vi "RTS Door Opener Setup.vi"(8 "Error In":errorcluster, 11 "Station Settings":T1) -> (0 "Error Out":errorcluster, 3 "Update Server Output":bool)   [LabVIEW 2020]
uses:
  Type Definitions/RTS Door Op Data.ctl
  Type Definitions/RTS Door Ops Client.ctl
  Type Definitions/RTS Door Opening Schedule.ctl
  Type Definitions/RTS Door Ops Sequence.ctl
  Type Definitions/RTS Standard Door Opening Test.ctl
  Type Definitions/RTS Station Settions TCP Comms.ctl
  Type Definitions/RTS Chamber Save Status.ctl
  Type Definitions/RTS Test Pattern.ctl
panel:
  out "Front Program Name":string
  in  "Update Server":bool
  in  "Tab Control 2":enum32{"Page 1", "Standard Test"}(tab)
  out "time stamp":timestamp
  out "Station":u16
  out "Chamber":u16
  out "Debug array":string[](array[string])
  in  "Debug":bool
  in  "ISO Energy Consumption":T4={"Chamber 1-3"=[], "Chamber 1-2"=[], "Chamber 1-1"=[{"End Time"=timestamp(0 s since 1904-01-01), "Start Time"=timestamp(0 s since 1904-01-01), "Door Opening Schedule:"={"Open Door Timer (s)"=0.0, "Delay Time (s)"=0.0, "Close Door Timer (s)"=0.0}, "Enable Door Ops"=FALSE, "Door Openings"=0, "Temp (°F)"=90.0, "Humidity (%)"=40.0, "Voltage (V)"=0.0, "Door Open Sequence:"=enum."", "Door Delay(sec)"=0.0, "Dehum (°F)"=0.0, "Cool (°F)"=0.0}], "Standard Tests 1-1"=enum."511-B304 ISO Energy Consumption"} {"Chamber 1-1"."Start Time" format="%<%X\n%x>T"; "Chamber 1-1"."End Time" format="%<%X\n%x>T"; "Chamber 1-2"."Start Time" format="%<%X\n%x>T"; "Chamber 1-2"."End Time" format="%<%X\n%x>T"; "Chamber 1-3"."Start Time" format="%<%X\n%x>T"; "Chamber 1-3"."End Time" format="%<%X\n%x>T"}
  in  "NDO":T4={"Chamber 1-3"=[], "Chamber 1-2"=[], "Chamber 1-1"=[{"End Time"=timestamp(0 s since 1904-01-01), "Start Time"=timestamp(0 s since 1904-01-01), "Door Opening Schedule:"={"Open Door Timer (s)"=0.0, "Delay Time (s)"=0.0, "Close Door Timer (s)"=0.0}, "Enable Door Ops"=FALSE, "Door Openings"=0, "Temp (°F)"=90.0, "Humidity (%)"=50.0, "Voltage (V)"=0.0, "Door Open Sequence:"=enum."", "Door Delay(sec)"=0.0, "Dehum (°F)"=0.0, "Cool (°F)"=0.0}], "Standard Tests 1-1"=enum."511-B100 No Door Opening (NDO)"} {"Chamber 1-1"."Start Time" format="%<%X\n%x>T"; "Chamber 1-1"."End Time" format="%<%X\n%x>T"; "Chamber 1-2"."Start Time" format="%<%X\n%x>T"; "Chamber 1-2"."End Time" format="%<%X\n%x>T"; "Chamber 1-3"."Start Time" format="%<%X\n%x>T"; "Chamber 1-3"."End Time" format="%<%X\n%x>T"}
  in  "Moisture Accumulation (511-C401)":T4={"Chamber 1-3"=[{"End Time"=timestamp(0 s since 1904-01-01), "Start Time"=timestamp(0 s since 1904-01-01), "Door Opening Schedule:"={"Open Door Timer (s)"=0.0, "Delay Time (s)"=0.0, "Close Door Timer (s)"=0.0}, "Enable Door Ops"=FALSE, "Door Openings"=0, "Temp (°F)"=78.0, "Humidity (%)"=83.0, "Voltage (V)"=120.0, "Door Open Sequence:"=enum."", "Door Delay(sec)"=0.0, "Dehum (°F)"=70.0, "Cool (°F)"=65.0}, {"End Time"=timestamp(0 s since 1904-01-01), "Start Time"=timestamp(0 s since 1904-01-01), "Door Opening Schedule:"={"Open Door Timer (s)"=6.0, "Delay Time (s)"=465.0, "Close Door Timer (s)"=6.0}, "Enable Door Ops"=TRUE, "Door Openings"=0, "Temp (°F)"=90.0, "Humidity (%)"=65.0, "Voltage (V)"=120.0, "Door Open Sequence:"=enum."", "Door Delay(sec)"=0.0, "Dehum (°F)"=84.0, "Cool (°F)"=85.0}, {"End Time"=timestamp(0 s since 1904-01-01), "Start Time"=timestamp(0 s since 1904-01-01), "Door Opening Schedule:"={"Open Door Timer (s)"=6.0, "Delay Time (s)"=465.0, "Close Door Timer (s)"=6.0}, "Enable Door Ops"=TRUE, "Door Openings"=0, "Temp (°F)"=78.0, "Humidity (%)"=83.0, "Voltage (V)"=120.0, "Door Open Sequence:"=enum."", "Door Delay(sec)"=0.0, "Dehum (°F)"=70.0, "Cool (°F)"=65.0}, {"End Time"=timestamp(0 s since 1904-01-01), "Start Time"=timestamp(0 s since 1904-01-01), "Door Opening Schedule:"={"Open Door Timer (s)"=0.0, "Delay Time (s)"=0.0, "Close Door Timer (s)"=0.0}, "Enable Door Ops"=FALSE, "Door Openings"=0, "Temp (°F)"=78.0, "Humidity (%)"=83.0, "Voltage (V)"=120.0, "Door Open Sequence:"=enum."", "Door Delay(sec)"=0.0, "Dehum (°F)"=70.0, "Cool (°F)"=65.0}, {"End Time"=timestamp(0 s since 1904-01-01), "Start Time"=timestamp(0 s since 1904-01-01), "Door Opening Schedule:"={"Open Door Timer (s)"=6.0, "Delay Time (s)"=465.0, "Close Door Timer (s)"=6.0}, "Enable Door Ops"=TRUE, "Door Openings"=0, "Temp (°F)"=90.0, "Humidity (%)"=65.0, "Voltage (V)"=120.0, "Door Open Sequence:"=enum."", "Door Delay(sec)"=0.0, "Dehum (°F)"=84.0, "Cool (°F)"=85.0}, {"End Time"=timestamp(0 s since 1904-01-01), "Start Time"=timestamp(0 s since 1904-01-01), "Door Opening Schedule:"={"Open Door Timer (s)"=6.0, "Delay Time (s)"=465.0, "Close Door Timer (s)"=6.0}, "Enable Door Ops"=TRUE, "Door Openings"=0, "Temp (°F)"=78.0, "Humidity (%)"=83.0, "Voltage (V)"=120.0, "Door Open Sequence:"=enum."", "Door Delay(sec)"=0.0, "Dehum (°F)"=70.0, "Cool (°F)"=65.0}, {"End Time"=timestamp(0 s since 1904-01-01), "Start Time"=timestamp(0 s since 1904-01-01), "Door Opening Schedule:"={"Open Door Timer (s)"=0.0, "Delay Time (s)"=0.0, "Close Door Timer (s)"=0.0}, "Enable Door Ops"=FALSE, "Door Openings"=0, "Temp (°F)"=78.0, "Humidity (%)"=83.0, "Voltage (V)"=120.0, "Door Open Sequence:"=enum."", "Door Delay(sec)"=0.0, "Dehum (°F)"=70.0, "Cool (°F)"=65.0}], "Chamber 1-2"=[{"End Time"=timestamp(0 s since 1904-01-01), "Start Time"=timestamp(0 s since 1904-01-01), "Door Opening Schedule:"={"Open Door Timer (s)"=0.0, "Delay Time (s)"=0.0, "Close Door Timer (s)"=0.0}, "Enable Door Ops"=FALSE, "Door Openings"=0, "Temp (°F)"=78.0, "Humidity (%)"=83.0, "Voltage (V)"=120.0, "Door Open Sequence:"=enum."", "Door Delay(sec)"=0.0, "Dehum (°F)"=70.0, "Cool (°F)"=65.0}, {"End Time"=timestamp(0 s since 1904-01-01), "Start Time"=timestamp(0 s since 1904-01-01), "Door Opening Schedule:"={"Open Door Timer (s)"=6.0, "Delay Time (s)"=465.0, "Close Door Timer (s)"=6.0}, "Enable Door Ops"=TRUE, "Door Openings"=0, "Temp (°F)"=90.0, "Humidity (%)"=65.0, "Voltage (V)"=120.0, "Door Open Sequence:"=enum."", "Door Delay(sec)"=0.0, "Dehum (°F)"=0.0, "Cool (°F)"=0.0}, {"End Time"=timestamp(0 s since 1904-01-01), "Start Time"=timestamp(0 s since 1904-01-01), "Door Opening Schedule:"={"Open Door Timer (s)"=6.0, "Delay Time (s)"=465.0, "Close Door Timer (s)"=6.0}, "Enable Door Ops"=TRUE, "Door Openings"=0, "Temp (°F)"=78.0, "Humidity (%)"=83.0, "Voltage (V)"=120.0, "Door Open Sequence:"=enum."", "Door Delay(sec)"=0.0, "Dehum (°F)"=70.0, "Cool (°F)"=65.0}, {"End Time"=timestamp(0 s since 1904-01-01), "Start Time"=timestamp(0 s since 1904-01-01), "Door Opening Schedule:"={"Open Door Timer (s)"=0.0, "Delay Time (s)"=0.0, "Close Door Timer (s)"=0.0}, "Enable Door Ops"=FALSE, "Door Openings"=0, "Temp (°F)"=78.0, "Humidity (%)"=83.0, "Voltage (V)"=120.0, "Door Open Sequence:"=enum."", "Door Delay(sec)"=0.0, "Dehum (°F)"=70.0, "Cool (°F)"=65.0}, {"End Time"=timestamp(0 s since 1904-01-01), "Start Time"=timestamp(0 s since 1904-01-01), "Door Opening Schedule:"={"Open Door Timer (s)"=6.0, "Delay Time (s)"=465.0, "Close Door Timer (s)"=6.0}, "Enable Door Ops"=TRUE, "Door Openings"=0, "Temp (°F)"=90.0, "Humidity (%)"=65.0, "Voltage (V)"=120.0, "Door Open Sequence:"=enum."", "Door Delay(sec)"=0.0, "Dehum (°F)"=84.0, "Cool (°F)"=85.0}, {"End Time"=timestamp(0 s since 1904-01-01), "Start Time"=timestamp(0 s since 1904-01-01), "Door Opening Schedule:"={"Open Door Timer (s)"=6.0, "Delay Time (s)"=465.0, "Close Door Timer (s)"=6.0}, "Enable Door Ops"=TRUE, "Door Openings"=0, "Temp (°F)"=78.0, "Humidity (%)"=83.0, "Voltage (V)"=120.0, "Door Open Sequence:"=enum."", "Door Delay(sec)"=0.0, "Dehum (°F)"=70.0, "Cool (°F)"=65.0}, {"End Time"=timestamp(0 s since 1904-01-01), "Start Time"=timestamp(0 s since 1904-01-01), "Door Opening Schedule:"={"Open Door Timer (s)"=0.0, "Delay Time (s)"=0.0, "Close Door Timer (s)"=0.0}, "Enable Door Ops"=FALSE, "Door Openings"=0, "Temp (°F)"=78.0, "Humidity (%)"=83.0, "Voltage (V)"=120.0, "Door Open Sequence:"=enum."", "Door Delay(sec)"=0.0, "Dehum (°F)"=70.0, "Cool (°F)"=65.0}], "Chamber 1-1"=[{"End Time"=timestamp(0 s since 1904-01-01), "Start Time"=timestamp(0 s since 1904-01-01), "Door Opening Schedule:"={"Open Door Timer (s)"=0.0, "Delay Time (s)"=0.0, "Close Door Timer (s)"=0.0}, "Enable Door Ops"=FALSE, "Door Openings"=0, "Temp (°F)"=78.0, "Humidity (%)"=83.0, "Voltage (V)"=120.0, "Door Open Sequence:"=enum."", "Door Delay(sec)"=0.0, "Dehum (°F)"=70.0, "Cool (°F)"=65.0}, {"End Time"=timestamp(0 s since 1904-01-01), "Start Time"=timestamp(0 s since 1904-01-01), "Door Opening Schedule:"={"Open Door Timer (s)"=6.0, "Delay Time (s)"=1850.0, "Close Door Timer (s)"=6.0}, "Enable Door Ops"=TRUE, "Door Openings"=0, "Temp (°F)"=90.0, "Humidity (%)"=65.0, "Voltage (V)"=120.0, "Door Open Sequence:"=enum."", "Door Delay(sec)"=0.0, "Dehum (°F)"=84.0, "Cool (°F)"=85.0}, {"End Time"=timestamp(0 s since 1904-01-01), "Start Time"=timestamp(0 s since 1904-01-01), "Door Opening Schedule:"={"Open Door Timer (s)"=6.0, "Delay Time (s)"=1850.0, "Close Door Timer (s)"=6.0}, "Enable Door Ops"=TRUE, "Door Openings"=0, "Temp (°F)"=78.0, "Humidity (%)"=83.0, "Voltage (V)"=120.0, "Door Open Sequence:"=enum."", "Door Delay(sec)"=0.0, "Dehum (°F)"=70.0, "Cool (°F)"=65.0}, {"End Time"=timestamp(0 s since 1904-01-01), "Start Time"=timestamp(0 s since 1904-01-01), "Door Opening Schedule:"={"Open Door Timer (s)"=0.0, "Delay Time (s)"=0.0, "Close Door Timer (s)"=0.0}, "Enable Door Ops"=FALSE, "Door Openings"=0, "Temp (°F)"=78.0, "Humidity (%)"=83.0, "Voltage (V)"=120.0, "Door Open Sequence:"=enum."", "Door Delay(sec)"=0.0, "Dehum (°F)"=70.0, "Cool (°F)"=65.0}, {"End Time"=timestamp(0 s since 1904-01-01), "Start Time"=timestamp(0 s since 1904-01-01), "Door Opening Schedule:"={"Open Door Timer (s)"=6.0, "Delay Time (s)"=1850.0, "Close Door Timer (s)"=6.0}, "Enable Door Ops"=TRUE, "Door Openings"=0, "Temp (°F)"=90.0, "Humidity (%)"=65.0, "Voltage (V)"=120.0, "Door Open Sequence:"=enum."", "Door Delay(sec)"=0.0, "Dehum (°F)"=84.0, "Cool (°F)"=85.0}, {"End Time"=timestamp(0 s since 1904-01-01), "Start Time"=timestamp(0 s since 1904-01-01), "Door Opening Schedule:"={"Open Door Timer (s)"=6.0, "Delay Time (s)"=1850.0, "Close Door Timer (s)"=6.0}, "Enable Door Ops"=TRUE, "Door Openings"=0, "Temp (°F)"=78.0, "Humidity (%)"=83.0, "Voltage (V)"=120.0, "Door Open Sequence:"=enum."", "Door Delay(sec)"=0.0, "Dehum (°F)"=70.0, "Cool (°F)"=65.0}, {"End Time"=timestamp(0 s since 1904-01-01), "Start Time"=timestamp(0 s since 1904-01-01), "Door Opening Schedule:"={"Open Door Timer (s)"=0.0, "Delay Time (s)"=0.0, "Close Door Timer (s)"=0.0}, "Enable Door Ops"=FALSE, "Door Openings"=0, "Temp (°F)"=78.0, "Humidity (%)"=83.0, "Voltage (V)"=120.0, "Door Open Sequence:"=enum."", "Door Delay(sec)"=0.0, "Dehum (°F)"=70.0, "Cool (°F)"=65.0}], "Standard Tests 1-1"=enum."511-C401 Moisture Accumulation"} {"Chamber 1-1"."Start Time" format="%<%X\n%x>T"; "Chamber 1-1"."End Time" format="%<%X\n%x>T"; "Chamber 1-2"."Start Time" format="%<%X\n%x>T"; "Chamber 1-2"."End Time" format="%<%X\n%x>T"; "Chamber 1-3"."Start Time" format="%<%X\n%x>T"; "Chamber 1-3"."End Time" format="%<%X\n%x>T"}
  in  "SLAT (512-C419)":T4={"Chamber 1-3"=[{"End Time"=timestamp(3594046716.8947463 s since 1904-01-01), "Start Time"=timestamp(3593614713.19836 s since 1904-01-01), "Door Opening Schedule:"={"Open Door Timer (s)"=12.0, "Delay Time (s)"=695.0, "Close Door Timer (s)"=12.0}, "Enable Door Ops"=FALSE, "Door Openings"=120, "Temp (°F)"=0.0, "Humidity (%)"=0.0, "Voltage (V)"=0.0, "Door Open Sequence:"=enum."", "Door Delay(sec)"=0.0, "Dehum (°F)"=0.0, "Cool (°F)"=0.0}], "Chamber 1-2"=[{"End Time"=timestamp(3594046708.565822 s since 1904-01-01), "Start Time"=timestamp(3593614700.612354 s since 1904-01-01), "Door Opening Schedule:"={"Open Door Timer (s)"=12.0, "Delay Time (s)"=695.0, "Close Door Timer (s)"=12.0}, "Enable Door Ops"=FALSE, "Door Openings"=0, "Temp (°F)"=0.0, "Humidity (%)"=0.0, "Voltage (V)"=0.0, "Door Open Sequence:"=enum."", "Door Delay(sec)"=0.0, "Dehum (°F)"=0.0, "Cool (°F)"=0.0}], "Chamber 1-1"=[{"End Time"=timestamp(3594046691.867131 s since 1904-01-01), "Start Time"=timestamp(3593614687.850203 s since 1904-01-01), "Door Opening Schedule:"={"Open Door Timer (s)"=12.0, "Delay Time (s)"=2800.0, "Close Door Timer (s)"=12.0}, "Enable Door Ops"=TRUE, "Door Openings"=30, "Temp (°F)"=0.0, "Humidity (%)"=0.0, "Voltage (V)"=0.0, "Door Open Sequence:"=enum."", "Door Delay(sec)"=0.0, "Dehum (°F)"=0.0, "Cool (°F)"=0.0}], "Standard Tests 1-1"=enum."512-C410 SLAT"} {"Chamber 1-1"."Start Time" format="%<%X\n%x>T"; "Chamber 1-1"."End Time" format="%<%X\n%x>T"; "Chamber 1-2"."Start Time" format="%<%X\n%x>T"; "Chamber 1-2"."End Time" format="%<%X\n%x>T"; "Chamber 1-3"."Start Time" format="%<%X\n%x>T"; "Chamber 1-3"."End Time" format="%<%X\n%x>T"}
  in  "HUT (511-B110)":T4={"Chamber 1-3"=[{"End Time"=timestamp(3594046716.8947463 s since 1904-01-01), "Start Time"=timestamp(3593614713.19836 s since 1904-01-01), "Door Opening Schedule:"={"Open Door Timer (s)"=0.0, "Delay Time (s)"=0.0, "Close Door Timer (s)"=0.0}, "Enable Door Ops"=FALSE, "Door Openings"=120, "Temp (°F)"=78.0, "Humidity (%)"=83.0, "Voltage (V)"=120.0, "Door Open Sequence:"=enum."", "Door Delay(sec)"=0.0, "Dehum (°F)"=70.0, "Cool (°F)"=65.0}, {"End Time"=timestamp(0 s since 1904-01-01), "Start Time"=timestamp(0 s since 1904-01-01), "Door Opening Schedule:"={"Open Door Timer (s)"=6.0, "Delay Time (s)"=465.0, "Close Door Timer (s)"=6.0}, "Enable Door Ops"=TRUE, "Door Openings"=0, "Temp (°F)"=90.0, "Humidity (%)"=65.0, "Voltage (V)"=120.0, "Door Open Sequence:"=enum."", "Door Delay(sec)"=0.0, "Dehum (°F)"=84.0, "Cool (°F)"=85.0}, {"End Time"=timestamp(0 s since 1904-01-01), "Start Time"=timestamp(0 s since 1904-01-01), "Door Opening Schedule:"={"Open Door Timer (s)"=6.0, "Delay Time (s)"=465.0, "Close Door Timer (s)"=6.0}, "Enable Door Ops"=TRUE, "Door Openings"=0, "Temp (°F)"=78.0, "Humidity (%)"=83.0, "Voltage (V)"=120.0, "Door Open Sequence:"=enum."", "Door Delay(sec)"=0.0, "Dehum (°F)"=70.0, "Cool (°F)"=65.0}, {"End Time"=timestamp(0 s since 1904-01-01), "Start Time"=timestamp(0 s since 1904-01-01), "Door Opening Schedule:"={"Open Door Timer (s)"=0.0, "Delay Time (s)"=0.0, "Close Door Timer (s)"=0.0}, "Enable Door Ops"=FALSE, "Door Openings"=0, "Temp (°F)"=78.0, "Humidity (%)"=83.0, "Voltage (V)"=120.0, "Door Open Sequence:"=enum."", "Door Delay(sec)"=0.0, "Dehum (°F)"=70.0, "Cool (°F)"=65.0}], "Chamber 1-2"=[{"End Time"=timestamp(3594046708.565822 s since 1904-01-01), "Start Time"=timestamp(3593614700.612354 s since 1904-01-01), "Door Opening Schedule:"={"Open Door Timer (s)"=0.0, "Delay Time (s)"=0.0, "Close Door Timer (s)"=0.0}, "Enable Door Ops"=FALSE, "Door Openings"=0, "Temp (°F)"=78.0, "Humidity (%)"=83.0, "Voltage (V)"=120.0, "Door Open Sequence:"=enum."", "Door Delay(sec)"=0.0, "Dehum (°F)"=70.0, "Cool (°F)"=65.0}, {"End Time"=timestamp(0 s since 1904-01-01), "Start Time"=timestamp(0 s since 1904-01-01), "Door Opening Schedule:"={"Open Door Timer (s)"=6.0, "Delay Time (s)"=465.0, "Close Door Timer (s)"=6.0}, "Enable Door Ops"=TRUE, "Door Openings"=0, "Temp (°F)"=90.0, "Humidity (%)"=65.0, "Voltage (V)"=120.0, "Door Open Sequence:"=enum."", "Door Delay(sec)"=0.0, "Dehum (°F)"=84.0, "Cool (°F)"=85.0}, {"End Time"=timestamp(0 s since 1904-01-01), "Start Time"=timestamp(0 s since 1904-01-01), "Door Opening Schedule:"={"Open Door Timer (s)"=6.0, "Delay Time (s)"=465.0, "Close Door Timer (s)"=6.0}, "Enable Door Ops"=TRUE, "Door Openings"=0, "Temp (°F)"=78.0, "Humidity (%)"=83.0, "Voltage (V)"=120.0, "Door Open Sequence:"=enum."", "Door Delay(sec)"=0.0, "Dehum (°F)"=70.0, "Cool (°F)"=65.0}, {"End Time"=timestamp(0 s since 1904-01-01), "Start Time"=timestamp(0 s since 1904-01-01), "Door Opening Schedule:"={"Open Door Timer (s)"=0.0, "Delay Time (s)"=0.0, "Close Door Timer (s)"=0.0}, "Enable Door Ops"=FALSE, "Door Openings"=0, "Temp (°F)"=78.0, "Humidity (%)"=83.0, "Voltage (V)"=120.0, "Door Open Sequence:"=enum."", "Door Delay(sec)"=0.0, "Dehum (°F)"=70.0, "Cool (°F)"=65.0}], "Chamber 1-1"=[{"End Time"=timestamp(3594046691.867131 s since 1904-01-01), "Start Time"=timestamp(3593614687.850203 s since 1904-01-01), "Door Opening Schedule:"={"Open Door Timer (s)"=0.0, "Delay Time (s)"=0.0, "Close Door Timer (s)"=0.0}, "Enable Door Ops"=FALSE, "Door Openings"=30, "Temp (°F)"=78.0, "Humidity (%)"=83.0, "Voltage (V)"=120.0, "Door Open Sequence:"=enum."", "Door Delay(sec)"=0.0, "Dehum (°F)"=70.0, "Cool (°F)"=65.0}, {"End Time"=timestamp(0 s since 1904-01-01), "Start Time"=timestamp(0 s since 1904-01-01), "Door Opening Schedule:"={"Open Door Timer (s)"=6.0, "Delay Time (s)"=1850.0, "Close Door Timer (s)"=6.0}, "Enable Door Ops"=TRUE, "Door Openings"=0, "Temp (°F)"=90.0, "Humidity (%)"=65.0, "Voltage (V)"=120.0, "Door Open Sequence:"=enum."", "Door Delay(sec)"=0.0, "Dehum (°F)"=84.0, "Cool (°F)"=85.0}, {"End Time"=timestamp(0 s since 1904-01-01), "Start Time"=timestamp(0 s since 1904-01-01), "Door Opening Schedule:"={"Open Door Timer (s)"=6.0, "Delay Time (s)"=1850.0, "Close Door Timer (s)"=6.0}, "Enable Door Ops"=TRUE, "Door Openings"=0, "Temp (°F)"=78.0, "Humidity (%)"=83.0, "Voltage (V)"=120.0, "Door Open Sequence:"=enum."", "Door Delay(sec)"=0.0, "Dehum (°F)"=70.0, "Cool (°F)"=65.0}, {"End Time"=timestamp(0 s since 1904-01-01), "Start Time"=timestamp(0 s since 1904-01-01), "Door Opening Schedule:"={"Open Door Timer (s)"=0.0, "Delay Time (s)"=0.0, "Close Door Timer (s)"=0.0}, "Enable Door Ops"=FALSE, "Door Openings"=0, "Temp (°F)"=78.0, "Humidity (%)"=83.0, "Voltage (V)"=120.0, "Door Open Sequence:"=enum."", "Door Delay(sec)"=0.0, "Dehum (°F)"=70.0, "Cool (°F)"=65.0}], "Standard Tests 1-1"=enum."511-B110 HUT"} {"Chamber 1-1"."Start Time" format="%<%X\n%x>T"; "Chamber 1-1"."End Time" format="%<%X\n%x>T"; "Chamber 1-2"."Start Time" format="%<%X\n%x>T"; "Chamber 1-2"."End Time" format="%<%X\n%x>T"; "Chamber 1-3"."Start Time" format="%<%X\n%x>T"; "Chamber 1-3"."End Time" format="%<%X\n%x>T"}
  in  "Internal Moisture Test (511-B111) - 5 Days":T4={"Chamber 1-3"=[{"End Time"=timestamp(3594046716.8947463 s since 1904-01-01), "Start Time"=timestamp(3593614713.19836 s since 1904-01-01), "Door Opening Schedule:"={"Open Door Timer (s)"=12.0, "Delay Time (s)"=695.0, "Close Door Timer (s)"=12.0}, "Enable Door Ops"=FALSE, "Door Openings"=120, "Temp (°F)"=78.0, "Humidity (%)"=83.0, "Voltage (V)"=120.0, "Door Open Sequence:"=enum."", "Door Delay(sec)"=0.0, "Dehum (°F)"=70.0, "Cool (°F)"=65.0}, {"End Time"=timestamp(0 s since 1904-01-01), "Start Time"=timestamp(0 s since 1904-01-01), "Door Opening Schedule:"={"Open Door Timer (s)"=6.0, "Delay Time (s)"=465.0, "Close Door Timer (s)"=6.0}, "Enable Door Ops"=TRUE, "Door Openings"=0, "Temp (°F)"=90.0, "Humidity (%)"=65.0, "Voltage (V)"=120.0, "Door Open Sequence:"=enum."", "Door Delay(sec)"=0.0, "Dehum (°F)"=84.0, "Cool (°F)"=85.0}, {"End Time"=timestamp(0 s since 1904-01-01), "Start Time"=timestamp(0 s since 1904-01-01), "Door Opening Schedule:"={"Open Door Timer (s)"=6.0, "Delay Time (s)"=465.0, "Close Door Timer (s)"=6.0}, "Enable Door Ops"=TRUE, "Door Openings"=0, "Temp (°F)"=78.0, "Humidity (%)"=83.0, "Voltage (V)"=120.0, "Door Open Sequence:"=enum."", "Door Delay(sec)"=0.0, "Dehum (°F)"=70.0, "Cool (°F)"=65.0}, {"End Time"=timestamp(0 s since 1904-01-01), "Start Time"=timestamp(0 s since 1904-01-01), "Door Opening Schedule:"={"Open Door Timer (s)"=0.0, "Delay Time (s)"=0.0, "Close Door Timer (s)"=0.0}, "Enable Door Ops"=FALSE, "Door Openings"=0, "Temp (°F)"=78.0, "Humidity (%)"=83.0, "Voltage (V)"=120.0, "Door Open Sequence:"=enum."", "Door Delay(sec)"=0.0, "Dehum (°F)"=70.0, "Cool (°F)"=65.0}, {"End Time"=timestamp(0 s since 1904-01-01), "Start Time"=timestamp(0 s since 1904-01-01), "Door Opening Schedule:"={"Open Door Timer (s)"=6.0, "Delay Time (s)"=465.0, "Close Door Timer (s)"=6.0}, "Enable Door Ops"=TRUE, "Door Openings"=0, "Temp (°F)"=90.0, "Humidity (%)"=65.0, "Voltage (V)"=120.0, "Door Open Sequence:"=enum."", "Door Delay(sec)"=0.0, "Dehum (°F)"=84.0, "Cool (°F)"=85.0}, {"End Time"=timestamp(0 s since 1904-01-01), "Start Time"=timestamp(0 s since 1904-01-01), "Door Opening Schedule:"={"Open Door Timer (s)"=6.0, "Delay Time (s)"=465.0, "Close Door Timer (s)"=6.0}, "Enable Door Ops"=TRUE, "Door Openings"=0, "Temp (°F)"=78.0, "Humidity (%)"=83.0, "Voltage (V)"=120.0, "Door Open Sequence:"=enum."", "Door Delay(sec)"=0.0, "Dehum (°F)"=70.0, "Cool (°F)"=65.0}, {"End Time"=timestamp(0 s since 1904-01-01), "Start Time"=timestamp(0 s since 1904-01-01), "Door Opening Schedule:"={"Open Door Timer (s)"=0.0, "Delay Time (s)"=0.0, "Close Door Timer (s)"=0.0}, "Enable Door Ops"=FALSE, "Door Openings"=0, "Temp (°F)"=78.0, "Humidity (%)"=83.0, "Voltage (V)"=120.0, "Door Open Sequence:"=enum."", "Door Delay(sec)"=0.0, "Dehum (°F)"=70.0, "Cool (°F)"=65.0}, {"End Time"=timestamp(0 s since 1904-01-01), "Start Time"=timestamp(0 s since 1904-01-01), "Door Opening Schedule:"={"Open Door Timer (s)"=6.0, "Delay Time (s)"=465.0, "Close Door Timer (s)"=6.0}, "Enable Door Ops"=TRUE, "Door Openings"=0, "Temp (°F)"=90.0, "Humidity (%)"=65.0, "Voltage (V)"=120.0, "Door Open Sequence:"=enum."", "Door Delay(sec)"=0.0, "Dehum (°F)"=84.0, "Cool (°F)"=85.0}, {"End Time"=timestamp(0 s since 1904-01-01), "Start Time"=timestamp(0 s since 1904-01-01), "Door Opening Schedule:"={"Open Door Timer (s)"=6.0, "Delay Time (s)"=465.0, "Close Door Timer (s)"=6.0}, "Enable Door Ops"=TRUE, "Door Openings"=0, "Temp (°F)"=78.0, "Humidity (%)"=83.0, "Voltage (V)"=120.0, "Door Open Sequence:"=enum."", "Door Delay(sec)"=0.0, "Dehum (°F)"=70.0, "Cool (°F)"=65.0}, {"End Time"=timestamp(0 s since 1904-01-01), "Start Time"=timestamp(0 s since 1904-01-01), "Door Opening Schedule:"={"Open Door Timer (s)"=0.0, "Delay Time (s)"=0.0, "Close Door Timer (s)"=0.0}, "Enable Door Ops"=FALSE, "Door Openings"=0, "Temp (°F)"=78.0, "Humidity (%)"=83.0, "Voltage (V)"=120.0, "Door Open Sequence:"=enum."", "Door Delay(sec)"=0.0, "Dehum (°F)"=70.0, "Cool (°F)"=65.0}, {"End Time"=timestamp(0 s since 1904-01-01), "Start Time"=timestamp(0 s since 1904-01-01), "Door Opening Schedule:"={"Open Door Timer (s)"=6.0, "Delay Time (s)"=465.0, "Close Door Timer (s)"=6.0}, "Enable Door Ops"=TRUE, "Door Openings"=0, "Temp (°F)"=90.0, "Humidity (%)"=65.0, "Voltage (V)"=120.0, "Door Open Sequence:"=enum."", "Door Delay(sec)"=0.0, "Dehum (°F)"=84.0, "Cool (°F)"=85.0}, {"End Time"=timestamp(0 s since 1904-01-01), "Start Time"=timestamp(0 s since 1904-01-01), "Door Opening Schedule:"={"Open Door Timer (s)"=6.0, "Delay Time (s)"=465.0, "Close Door Timer (s)"=6.0}, "Enable Door Ops"=TRUE, "Door Openings"=0, "Temp (°F)"=78.0, "Humidity (%)"=83.0, "Voltage (V)"=120.0, "Door Open Sequence:"=enum."", "Door Delay(sec)"=0.0, "Dehum (°F)"=70.0, "Cool (°F)"=65.0}, {"End Time"=timestamp(0 s since 1904-01-01), "Start Time"=timestamp(0 s since 1904-01-01), "Door Opening Schedule:"={"Open Door Timer (s)"=0.0, "Delay Time (s)"=0.0, "Close Door Timer (s)"=0.0}, "Enable Door Ops"=FALSE, "Door Openings"=0, "Temp (°F)"=78.0, "Humidity (%)"=83.0, "Voltage (V)"=120.0, "Door Open Sequence:"=enum."", "Door Delay(sec)"=0.0, "Dehum (°F)"=70.0, "Cool (°F)"=65.0}, {"End Time"=timestamp(0 s since 1904-01-01), "Start Time"=timestamp(0 s since 1904-01-01), "Door Opening Schedule:"={"Open Door Timer (s)"=6.0, "Delay Time (s)"=465.0, "Close Door Timer (s)"=6.0}, "Enable Door Ops"=TRUE, "Door Openings"=0, "Temp (°F)"=90.0, "Humidity (%)"=65.0, "Voltage (V)"=120.0, "Door Open Sequence:"=enum."", "Door Delay(sec)"=0.0, "Dehum (°F)"=84.0, "Cool (°F)"=85.0}, {"End Time"=timestamp(0 s since 1904-01-01), "Start Time"=timestamp(0 s since 1904-01-01), "Door Opening Schedule:"={"Open Door Timer (s)"=6.0, "Delay Time (s)"=465.0, "Close Door Timer (s)"=6.0}, "Enable Door Ops"=TRUE, "Door Openings"=0, "Temp (°F)"=78.0, "Humidity (%)"=83.0, "Voltage (V)"=120.0, "Door Open Sequence:"=enum."", "Door Delay(sec)"=0.0, "Dehum (°F)"=70.0, "Cool (°F)"=65.0}, {"End Time"=timestamp(0 s since 1904-01-01), "Start Time"=timestamp(0 s since 1904-01-01), "Door Opening Schedule:"={"Open Door Timer (s)"=0.0, "Delay Time (s)"=0.0, "Close Door Timer (s)"=0.0}, "Enable Door Ops"=FALSE, "Door Openings"=0, "Temp (°F)"=78.0, "Humidity (%)"=83.0, "Voltage (V)"=120.0, "Door Open Sequence:"=enum."", "Door Delay(sec)"=0.0, "Dehum (°F)"=70.0, "Cool (°F)"=65.0}], "Chamber 1-2"=[{"End Time"=timestamp(3594046708.565822 s since 1904-01-01), "Start Time"=timestamp(3593614700.612354 s since 1904-01-01), "Door Opening Schedule:"={"Open Door Timer (s)"=12.0, "Delay Time (s)"=695.0, "Close Door Timer (s)"=12.0}, "Enable Door Ops"=FALSE, "Door Openings"=0, "Temp (°F)"=78.0, "Humidity (%)"=83.0, "Voltage (V)"=120.0, "Door Open Sequence:"=enum."", "Door Delay(sec)"=0.0, "Dehum (°F)"=70.0, "Cool (°F)"=65.0}, {"End Time"=timestamp(0 s since 1904-01-01), "Start Time"=timestamp(0 s since 1904-01-01), "Door Opening Schedule:"={"Open Door Timer (s)"=6.0, "Delay Time (s)"=465.0, "Close Door Timer (s)"=6.0}, "Enable Door Ops"=TRUE, "Door Openings"=0, "Temp (°F)"=90.0, "Humidity (%)"=65.0, "Voltage (V)"=120.0, "Door Open Sequence:"=enum."", "Door Delay(sec)"=0.0, "Dehum (°F)"=84.0, "Cool (°F)"=85.0}, {"End Time"=timestamp(0 s since 1904-01-01), "Start Time"=timestamp(0 s since 1904-01-01), "Door Opening Schedule:"={"Open Door Timer (s)"=6.0, "Delay Time (s)"=465.0, "Close Door Timer (s)"=6.0}, "Enable Door Ops"=TRUE, "Door Openings"=0, "Temp (°F)"=78.0, "Humidity (%)"=83.0, "Voltage (V)"=120.0, "Door Open Sequence:"=enum."", "Door Delay(sec)"=0.0, "Dehum (°F)"=70.0, "Cool (°F)"=65.0}, {"End Time"=timestamp(0 s since 1904-01-01), "Start Time"=timestamp(0 s since 1904-01-01), "Door Opening Schedule:"={"Open Door Timer (s)"=0.0, "Delay Time (s)"=0.0, "Close Door Timer (s)"=0.0}, "Enable Door Ops"=FALSE, "Door Openings"=0, "Temp (°F)"=78.0, "Humidity (%)"=83.0, "Voltage (V)"=120.0, "Door Open Sequence:"=enum."", "Door Delay(sec)"=0.0, "Dehum (°F)"=70.0, "Cool (°F)"=65.0}, {"End Time"=timestamp(0 s since 1904-01-01), "Start Time"=timestamp(0 s since 1904-01-01), "Door Opening Schedule:"={"Open Door Timer (s)"=6.0, "Delay Time (s)"=465.0, "Close Door Timer (s)"=6.0}, "Enable Door Ops"=TRUE, "Door Openings"=0, "Temp (°F)"=90.0, "Humidity (%)"=65.0, "Voltage (V)"=120.0, "Door Open Sequence:"=enum."", "Door Delay(sec)"=0.0, "Dehum (°F)"=84.0, "Cool (°F)"=85.0}, {"End Time"=timestamp(0 s since 1904-01-01), "Start Time"=timestamp(0 s since 1904-01-01), "Door Opening Schedule:"={"Open Door Timer (s)"=6.0, "Delay Time (s)"=465.0, "Close Door Timer (s)"=6.0}, "Enable Door Ops"=TRUE, "Door Openings"=0, "Temp (°F)"=78.0, "Humidity (%)"=83.0, "Voltage (V)"=120.0, "Door Open Sequence:"=enum."", "Door Delay(sec)"=0.0, "Dehum (°F)"=70.0, "Cool (°F)"=65.0}, {"End Time"=timestamp(0 s since 1904-01-01), "Start Time"=timestamp(0 s since 1904-01-01), "Door Opening Schedule:"={"Open Door Timer (s)"=0.0, "Delay Time (s)"=0.0, "Close Door Timer (s)"=0.0}, "Enable Door Ops"=FALSE, "Door Openings"=0, "Temp (°F)"=78.0, "Humidity (%)"=83.0, "Voltage (V)"=120.0, "Door Open Sequence:"=enum."", "Door Delay(sec)"=0.0, "Dehum (°F)"=70.0, "Cool (°F)"=65.0}, {"End Time"=timestamp(0 s since 1904-01-01), "Start Time"=timestamp(0 s since 1904-01-01), "Door Opening Schedule:"={"Open Door Timer (s)"=6.0, "Delay Time (s)"=465.0, "Close Door Timer (s)"=6.0}, "Enable Door Ops"=TRUE, "Door Openings"=0, "Temp (°F)"=90.0, "Humidity (%)"=65.0, "Voltage (V)"=120.0, "Door Open Sequence:"=enum."", "Door Delay(sec)"=0.0, "Dehum (°F)"=84.0, "Cool (°F)"=85.0}, {"End Time"=timestamp(0 s since 1904-01-01), "Start Time"=timestamp(0 s since 1904-01-01), "Door Opening Schedule:"={"Open Door Timer (s)"=6.0, "Delay Time (s)"=465.0, "Close Door Timer (s)"=6.0}, "Enable Door Ops"=TRUE, "Door Openings"=0, "Temp (°F)"=78.0, "Humidity (%)"=83.0, "Voltage (V)"=120.0, "Door Open Sequence:"=enum."", "Door Delay(sec)"=0.0, "Dehum (°F)"=70.0, "Cool (°F)"=65.0}, {"End Time"=timestamp(0 s since 1904-01-01), "Start Time"=timestamp(0 s since 1904-01-01), "Door Opening Schedule:"={"Open Door Timer (s)"=0.0, "Delay Time (s)"=0.0, "Close Door Timer (s)"=0.0}, "Enable Door Ops"=FALSE, "Door Openings"=0, "Temp (°F)"=78.0, "Humidity (%)"=83.0, "Voltage (V)"=120.0, "Door Open Sequence:"=enum."", "Door Delay(sec)"=0.0, "Dehum (°F)"=70.0, "Cool (°F)"=65.0}, {"End Time"=timestamp(0 s since 1904-01-01), "Start Time"=timestamp(0 s since 1904-01-01), "Door Opening Schedule:"={"Open Door Timer (s)"=6.0, "Delay Time (s)"=465.0, "Close Door Timer (s)"=6.0}, "Enable Door Ops"=TRUE, "Door Openings"=0, "Temp (°F)"=90.0, "Humidity (%)"=65.0, "Voltage (V)"=120.0, "Door Open Sequence:"=enum."", "Door Delay(sec)"=0.0, "Dehum (°F)"=84.0, "Cool (°F)"=85.0}, {"End Time"=timestamp(0 s since 1904-01-01), "Start Time"=timestamp(0 s since 1904-01-01), "Door Opening Schedule:"={"Open Door Timer (s)"=6.0, "Delay Time (s)"=465.0, "Close Door Timer (s)"=6.0}, "Enable Door Ops"=TRUE, "Door Openings"=0, "Temp (°F)"=78.0, "Humidity (%)"=83.0, "Voltage (V)"=120.0, "Door Open Sequence:"=enum."", "Door Delay(sec)"=0.0, "Dehum (°F)"=70.0, "Cool (°F)"=65.0}, {"End Time"=timestamp(0 s since 1904-01-01), "Start Time"=timestamp(0 s since 1904-01-01), "Door Opening Schedule:"={"Open Door Timer (s)"=0.0, "Delay Time (s)"=0.0, "Close Door Timer (s)"=0.0}, "Enable Door Ops"=FALSE, "Door Openings"=0, "Temp (°F)"=78.0, "Humidity (%)"=83.0, "Voltage (V)"=120.0, "Door Open Sequence:"=enum."", "Door Delay(sec)"=0.0, "Dehum (°F)"=70.0, "Cool (°F)"=65.0}, {"End Time"=timestamp(0 s since 1904-01-01), "Start Time"=timestamp(0 s since 1904-01-01), "Door Opening Schedule:"={"Open Door Timer (s)"=6.0, "Delay Time (s)"=465.0, "Close Door Timer (s)"=6.0}, "Enable Door Ops"=TRUE, "Door Openings"=0, "Temp (°F)"=90.0, "Humidity (%)"=65.0, "Voltage (V)"=120.0, "Door Open Sequence:"=enum."", "Door Delay(sec)"=0.0, "Dehum (°F)"=84.0, "Cool (°F)"=85.0}, {"End Time"=timestamp(0 s since 1904-01-01), "Start Time"=timestamp(0 s since 1904-01-01), "Door Opening Schedule:"={"Open Door Timer (s)"=6.0, "Delay Time (s)"=465.0, "Close Door Timer (s)"=6.0}, "Enable Door Ops"=TRUE, "Door Openings"=0, "Temp (°F)"=78.0, "Humidity (%)"=83.0, "Voltage (V)"=120.0, "Door Open Sequence:"=enum."", "Door Delay(sec)"=0.0, "Dehum (°F)"=70.0, "Cool (°F)"=65.0}, {"End Time"=timestamp(0 s since 1904-01-01), "Start Time"=timestamp(0 s since 1904-01-01), "Door Opening Schedule:"={"Open Door Timer (s)"=0.0, "Delay Time (s)"=0.0, "Close Door Timer (s)"=0.0}, "Enable Door Ops"=FALSE, "Door Openings"=0, "Temp (°F)"=78.0, "Humidity (%)"=83.0, "Voltage (V)"=120.0, "Door Open Sequence:"=enum."", "Door Delay(sec)"=0.0, "Dehum (°F)"=70.0, "Cool (°F)"=65.0}], "Chamber 1-1"=[{"End Time"=timestamp(3594046691.867131 s since 1904-01-01), "Start Time"=timestamp(3593614687.850203 s since 1904-01-01), "Door Opening Schedule:"={"Open Door Timer (s)"=0.0, "Delay Time (s)"=0.0, "Close Door Timer (s)"=0.0}, "Enable Door Ops"=FALSE, "Door Openings"=0, "Temp (°F)"=78.0, "Humidity (%)"=83.0, "Voltage (V)"=120.0, "Door Open Sequence:"=enum."", "Door Delay(sec)"=0.0, "Dehum (°F)"=70.0, "Cool (°F)"=65.0}, {"End Time"=timestamp(0 s since 1904-01-01), "Start Time"=timestamp(0 s since 1904-01-01), "Door Opening Schedule:"={"Open Door Timer (s)"=6.0, "Delay Time (s)"=1850.0, "Close Door Timer (s)"=6.0}, "Enable Door Ops"=TRUE, "Door Openings"=0, "Temp (°F)"=90.0, "Humidity (%)"=65.0, "Voltage (V)"=120.0, "Door Open Sequence:"=enum."", "Door Delay(sec)"=0.0, "Dehum (°F)"=84.0, "Cool (°F)"=85.0}, {"End Time"=timestamp(0 s since 1904-01-01), "Start Time"=timestamp(0 s since 1904-01-01), "Door Opening Schedule:"={"Open Door Timer (s)"=6.0, "Delay Time (s)"=1850.0, "Close Door Timer (s)"=6.0}, "Enable Door Ops"=TRUE, "Door Openings"=0, "Temp (°F)"=78.0, "Humidity (%)"=83.0, "Voltage (V)"=120.0, "Door Open Sequence:"=enum."", "Door Delay(sec)"=0.0, "Dehum (°F)"=70.0, "Cool (°F)"=65.0}, {"End Time"=timestamp(0 s since 1904-01-01), "Start Time"=timestamp(0 s since 1904-01-01), "Door Opening Schedule:"={"Open Door Timer (s)"=0.0, "Delay Time (s)"=0.0, "Close Door Timer (s)"=0.0}, "Enable Door Ops"=FALSE, "Door Openings"=0, "Temp (°F)"=78.0, "Humidity (%)"=83.0, "Voltage (V)"=120.0, "Door Open Sequence:"=enum."", "Door Delay(sec)"=0.0, "Dehum (°F)"=70.0, "Cool (°F)"=65.0}, {"End Time"=timestamp(0 s since 1904-01-01), "Start Time"=timestamp(0 s since 1904-01-01), "Door Opening Schedule:"={"Open Door Timer (s)"=6.0, "Delay Time (s)"=1850.0, "Close Door Timer (s)"=6.0}, "Enable Door Ops"=TRUE, "Door Openings"=0, "Temp (°F)"=90.0, "Humidity (%)"=65.0, "Voltage (V)"=120.0, "Door Open Sequence:"=enum."", "Door Delay(sec)"=0.0, "Dehum (°F)"=84.0, "Cool (°F)"=85.0}, {"End Time"=timestamp(0 s since 1904-01-01), "Start Time"=timestamp(0 s since 1904-01-01), "Door Opening Schedule:"={"Open Door Timer (s)"=6.0, "Delay Time (s)"=1850.0, "Close Door Timer (s)"=6.0}, "Enable Door Ops"=TRUE, "Door Openings"=0, "Temp (°F)"=78.0, "Humidity (%)"=83.0, "Voltage (V)"=120.0, "Door Open Sequence:"=enum."", "Door Delay(sec)"=0.0, "Dehum (°F)"=70.0, "Cool (°F)"=65.0}, {"End Time"=timestamp(0 s since 1904-01-01), "Start Time"=timestamp(0 s since 1904-01-01), "Door Opening Schedule:"={"Open Door Timer (s)"=0.0, "Delay Time (s)"=0.0, "Close Door Timer (s)"=0.0}, "Enable Door Ops"=FALSE, "Door Openings"=0, "Temp (°F)"=78.0, "Humidity (%)"=83.0, "Voltage (V)"=120.0, "Door Open Sequence:"=enum."", "Door Delay(sec)"=0.0, "Dehum (°F)"=70.0, "Cool (°F)"=65.0}, {"End Time"=timestamp(0 s since 1904-01-01), "Start Time"=timestamp(0 s since 1904-01-01), "Door Opening Schedule:"={"Open Door Timer (s)"=6.0, "Delay Time (s)"=1850.0, "Close Door Timer (s)"=6.0}, "Enable Door Ops"=TRUE, "Door Openings"=0, "Temp (°F)"=90.0, "Humidity (%)"=65.0, "Voltage (V)"=120.0, "Door Open Sequence:"=enum."", "Door Delay(sec)"=0.0, "Dehum (°F)"=84.0, "Cool (°F)"=85.0}, {"End Time"=timestamp(0 s since 1904-01-01), "Start Time"=timestamp(0 s since 1904-01-01), "Door Opening Schedule:"={"Open Door Timer (s)"=6.0, "Delay Time (s)"=1850.0, "Close Door Timer (s)"=6.0}, "Enable Door Ops"=TRUE, "Door Openings"=0, "Temp (°F)"=78.0, "Humidity (%)"=83.0, "Voltage (V)"=120.0, "Door Open Sequence:"=enum."", "Door Delay(sec)"=0.0, "Dehum (°F)"=70.0, "Cool (°F)"=65.0}, {"End Time"=timestamp(0 s since 1904-01-01), "Start Time"=timestamp(0 s since 1904-01-01), "Door Opening Schedule:"={"Open Door Timer (s)"=0.0, "Delay Time (s)"=0.0, "Close Door Timer (s)"=0.0}, "Enable Door Ops"=FALSE, "Door Openings"=0, "Temp (°F)"=78.0, "Humidity (%)"=83.0, "Voltage (V)"=120.0, "Door Open Sequence:"=enum."", "Door Delay(sec)"=0.0, "Dehum (°F)"=70.0, "Cool (°F)"=65.0}, {"End Time"=timestamp(0 s since 1904-01-01), "Start Time"=timestamp(0 s since 1904-01-01), "Door Opening Schedule:"={"Open Door Timer (s)"=6.0, "Delay Time (s)"=1850.0, "Close Door Timer (s)"=6.0}, "Enable Door Ops"=TRUE, "Door Openings"=0, "Temp (°F)"=90.0, "Humidity (%)"=65.0, "Voltage (V)"=120.0, "Door Open Sequence:"=enum."", "Door Delay(sec)"=0.0, "Dehum (°F)"=84.0, "Cool (°F)"=85.0}, {"End Time"=timestamp(0 s since 1904-01-01), "Start Time"=timestamp(0 s since 1904-01-01), "Door Opening Schedule:"={"Open Door Timer (s)"=6.0, "Delay Time (s)"=1850.0, "Close Door Timer (s)"=6.0}, "Enable Door Ops"=TRUE, "Door Openings"=0, "Temp (°F)"=78.0, "Humidity (%)"=83.0, "Voltage (V)"=120.0, "Door Open Sequence:"=enum."", "Door Delay(sec)"=0.0, "Dehum (°F)"=70.0, "Cool (°F)"=65.0}, {"End Time"=timestamp(0 s since 1904-01-01), "Start Time"=timestamp(0 s since 1904-01-01), "Door Opening Schedule:"={"Open Door Timer (s)"=0.0, "Delay Time (s)"=0.0, "Close Door Timer (s)"=0.0}, "Enable Door Ops"=FALSE, "Door Openings"=0, "Temp (°F)"=78.0, "Humidity (%)"=83.0, "Voltage (V)"=120.0, "Door Open Sequence:"=enum."", "Door Delay(sec)"=0.0, "Dehum (°F)"=70.0, "Cool (°F)"=65.0}, {"End Time"=timestamp(0 s since 1904-01-01), "Start Time"=timestamp(0 s since 1904-01-01), "Door Opening Schedule:"={"Open Door Timer (s)"=6.0, "Delay Time (s)"=1850.0, "Close Door Timer (s)"=6.0}, "Enable Door Ops"=TRUE, "Door Openings"=0, "Temp (°F)"=90.0, "Humidity (%)"=65.0, "Voltage (V)"=120.0, "Door Open Sequence:"=enum."", "Door Delay(sec)"=0.0, "Dehum (°F)"=84.0, "Cool (°F)"=85.0}, {"End Time"=timestamp(0 s since 1904-01-01), "Start Time"=timestamp(0 s since 1904-01-01), "Door Opening Schedule:"={"Open Door Timer (s)"=6.0, "Delay Time (s)"=4850.0, "Close Door Timer (s)"=6.0}, "Enable Door Ops"=TRUE, "Door Openings"=0, "Temp (°F)"=78.0, "Humidity (%)"=83.0, "Voltage (V)"=120.0, "Door Open Sequence:"=enum."", "Door Delay(sec)"=0.0, "Dehum (°F)"=70.0, "Cool (°F)"=65.0}, {"End Time"=timestamp(0 s since 1904-01-01), "Start Time"=timestamp(0 s since 1904-01-01), "Door Opening Schedule:"={"Open Door Timer (s)"=0.0, "Delay Time (s)"=0.0, "Close Door Timer (s)"=0.0}, "Enable Door Ops"=FALSE, "Door Openings"=0, "Temp (°F)"=78.0, "Humidity (%)"=83.0, "Voltage (V)"=120.0, "Door Open Sequence:"=enum."", "Door Delay(sec)"=0.0, "Dehum (°F)"=70.0, "Cool (°F)"=65.0}], "Standard Tests 1-1"=enum."511-B111 Internal Moisture"} {"Chamber 1-1"."Start Time" format="%<%X\n%x>T"; "Chamber 1-1"."End Time" format="%<%X\n%x>T"; "Chamber 1-2"."Start Time" format="%<%X\n%x>T"; "Chamber 1-2"."End Time" format="%<%X\n%x>T"; "Chamber 1-3"."Start Time" format="%<%X\n%x>T"; "Chamber 1-3"."End Time" format="%<%X\n%x>T"}
  in  "EHUT (511-B113)":T4 {"Chamber 1-1"."Start Time" format="%<%X\n%x>T"; "Chamber 1-1"."End Time" format="%<%X\n%x>T"; "Chamber 1-2"."Start Time" format="%<%X\n%x>T"; "Chamber 1-2"."End Time" format="%<%X\n%x>T"; "Chamber 1-3"."Start Time" format="%<%X\n%x>T"; "Chamber 1-3"."End Time" format="%<%X\n%x>T"}
  in  "Tab Control":T9(tab)
  in  "Chamber 1 Tab":T10(tab)
  in  "1-1":T4 {"Chamber 1-1"."Start Time" format="%<%X\n%x>T"; "Chamber 1-1"."End Time" format="%<%X\n%x>T"; "Chamber 1-2"."Start Time" format="%<%X\n%x>T"; "Chamber 1-2"."End Time" format="%<%X\n%x>T"; "Chamber 1-3"."Start Time" format="%<%X\n%x>T"; "Chamber 1-3"."End Time" format="%<%X\n%x>T"}
  in  "1-2":T4 {"Chamber 1-1"."Start Time" format="%<%X\n%x>T"; "Chamber 1-1"."End Time" format="%<%X\n%x>T"; "Chamber 1-2"."Start Time" format="%<%X\n%x>T"; "Chamber 1-2"."End Time" format="%<%X\n%x>T"; "Chamber 1-3"."Start Time" format="%<%X\n%x>T"; "Chamber 1-3"."End Time" format="%<%X\n%x>T"}
  in  "1-3":T4 {"Chamber 1-1"."Start Time" format="%<%X\n%x>T"; "Chamber 1-1"."End Time" format="%<%X\n%x>T"; "Chamber 1-2"."Start Time" format="%<%X\n%x>T"; "Chamber 1-2"."End Time" format="%<%X\n%x>T"; "Chamber 1-3"."Start Time" format="%<%X\n%x>T"; "Chamber 1-3"."End Time" format="%<%X\n%x>T"}
  in  "1-4":T4 {"Chamber 1-1"."Start Time" format="%<%X\n%x>T"; "Chamber 1-1"."End Time" format="%<%X\n%x>T"; "Chamber 1-2"."Start Time" format="%<%X\n%x>T"; "Chamber 1-2"."End Time" format="%<%X\n%x>T"; "Chamber 1-3"."Start Time" format="%<%X\n%x>T"; "Chamber 1-3"."End Time" format="%<%X\n%x>T"}
  in  "1-5":T4 {"Chamber 1-1"."Start Time" format="%<%X\n%x>T"; "Chamber 1-1"."End Time" format="%<%X\n%x>T"; "Chamber 1-2"."Start Time" format="%<%X\n%x>T"; "Chamber 1-2"."End Time" format="%<%X\n%x>T"; "Chamber 1-3"."Start Time" format="%<%X\n%x>T"; "Chamber 1-3"."End Time" format="%<%X\n%x>T"}
  in  "1-6":T4 {"Chamber 1-1"."Start Time" format="%<%X\n%x>T"; "Chamber 1-1"."End Time" format="%<%X\n%x>T"; "Chamber 1-2"."Start Time" format="%<%X\n%x>T"; "Chamber 1-2"."End Time" format="%<%X\n%x>T"; "Chamber 1-3"."Start Time" format="%<%X\n%x>T"; "Chamber 1-3"."End Time" format="%<%X\n%x>T"}
  in  "1-7":T4 {"Chamber 1-1"."Start Time" format="%<%X\n%x>T"; "Chamber 1-1"."End Time" format="%<%X\n%x>T"; "Chamber 1-2"."Start Time" format="%<%X\n%x>T"; "Chamber 1-2"."End Time" format="%<%X\n%x>T"; "Chamber 1-3"."Start Time" format="%<%X\n%x>T"; "Chamber 1-3"."End Time" format="%<%X\n%x>T"}
  in  "1-8":T4 {"Chamber 1-1"."Start Time" format="%<%X\n%x>T"; "Chamber 1-1"."End Time" format="%<%X\n%x>T"; "Chamber 1-2"."Start Time" format="%<%X\n%x>T"; "Chamber 1-2"."End Time" format="%<%X\n%x>T"; "Chamber 1-3"."Start Time" format="%<%X\n%x>T"; "Chamber 1-3"."End Time" format="%<%X\n%x>T"}
  in  "Chamber 2 Tab":T10(tab)
  in  "2-1":T4 {"Chamber 1-1"."Start Time" format="%<%X\n%x>T"; "Chamber 1-1"."End Time" format="%<%X\n%x>T"; "Chamber 1-2"."Start Time" format="%<%X\n%x>T"; "Chamber 1-2"."End Time" format="%<%X\n%x>T"; "Chamber 1-3"."Start Time" format="%<%X\n%x>T"; "Chamber 1-3"."End Time" format="%<%X\n%x>T"}
  in  "2-2":T4 {"Chamber 1-1"."Start Time" format="%<%X\n%x>T"; "Chamber 1-1"."End Time" format="%<%X\n%x>T"; "Chamber 1-2"."Start Time" format="%<%X\n%x>T"; "Chamber 1-2"."End Time" format="%<%X\n%x>T"; "Chamber 1-3"."Start Time" format="%<%X\n%x>T"; "Chamber 1-3"."End Time" format="%<%X\n%x>T"}
  in  "2-3":T4 {"Chamber 1-1"."Start Time" format="%<%X\n%x>T"; "Chamber 1-1"."End Time" format="%<%X\n%x>T"; "Chamber 1-2"."Start Time" format="%<%X\n%x>T"; "Chamber 1-2"."End Time" format="%<%X\n%x>T"; "Chamber 1-3"."Start Time" format="%<%X\n%x>T"; "Chamber 1-3"."End Time" format="%<%X\n%x>T"}
  in  "2-4":T4 {"Chamber 1-1"."Start Time" format="%<%X\n%x>T"; "Chamber 1-1"."End Time" format="%<%X\n%x>T"; "Chamber 1-2"."Start Time" format="%<%X\n%x>T"; "Chamber 1-2"."End Time" format="%<%X\n%x>T"; "Chamber 1-3"."Start Time" format="%<%X\n%x>T"; "Chamber 1-3"."End Time" format="%<%X\n%x>T"}
  in  "2-5":T4 {"Chamber 1-1"."Start Time" format="%<%X\n%x>T"; "Chamber 1-1"."End Time" format="%<%X\n%x>T"; "Chamber 1-2"."Start Time" format="%<%X\n%x>T"; "Chamber 1-2"."End Time" format="%<%X\n%x>T"; "Chamber 1-3"."Start Time" format="%<%X\n%x>T"; "Chamber 1-3"."End Time" format="%<%X\n%x>T"}
  in  "2-6":T4 {"Chamber 1-1"."Start Time" format="%<%X\n%x>T"; "Chamber 1-1"."End Time" format="%<%X\n%x>T"; "Chamber 1-2"."Start Time" format="%<%X\n%x>T"; "Chamber 1-2"."End Time" format="%<%X\n%x>T"; "Chamber 1-3"."Start Time" format="%<%X\n%x>T"; "Chamber 1-3"."End Time" format="%<%X\n%x>T"}
  in  "2-7":T4 {"Chamber 1-1"."Start Time" format="%<%X\n%x>T"; "Chamber 1-1"."End Time" format="%<%X\n%x>T"; "Chamber 1-2"."Start Time" format="%<%X\n%x>T"; "Chamber 1-2"."End Time" format="%<%X\n%x>T"; "Chamber 1-3"."Start Time" format="%<%X\n%x>T"; "Chamber 1-3"."End Time" format="%<%X\n%x>T"}
  in  "2-8":T4 {"Chamber 1-1"."Start Time" format="%<%X\n%x>T"; "Chamber 1-1"."End Time" format="%<%X\n%x>T"; "Chamber 1-2"."Start Time" format="%<%X\n%x>T"; "Chamber 1-2"."End Time" format="%<%X\n%x>T"; "Chamber 1-3"."Start Time" format="%<%X\n%x>T"; "Chamber 1-3"."End Time" format="%<%X\n%x>T"}
  in  "Chamber 3 Tab":T10(tab)
  in  "3-1":T4 {"Chamber 1-1"."Start Time" format="%<%X\n%x>T"; "Chamber 1-1"."End Time" format="%<%X\n%x>T"; "Chamber 1-2"."Start Time" format="%<%X\n%x>T"; "Chamber 1-2"."End Time" format="%<%X\n%x>T"; "Chamber 1-3"."Start Time" format="%<%X\n%x>T"; "Chamber 1-3"."End Time" format="%<%X\n%x>T"}
  in  "3-2":T4 {"Chamber 1-1"."Start Time" format="%<%X\n%x>T"; "Chamber 1-1"."End Time" format="%<%X\n%x>T"; "Chamber 1-2"."Start Time" format="%<%X\n%x>T"; "Chamber 1-2"."End Time" format="%<%X\n%x>T"; "Chamber 1-3"."Start Time" format="%<%X\n%x>T"; "Chamber 1-3"."End Time" format="%<%X\n%x>T"}
  in  "3-3":T4 {"Chamber 1-1"."Start Time" format="%<%X\n%x>T"; "Chamber 1-1"."End Time" format="%<%X\n%x>T"; "Chamber 1-2"."Start Time" format="%<%X\n%x>T"; "Chamber 1-2"."End Time" format="%<%X\n%x>T"; "Chamber 1-3"."Start Time" format="%<%X\n%x>T"; "Chamber 1-3"."End Time" format="%<%X\n%x>T"}
  in  "3-4":T4 {"Chamber 1-1"."Start Time" format="%<%X\n%x>T"; "Chamber 1-1"."End Time" format="%<%X\n%x>T"; "Chamber 1-2"."Start Time" format="%<%X\n%x>T"; "Chamber 1-2"."End Time" format="%<%X\n%x>T"; "Chamber 1-3"."Start Time" format="%<%X\n%x>T"; "Chamber 1-3"."End Time" format="%<%X\n%x>T"}
  in  "3-5":T4 {"Chamber 1-1"."Start Time" format="%<%X\n%x>T"; "Chamber 1-1"."End Time" format="%<%X\n%x>T"; "Chamber 1-2"."Start Time" format="%<%X\n%x>T"; "Chamber 1-2"."End Time" format="%<%X\n%x>T"; "Chamber 1-3"."Start Time" format="%<%X\n%x>T"; "Chamber 1-3"."End Time" format="%<%X\n%x>T"}
  in  "3-6":T4 {"Chamber 1-1"."Start Time" format="%<%X\n%x>T"; "Chamber 1-1"."End Time" format="%<%X\n%x>T"; "Chamber 1-2"."Start Time" format="%<%X\n%x>T"; "Chamber 1-2"."End Time" format="%<%X\n%x>T"; "Chamber 1-3"."Start Time" format="%<%X\n%x>T"; "Chamber 1-3"."End Time" format="%<%X\n%x>T"}
  in  "3-7":T4 {"Chamber 1-1"."Start Time" format="%<%X\n%x>T"; "Chamber 1-1"."End Time" format="%<%X\n%x>T"; "Chamber 1-2"."Start Time" format="%<%X\n%x>T"; "Chamber 1-2"."End Time" format="%<%X\n%x>T"; "Chamber 1-3"."Start Time" format="%<%X\n%x>T"; "Chamber 1-3"."End Time" format="%<%X\n%x>T"}
  in  "3-8":T4 {"Chamber 1-1"."Start Time" format="%<%X\n%x>T"; "Chamber 1-1"."End Time" format="%<%X\n%x>T"; "Chamber 1-2"."Start Time" format="%<%X\n%x>T"; "Chamber 1-2"."End Time" format="%<%X\n%x>T"; "Chamber 1-3"."Start Time" format="%<%X\n%x>T"; "Chamber 1-3"."End Time" format="%<%X\n%x>T"}
  in  "Chamber 4 Tab":T10(tab)
  in  "4-1":T4 {"Chamber 1-1"."Start Time" format="%<%X\n%x>T"; "Chamber 1-1"."End Time" format="%<%X\n%x>T"; "Chamber 1-2"."Start Time" format="%<%X\n%x>T"; "Chamber 1-2"."End Time" format="%<%X\n%x>T"; "Chamber 1-3"."Start Time" format="%<%X\n%x>T"; "Chamber 1-3"."End Time" format="%<%X\n%x>T"}
  in  "4-2":T4 {"Chamber 1-1"."Start Time" format="%<%X\n%x>T"; "Chamber 1-1"."End Time" format="%<%X\n%x>T"; "Chamber 1-2"."Start Time" format="%<%X\n%x>T"; "Chamber 1-2"."End Time" format="%<%X\n%x>T"; "Chamber 1-3"."Start Time" format="%<%X\n%x>T"; "Chamber 1-3"."End Time" format="%<%X\n%x>T"}
  in  "4-3":T4 {"Chamber 1-1"."Start Time" format="%<%X\n%x>T"; "Chamber 1-1"."End Time" format="%<%X\n%x>T"; "Chamber 1-2"."Start Time" format="%<%X\n%x>T"; "Chamber 1-2"."End Time" format="%<%X\n%x>T"; "Chamber 1-3"."Start Time" format="%<%X\n%x>T"; "Chamber 1-3"."End Time" format="%<%X\n%x>T"}
  in  "4-4":T4 {"Chamber 1-1"."Start Time" format="%<%X\n%x>T"; "Chamber 1-1"."End Time" format="%<%X\n%x>T"; "Chamber 1-2"."Start Time" format="%<%X\n%x>T"; "Chamber 1-2"."End Time" format="%<%X\n%x>T"; "Chamber 1-3"."Start Time" format="%<%X\n%x>T"; "Chamber 1-3"."End Time" format="%<%X\n%x>T"}
  in  "4-5":T4 {"Chamber 1-1"."Start Time" format="%<%X\n%x>T"; "Chamber 1-1"."End Time" format="%<%X\n%x>T"; "Chamber 1-2"."Start Time" format="%<%X\n%x>T"; "Chamber 1-2"."End Time" format="%<%X\n%x>T"; "Chamber 1-3"."Start Time" format="%<%X\n%x>T"; "Chamber 1-3"."End Time" format="%<%X\n%x>T"}
  in  "4-6":T4 {"Chamber 1-1"."Start Time" format="%<%X\n%x>T"; "Chamber 1-1"."End Time" format="%<%X\n%x>T"; "Chamber 1-2"."Start Time" format="%<%X\n%x>T"; "Chamber 1-2"."End Time" format="%<%X\n%x>T"; "Chamber 1-3"."Start Time" format="%<%X\n%x>T"; "Chamber 1-3"."End Time" format="%<%X\n%x>T"}
  in  "4-7":T4 {"Chamber 1-1"."Start Time" format="%<%X\n%x>T"; "Chamber 1-1"."End Time" format="%<%X\n%x>T"; "Chamber 1-2"."Start Time" format="%<%X\n%x>T"; "Chamber 1-2"."End Time" format="%<%X\n%x>T"; "Chamber 1-3"."Start Time" format="%<%X\n%x>T"; "Chamber 1-3"."End Time" format="%<%X\n%x>T"}
  in  "4-8":T4 {"Chamber 1-1"."Start Time" format="%<%X\n%x>T"; "Chamber 1-1"."End Time" format="%<%X\n%x>T"; "Chamber 1-2"."Start Time" format="%<%X\n%x>T"; "Chamber 1-2"."End Time" format="%<%X\n%x>T"; "Chamber 1-3"."Start Time" format="%<%X\n%x>T"; "Chamber 1-3"."End Time" format="%<%X\n%x>T"}
  # "Freezer"
  # "Cab"
  # "Slide"
  # "Freezer"
  # "Cab"
  # "Slide"
  # "Chamber Conditions:"
  # "Chamber Conditions:"
  # "Chamber Conditions:"
  # "Freezer"
  # "Cab"
  # "Slide"
  # "Chamber Conditions:"
  # "Chamber Conditions:"
  # "Chamber Conditions:"
  # "Freezer"
  # "Cab"
  # "Slide"
  # "Chamber Conditions:"
  # "Chamber Conditions:"
  # "Chamber Conditions:"
  # "Freezer"
  # "Cab"
  # "Slide"
  # "Chamber Conditions:"
  # "Chamber Conditions:"
  # "Chamber Conditions:"
  # "Freezer"
  # "Cab"
  # "Slide"
  # "Chamber Conditions:"
  # "Chamber Conditions:"
  # "Chamber Conditions:"
  # "Freezer"
  # "Cab"
  # "Slide"
  # "Chamber Conditions:"
  # "Chamber Conditions:"
  # "Chamber Conditions:"
  # "Chamber Conditions:"
  # "Chamber Conditions:"
  # "Chamber Conditions:"
  # "Station 1-1 Freezer"
  # "Station 1-1 Cab"
  # "Station 1-1 Slide"
  # "Chamber Conditions:"
  # "Chamber Conditions:"
  # "Chamber Conditions:"
  # "Station 1-2 Freezer"
  # "Station 1-2 Cab"
  # "Station 1-2 Slide"
  # "Chamber Conditions:"
  # "Chamber Conditions:"
  # "Chamber Conditions:"
  # "Station 1-3 Freezer"
  # "Station 1-3 Cab"
  # "Station 1-3 Slide"
  # "Chamber Conditions:"
  # "Chamber Conditions:"
  # "Chamber Conditions:"
  # "Station 1-4 Freezer"
  # "Station 1-4 Cab"
  # "Station 1-4 Slide"
  # "Chamber Conditions:"
  # "Chamber Conditions:"
  # "Chamber Conditions:"
  # "Station 1-5 Freezer"
  # "Station 1-5 Cab"
  # "Station 1-5 Slide"
  # "Chamber Conditions:"
  # "Chamber Conditions:"
  # "Chamber Conditions:"
  # "Station 1-6 Freezer"
  # "Station 1-6 Cab"
  # "Station 1-6 Slide"
  # "Chamber Conditions:"
  # "Chamber Conditions:"
  # "Chamber Conditions:"
  # "Station 1-7 Freezer"
  # "Station 1-7 Cab"
  # "Station 1-7 Slide"
  # "Chamber Conditions:"
  # "Chamber Conditions:"
  # "Chamber Conditions:"
  # "Station 1-8 Freezer"
  # "Station 1-8 Cab"
  # "Station 1-8 Slide"
  # "Chamber Conditions:"
  # "Chamber Conditions:"
  # "Chamber Conditions:"
  # "Station 2-1 Freezer"
  # "Station 2-1 Cab"
  # "Station 2-1 Slide"
  # "Chamber Conditions:"
  # "Chamber Conditions:"
  # "Chamber Conditions:"
  # "Station 2-2 Freezer"
  # "Station 2-2 Cab"
  # "Station 2-2 Slide"
  # "Chamber Conditions:"
  # "Chamber Conditions:"
  # "Chamber Conditions:"
  # "Station 2-3 Freezer"
  # "Station 2-3 Cab"
  # "Station 2-3 Slide"
  # "Chamber Conditions:"
  # "Chamber Conditions:"
  # "Chamber Conditions:"
  # "Station 2-4 Freezer"
  # "Station 2-4 Cab"
  # "Station 2-4 Slide"
  # "Chamber Conditions:"
  # "Chamber Conditions:"
  # "Chamber Conditions:"
  # "Station 2-5 Freezer"
  # "Station 2-5 Cab"
  # "Station 2-5 Slide"
  # "Chamber Conditions:"
  # "Chamber Conditions:"
  # "Chamber Conditions:"
  # "Station 2-6 Freezer"
  # "Station 2-6 Cab"
  # "Station 2-6 Slide"
  # "Chamber Conditions:"
  # "Chamber Conditions:"
  # "Chamber Conditions:"
  # "Station 2-7 Freezer"
  # "Station 2-7 Cab"
  # "Station 2-7 Slide"
  # "Chamber Conditions:"
  # "Chamber Conditions:"
  # "Chamber Conditions:"
  # "Station 2-8 Freezer"
  # "Station 2-8 Cab"
  # "Station 2-8 Slide"
  # "Chamber Conditions:"
  # "Chamber Conditions:"
  # "Chamber Conditions:"
  # "Station 3-1 Freezer"
  # "Station 3-1 Cab"
  # "Station 3-1 Slide"
  # "Chamber Conditions:"
  # "Chamber Conditions:"
  # "Chamber Conditions:"
  # "Station 3-2 Freezer"
  # "Station 3-2 Cab"
  # "Station 3-2 Slide"
  # "Chamber Conditions:"
  # "Chamber Conditions:"
  # "Chamber Conditions:"
  # "Station 3-3 Freezer"
  # "Station 3-3 Cab"
  # "Station 3-3 Slide"
  # "Chamber Conditions:"
  # "Chamber Conditions:"
  # "Chamber Conditions:"
  # "Station 3-4 Freezer"
  # "Station 3-4 Cab"
  # "Station 3-4 Slide"
  # "Chamber Conditions:"
  # "Chamber Conditions:"
  # "Chamber Conditions:"
  # "Station 3-5 Freezer"
  # "Station 3-5 Cab"
  # "Station 3-5 Slide"
  # "Chamber Conditions:"
  # "Chamber Conditions:"
  # "Chamber Conditions:"
  # "Station 3-6 Freezer"
  # "Station 3-6 Cab"
  # "Station 3-6 Slide"
  # "Chamber Conditions:"
  # "Chamber Conditions:"
  # "Chamber Conditions:"
  # "Station 3-7 Freezer"
  # "Station 3-7 Cab"
  # "Station 3-7 Slide"
  # "Chamber Conditions:"
  # "Chamber Conditions:"
  # "Chamber Conditions:"
  # "Station 3-8 Freezer"
  # "Station 3-8 Cab"
  # "Station 3-8 Slide"
  # "Chamber Conditions:"
  # "Chamber Conditions:"
  # "Chamber Conditions:"
  # "Station 4-1 Freezer"
  # "Station 4-1 Cab"
  # "Station 4-1 Slide"
  # "Chamber Conditions:"
  # "Chamber Conditions:"
  # "Chamber Conditions:"
  # "Station 4-2 Freezer"
  # "Station 4-2 Cab"
  # "Station 4-2 Slide"
  # "Chamber Conditions:"
  # "Chamber Conditions:"
  # "Chamber Conditions:"
  # "Station 4-3 Freezer"
  # "Station 4-3 Cab"
  # "Station 4-3 Slide"
  # "Chamber Conditions:"
  # "Chamber Conditions:"
  # "Chamber Conditions:"
  # "Station 4-4 Freezer"
  # "Station 4-4 Cab"
  # "Station 4-4 Slide"
  # "Chamber Conditions:"
  # "Chamber Conditions:"
  # "Chamber Conditions:"
  # "Station 4-5 Freezer"
  # "Station 4-5 Cab"
  # "Station 4-5 Slide"
  # "Chamber Conditions:"
  # "Chamber Conditions:"
  # "Chamber Conditions:"
  # "Station 4-6 Freezer"
  # "Station 4-6 Cab"
  # "Station 4-6 Slide"
  # "Chamber Conditions:"
  # "Chamber Conditions:"
  # "Chamber Conditions:"
  # "Station 4-7 Freezer"
  # "Station 4-7 Cab"
  # "Station 4-7 Slide"
  # "Chamber Conditions:"
  # "Chamber Conditions:"
  # "Chamber Conditions:"
  # "Station 4-8 Freezer"
  # "Station 4-8 Cab"
  # "Station 4-8 Slide"
  # "Chamber Conditions:"
  # "Chamber Conditions:"
  # "Chamber Conditions:"
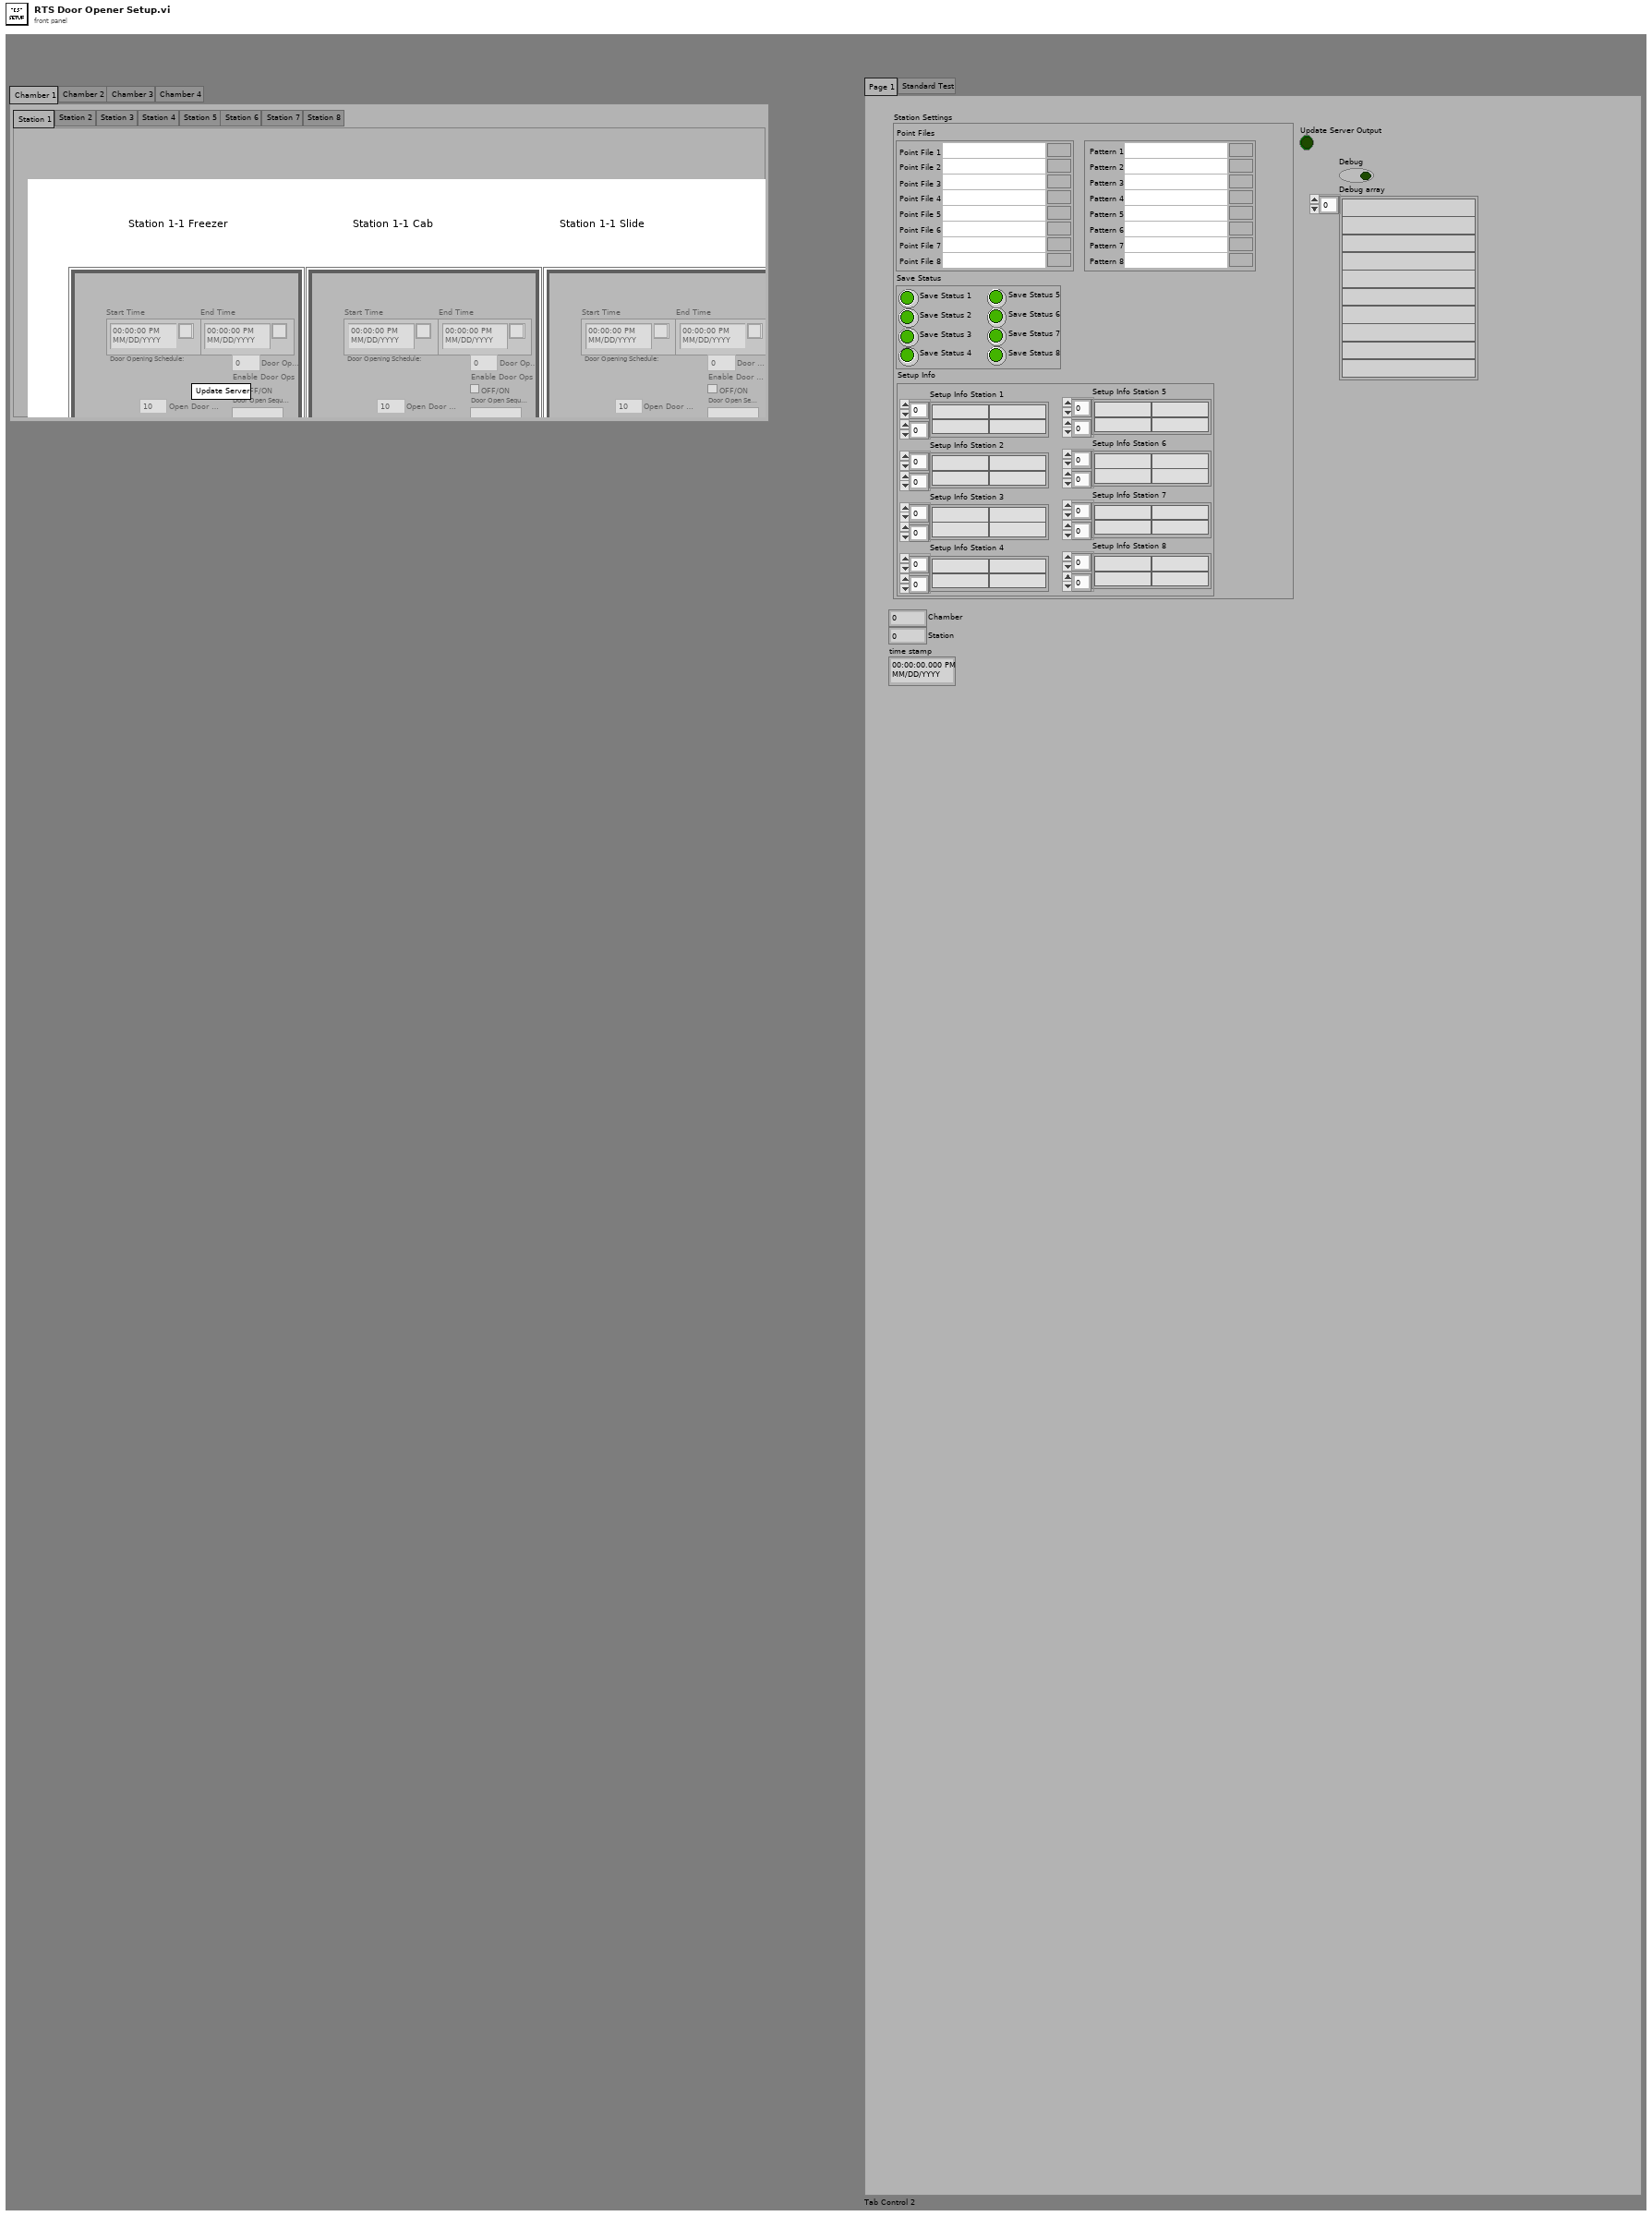
[diagram p1: front panel]
types:
  T1 = typedef "RTS Station Settions TCP Comms.ctl" = cluster{"Point Files":cluster{"Point File 1":path, "Point File 2":path, "Point File 3":path, "Point File 4":path, "Point File 5":path, "Point File 6":path, "Point File 7":path, "Point File 8":path}, "Save Status":T2, "Setup Info":cluster{"Setup Info Station 1":string[][], "Setup Info Station 2":string[][], "Setup Info Station 3":string[][], "Setup Info Station 4":string[][], "Setup Info Station 5":string[][], "Setup Info Station 6":string[][], "Setup Info Station 7":string[][], "Setup Info Station 8":string[][]}, "Chamber Test Pattern":T3}
  T2 = typedef "RTS Chamber Save Status.ctl" = cluster{"Save Status 1":bool, "Save Status 2":bool, "Save Status 3":bool, "Save Status 4":bool, "Save Status 5":bool, "Save Status 6":bool, "Save Status 7":bool, "Save Status 8":bool}
  T3 = typedef "RTS Test Pattern.ctl" = cluster{" Pattern 1":path, "Pattern 2":path, "Pattern 3":path, "Pattern 4":path, "Pattern 5":path, "Pattern 6":path, "Pattern 7":path, "Pattern 8":path}
  T4 = typedef "RTS Door Op Data.ctl" = cluster{"Chamber 1-3":T5[], "Chamber 1-2":T5[], "Chamber 1-1":T5[], "Standard Tests 1-1":T8}
  T5 = typedef "RTS Door Ops Client.ctl" = cluster{"End Time":timestamp, "Start Time":timestamp, "Door Opening Schedule:":T6, "Enable Door Ops":bool, "Door Openings":u32, "Temp (°F)":dbl, "Humidity (%)":dbl, "Voltage (V)":dbl, "Door Open Sequence:":T7, "Door Delay(sec)":dbl, "Dehum (°F)":dbl, "Cool (°F)":dbl}
  T6 = typedef "RTS Door Opening Schedule.ctl" = cluster{"Open Door Timer (s)":dbl, "Delay Time (s)":dbl, "Close Door Timer (s)":dbl}
  T7 = typedef "RTS Door Ops Sequence.ctl" = enum16{"", "1st", "2nd", "3rd"}
  T8 = typedef "RTS Standard Door Opening Test.ctl" = enum16{"Standard ETPs", "511-B113 EHUT", "511-B110 HUT", "512-C410 SLAT", "511-B111 Internal Moisture", "511-C401 Moisture Accumulation", "511-B100 No Door Opening (NDO)", "511-B304 ISO Energy Consumption", "Custom Test", "Cancel Test"}
  T9 = enum32{"Chamber 1", "Chamber 2", "Chamber 3", "Chamber 4"}
  T10 = enum32{"Station 1", "Station 2", "Station 3", "Station 4", "Station 5", "Station 6", "Station 7", "Station 8"}
  T11 = enum32{"invalid app kind", "Development System", "Run Time System", "Student Edition", "Embedded LabVIEW", "Evaluation", "Custom"}
  T12 = enum32{"Invalid", "Standard", "Closed", "Hidden", "Minimized", "Maximized"}
  T13 = cluster{"Core":cluster{"Current VI Reference":refnum<vi>, "Close Panel on Exit?":bool}, "Start Time":string, "End Time":string, "Station Settings":T1, "1-1":T4, "1-2":T4, "1-3":T4, "1-4":T4, "1-5":T4, "1-6":T4, "1-7":T4, "1-8":T4, "2-1":T4, "2-2":T4, "2-3":T4, "2-4":T4, "2-5":T4, "2-6":T4, "2-7":T4, "2-8":T4, "3-1":T4, "3-2":T4, "3-3":T4, "3-4":T4, "3-5":T4, "3-6":T4, "3-7":T4, "3-8":T4, "4-1":T4, "4-2":T4, "4-3":T4, "4-4":T4, "4-5":T4, "4-6":T4, "4-7":T4, "4-8":T4, "Update Server":bool}
  T14 = cluster{"Current VI Reference":refnum<vi>, "Close Panel on Exit?":bool}
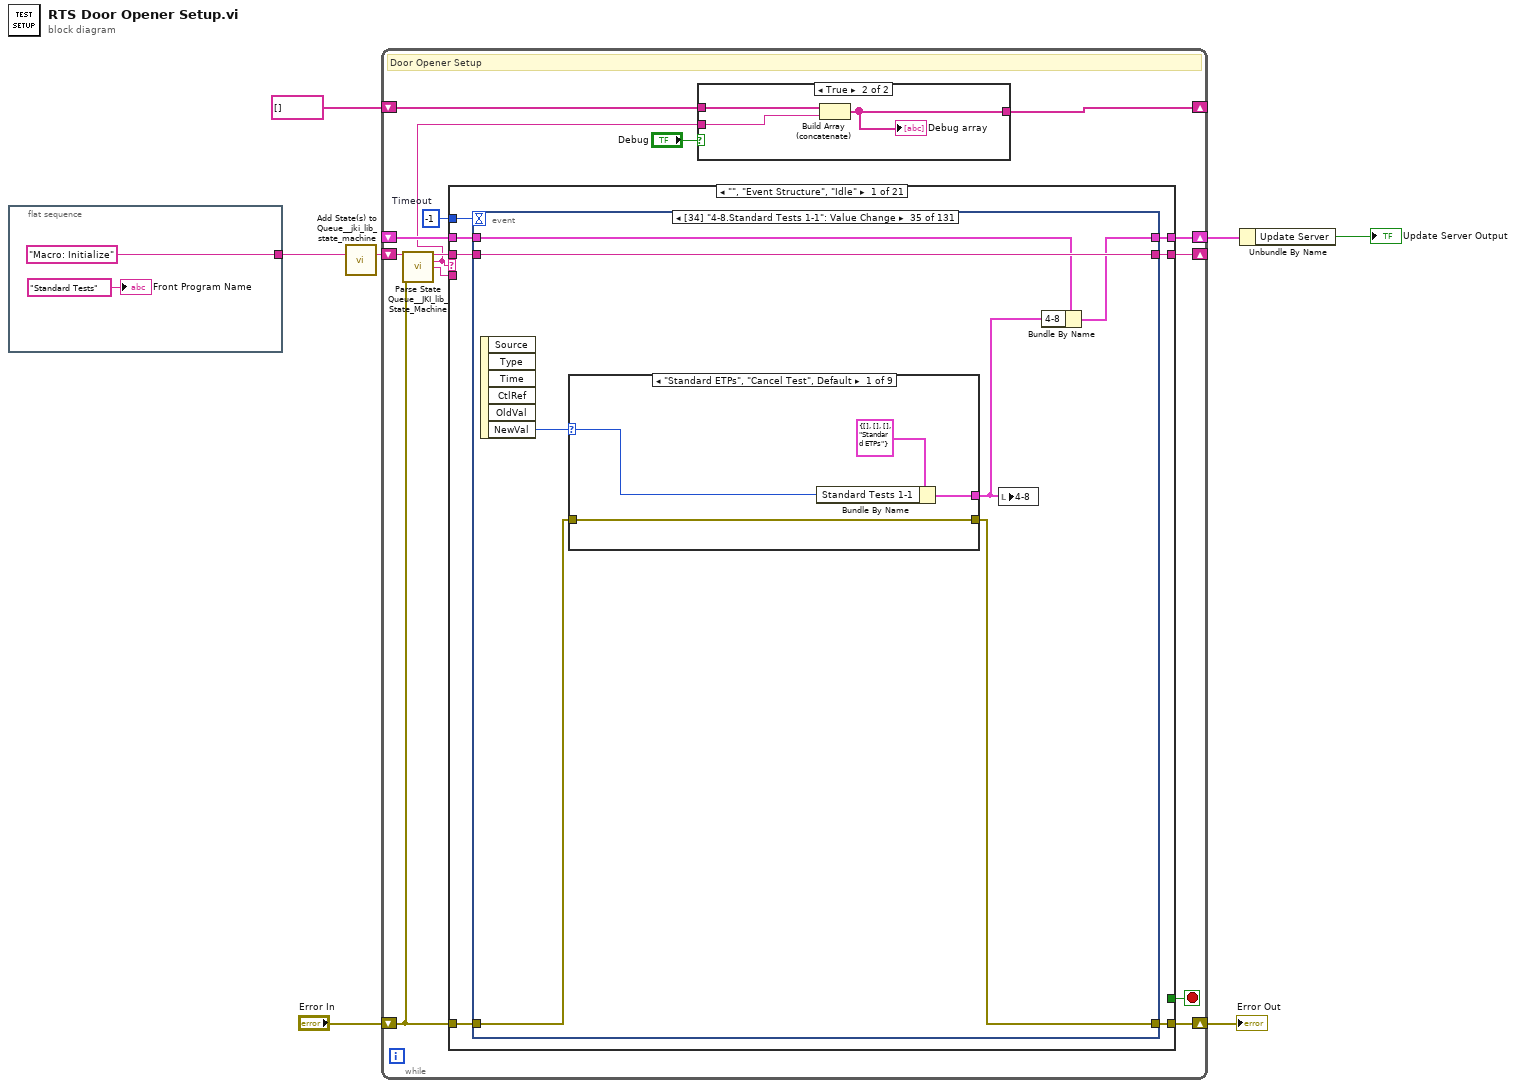
[diagram p0: block diagram]
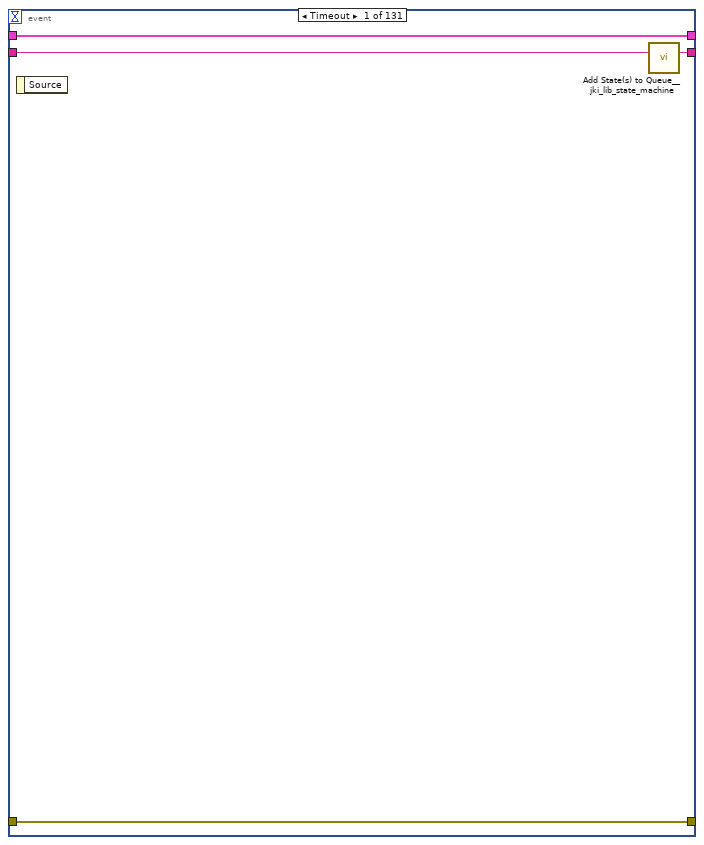
[diagram p3: hidden frame]
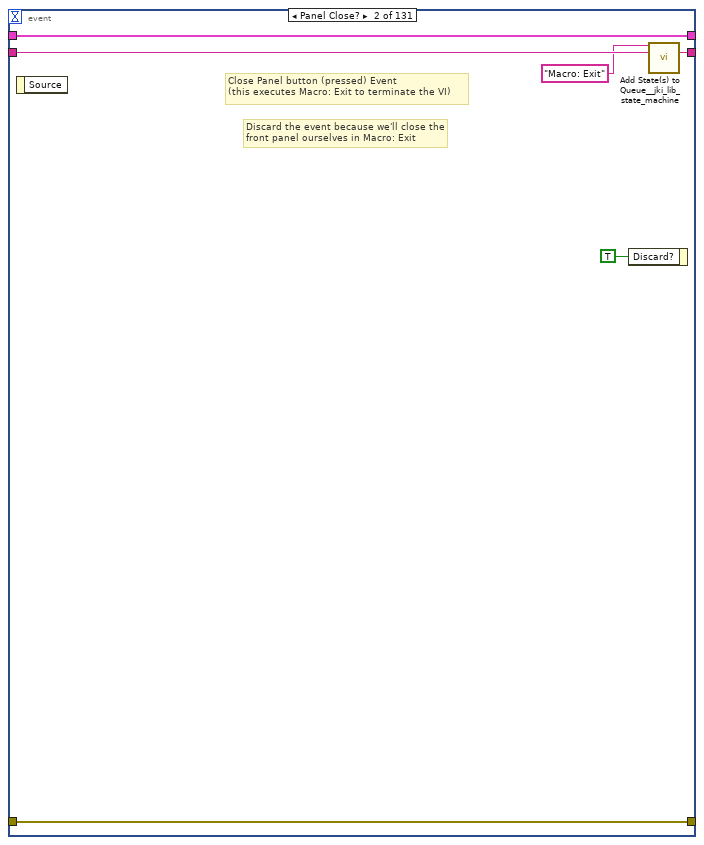
[diagram p4: hidden frame]
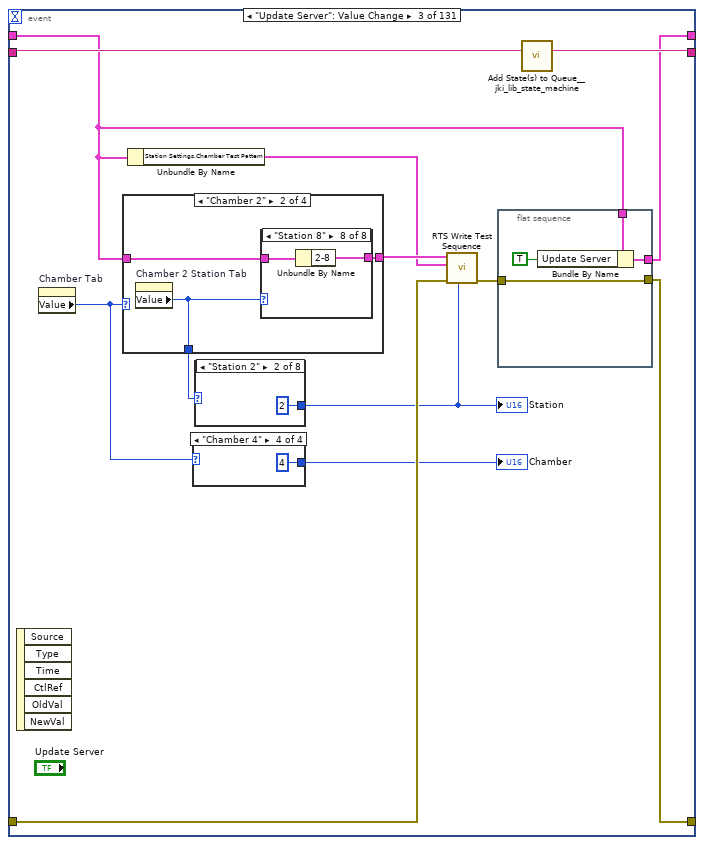
[diagram p5: hidden frame]
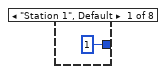
[diagram p6: hidden frame]
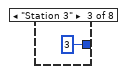
[diagram p7: hidden frame]
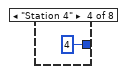
[diagram p8: hidden frame]
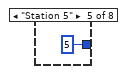
[diagram p9: hidden frame]
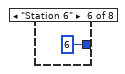
[diagram p10: hidden frame]
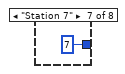
[diagram p11: hidden frame]
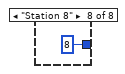
[diagram p12: hidden frame]
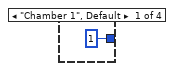
[diagram p13: hidden frame]
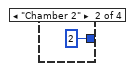
[diagram p14: hidden frame]
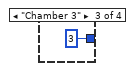
[diagram p15: hidden frame]
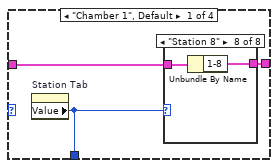
[diagram p16: hidden frame]
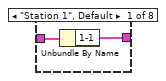
[diagram p17: hidden frame]
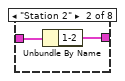
[diagram p18: hidden frame]
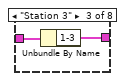
[diagram p19: hidden frame]
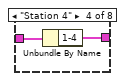
[diagram p20: hidden frame]
diagram:
  n1 = flat-sequence {
    tunnel: ["Macro: Initialize"] -> w4
    frame #0 {
      "Front Program Name" <- "Standard Tests" ("Front Program Name")
    }
  }
  n2 = call <vilib>:"Add State(s) to Queue__jki_lib_state_machine.vi"("State(s) in (\"\")"=w4) -> ("States Out"=w7:string)  [unwired: 14 in]
  n3 = while "JKI - String-Based Queued State Machine (Basic) v1.0" {
    shift-right: [w17] -> w3
    shift-left: _ -> [w16]
    shift-right: [w20] -> w5
    shift-left: "Error In" -> [w14]
    shift-right: [w19] -> _
    shift-left: w7 -> [w21]
    shift-right: [w11] -> _
    shift-left: string[] [] -> [w12]
    stop <- w18 stop-if-true
    w15 = -1  # Timeout
    # "Door Opener Setup"
    n4 = call <vilib>:"Parse State Queue__JKI_lib_State_Machine.vi"("State Queue"=w21, "Error In (no error)"=w14) -> ("Remaining States"=w23:string, "Current State"=w13:string, "Arguments"=w22:string)  [unwired: 11 in]
    n5 = case shown="\"\", \"Event Structure\", \"Idle\"" w13 {
      selector: w13 -> [_ _ w2432 _ _ _ _ _ _ _ _ _ _ _ _ _ _ _ _ _ _]
      tunnel: w23 -> [w34 w2431 w2436 w2454 w2460 w2465 w2469 w2510 w2516 w2520 w2524 w2530 w2538 w2543 w2550 w2576 w2581 w2591 w2595 w2600 w2620]
      tunnel: w22 -> [_ _ _ _ _ _ _ _ _ _ _ w2525 _ _ w2544 _ _ _ _ _ _]
      tunnel: w16 -> [w32 w2428 w2434 w2445 w2457 w2463 w2466 _ w2511 w2517 w2522 w2528 w2536 w2541 w2546 w2573 w2578 w2588 w2592 w2597 w2616]
      tunnel: [w28 w2429 w2438 w2451 errorcluster {"status"=FALSE, "code"=0, "source"=""} ("error out") w2462 w2467 w2507 w2512 w2518 w2521 w2526 w2535 w2540 w2547 w2574 w2579 w2589 w2593 w2598 w2615] -> w20
      tunnel: w14 -> [w31 w2429 w2437 w2451 w2456 w2462 w2467 w2507 w2513 w2518 w2521 w2527 w2535 w2540 w2548 w2574 w2579 w2589 w2593 w2598 w2615]
      tunnel: [w33 w2430 w2435 w2453 w2459 w2464 w2468 w2509 w2515 w2519 w2523 w2529 w2537 w2542 w2549 w2575 w2580 w2590 w2594 w2599 w2619] -> w19
      tunnel: [_ _ _ _ _ TRUE _ _ _ _ _ _ _ _ _ _ _ _ _ _ _] -> w18
      tunnel: [w30 w2428 w2434 w2452 w2457 w2463 w2466 w2508 w2511 w2517 w2522 w2528 w2536 w2541 w2546 w2573 w2578 w2588 w2592 w2596 w2616] -> w17
      tunnel: w15 -> [w29 _ _ _ _ _ _ _ _ _ _ _ _ _ _ _ _ _ _ _ _]
      frame "", "Event Structure", "Idle" {
        n6 = event shown="[34] \"4-8.Standard Tests 1-1\": Value Change" {
          selector: _ -> [_ _ _ _ _ _ _ _ _ _ _ _ _ _ _ _ _ _ _ _ _ _ _ _ _ _ _ _ _ _ _ _ _ _ _ _ _ _ _ _ _ _ _ _ _ _ _ _ _ _ _ _ _ _ _ _ _ _ _ _ _ _ _ _ _ _ _ _ _ _ _ _ _ _ _ _ _ _ _ _ _ _ _ _ _ _ _ _ _ _ _ _ _ _ _ _ _ _ _ _ _ _ _ _ _ _ _ _ _ _ _ _ _ _ _ _ _ _ _ _ _ _ _ _ _ _ _ _ _ _ _]
          dyn-events: _ -> [_ _ _ _ _ _ _ _ _ _ _ _ _ _ _ _ _ _ _ _ _ _ _ _ _ _ _ _ _ _ _ _ _ _ _ _ _ _ _ _ _ _ _ _ _ _ _ _ _ _ _ _ _ _ _ _ _ _ _ _ _ _ _ _ _ _ _ _ _ _ _ _ _ _ _ _ _ _ _ _ _ _ _ _ _ _ _ _ _ _ _ _ _ _ _ _ _ _ _ _ _ _ _ _ _ _ _ _ _ _ _ _ _ _ _ _ _ _ _ _ _ _ _ _ _ _ _ _ _ _ _]
          timeout: w29 -> [_ _ _ _ _ _ _ _ _ _ _ _ _ _ _ _ _ _ _ _ _ _ _ _ _ _ _ _ _ _ _ _ _ _ _ _ _ _ _ _ _ _ _ _ _ _ _ _ _ _ _ _ _ _ _ _ _ _ _ _ _ _ _ _ _ _ _ _ _ _ _ _ _ _ _ _ _ _ _ _ _ _ _ _ _ _ _ _ _ _ _ _ _ _ _ _ _ _ _ _ _ _ _ _ _ _ _ _ _ _ _ _ _ _ _ _ _ _ _ _ _ _ _ _ _ _ _ _ _ _ _]
          tunnel: w34 -> [w38 w44 w56 w156 w196 w236 w276 w317 w358 w399 w442 w483 w524 w563 w606 w645 w686 w729 w768 w811 w852 w893 w934 w975 w1016 w1057 w1098 w1137 w1180 w1219 w1262 w1303 w1345 w1385 w1426 w1473 w1479 w1491 w1507 w1511 w1527 w1531 w1541 w1551 w1561 w1571 w1581 w1591 w1601 w1611 w1621 w1631 w1641 w1651 w1667 w1671 w1681 w1691 w1701 w1711 w1723 w1735 w1741 w1753 w1763 w1775 w1781 w1792 w1801 w1814 w1821 w1833 w1841 w1851 w1863 w1877 w1881 w1893 w1901 w1917 w1923 w1937 w1944 w1952 w1962 w1972 w1981 w1997 w2003 w2012 w2027 w2035 w2044 w2055 w2061 w2074 w2081 w2094 w2103 w2117 w2121 w2132 w2142 w2153 w2161 w2175 w2187 w2197 w2201 w2213 w2224 w2231 w2244 w2257 w2264 w2277 w2282 w2294 w2307 w2312 w2324 w2334 w2347 w2354 w2361 w2371 w2385 w2395 w2404 w2415 w2425]
          tunnel: [w37 w43 w57 w156 w196 w236 w276 w317 w358 w399 w442 w483 w524 w563 w606 w645 w686 w729 w768 w811 w852 w893 w934 w975 w1016 w1057 w1098 w1137 w1180 w1219 w1262 w1303 w1345 w1385 w1426 w1473 w1479 w1491 w1507 w1511 w1527 w1531 w1541 w1551 w1561 w1571 w1581 w1591 w1601 w1611 w1621 w1631 w1641 w1651 w1667 w1671 w1681 w1691 w1701 w1711 w1723 w1735 w1741 w1753 w1763 w1775 w1781 w1792 w1801 w1814 w1821 w1833 w1841 w1851 w1863 w1877 w1881 w1893 w1901 w1917 w1923 w1937 w1944 w1952 w1962 w1972 w1981 w1997 w2003 w2012 w2027 w2035 w2044 w2055 w2061 w2074 w2081 w2094 w2103 w2117 w2121 w2132 w2142 w2153 w2161 w2175 w2187 w2197 w2201 w2213 w2224 w2231 w2244 w2257 w2264 w2277 w2282 w2294 w2307 w2312 w2324 w2334 w2347 w2354 w2361 w2371 w2385 w2395 w2404 w2415 w2425] -> w33
          tunnel: w32 -> [w35 w41 w46 w152 w193 w234 w275 w316 w357 w398 w439 w480 w521 w562 w603 w644 w685 w726 w767 w808 w849 w890 w931 w972 w1013 w1054 w1095 w1136 w1177 w1218 w1259 w1300 w1341 w1382 w1423 w1464 w1476 w1488 w1500 w1510 w1520 w1530 w1540 w1550 w1560 w1570 w1580 w1590 w1600 w1610 w1620 w1630 w1640 w1650 w1660 w1670 w1680 w1690 w1700 w1710 w1720 w1730 w1740 w1750 w1760 w1770 w1780 w1790 w1800 w1810 w1820 w1830 w1840 w1850 w1860 w1870 w1880 w1890 w1900 w1910 w1920 w1930 w1940 w1950 w1960 w1970 w1980 w1990 w2000 w2010 w2020 w2030 w2040 w2050 w2060 w2070 w2080 w2090 w2100 w2110 w2120 w2130 w2140 w2150 w2160 w2170 w2180 w2190 w2200 w2210 w2220 w2230 w2240 w2250 w2260 w2270 w2280 w2290 w2300 w2310 w2320 w2330 w2340 w2350 w2360 w2370 w2380 w2390 w2400 w2410 w2420]
          tunnel: [w36 w42 w47 w153 w194 w237 w278 w318 w359 w400 w440 w481 w522 w564 w604 w646 w687 w727 w769 w809 w850 w891 w932 w973 w1014 w1055 w1096 w1138 w1178 w1220 w1260 w1301 w1342 w1383 w1424 w1468 w1480 w1494 w1501 w1512 w1521 w1532 w1542 w1552 w1562 w1572 w1582 w1592 w1602 w1614 w1622 w1633 w1642 w1653 w1661 w1672 w1682 w1693 w1703 w1712 w1721 w1731 w1742 w1751 w1761 w1773 w1784 w1793 w1804 w1812 w1824 w1834 w1844 w1854 w1861 w1873 w1883 w1895 w1904 w1913 w1921 w1933 w1942 w1954 w1964 w1974 w1984 w1993 w2005 w2014 w2023 w2033 w2042 w2053 w2064 w2072 w2084 w2092 w2104 w2113 w2123 w2133 w2144 w2154 w2163 w2173 w2182 w2192 w2204 w2214 w2222 w2234 w2242 w2251 w2262 w2273 w2284 w2292 w2302 w2314 w2322 w2332 w2343 w2352 w2364 w2373 w2382 w2392 w2402 w2412 w2423] -> w28
          tunnel: w31 -> [w36 w42 w55 w154 w195 w238 w279 w319 w360 w401 w441 w482 w523 w565 w605 w647 w688 w728 w770 w810 w851 w892 w933 w974 w1015 w1056 w1097 w1139 w1179 w1221 w1261 w1302 w1343 w1384 w1425 w1469 w1481 w1493 w1502 w1513 w1522 w1533 w1543 w1553 w1563 w1573 w1583 w1593 w1603 w1615 w1623 w1634 w1643 w1654 w1662 w1673 w1683 w1694 w1704 w1713 w1722 w1732 w1743 w1752 w1762 w1774 w1785 w1794 w1805 w1813 w1825 w1835 w1845 w1855 w1862 w1874 w1884 w1894 w1905 w1914 w1922 w1934 w1943 w1955 w1965 w1975 w1985 w1994 w2004 w2015 w2024 w2034 w2043 w2054 w2065 w2073 w2085 w2093 w2105 w2114 w2124 w2134 w2145 w2155 w2164 w2174 w2183 w2193 w2205 w2215 w2223 w2235 w2243 w2252 w2263 w2274 w2285 w2293 w2303 w2315 w2323 w2333 w2344 w2353 w2365 w2374 w2383 w2393 w2403 w2413 w2424]
          tunnel: [w35 w41 w45 w151 w192 w233 w274 w315 w356 w397 w438 w479 w520 w561 w602 w643 w684 w725 w766 w807 w848 w889 w930 w971 w1012 w1053 w1094 w1135 w1176 w1217 w1258 w1299 w1340 w1381 w1422 w1463 w1475 w1487 w1499 w1509 w1519 w1529 w1539 w1549 w1559 w1569 w1579 w1589 w1599 w1609 w1619 w1629 w1639 w1649 w1659 w1669 w1679 w1689 w1699 w1709 w1719 w1729 w1739 w1749 w1759 w1769 w1779 w1789 w1799 w1809 w1819 w1829 w1839 w1849 w1859 w1869 w1879 w1889 w1899 w1909 w1919 w1929 w1939 w1949 w1959 w1969 w1979 w1989 w1999 w2009 w2019 w2029 w2039 w2049 w2059 w2069 w2079 w2089 w2099 w2109 w2119 w2129 w2139 w2149 w2159 w2169 w2179 w2189 w2199 w2209 w2219 w2229 w2239 w2249 w2259 w2269 w2279 w2289 w2299 w2309 w2319 w2329 w2339 w2349 w2359 w2369 w2379 w2389 w2399 w2409 w2419] -> w30
          event Timeout {
            n7 = event-data() -> ()  [unwired: 1 in, 1 out]
            n8 = call <vilib>:"Add State(s) to Queue__jki_lib_state_machine.vi"("State(s) in (\"\")"=w38) -> ("States Out"=w37:string)  [unwired: 14 in]
          }
          event Panel Close? {
            # "Discard the event because we'll close the front panel ourselves in Macro: Exit"
            # "Close Panel button (pressed) Event\n(this executes Macro: Exit to terminate the VI)"
            n9 = event-data() -> ()  [unwired: 1 in, 1 out]
            n10 = event-data("Discard?"=TRUE) -> ()  [unwired: 1 in, 1 out]
            n11 = call <vilib>:"Add State(s) to Queue__jki_lib_state_machine.vi"("State(s) in Front (\"\")"="Macro: Exit", "State(s) in (\"\")"=w44) -> ("States Out"=w43:string)  [unwired: 13 in]
          }
          event "Update Server": Value Change {
            n12 = event-data() -> ()  [unwired: 1 in, 6 out]
            n13 = property on="Chamber Tab" class="TabCtl (strict)"() -> ("Value"=w53:T9)  [unwired: 2 in, 2 out]
            n14 = case shown="\"Chamber 2\"" w53 {
              tunnel: w46 -> [w76 w95 w114 w133]
              tunnel: [w75 w94 w113 w132] -> w54
              tunnel: [w74 w93 w112 w131] -> w51
              frame "Chamber 1", Default {
                n15 = property on="Station Tab" class="TabCtl (strict)"() -> ("Value"=w74:T10)  [unwired: 2 in, 2 out]
                n16 = case shown="\"Station 8\"" w74 {
                  tunnel: w76 -> [w78 w80 w82 w84 w86 w88 w90 w92]
                  tunnel: [w77 w79 w81 w83 w85 w87 w89 w91] -> w75
                  frame "Station 1", Default {
                    n17 = Unbundle By Name(w78) -> ("1-1"=w77:T4)
                  }
                  frame "Station 2" {
                    n18 = Unbundle By Name(w80) -> ("1-2"=w79:T4)
                  }
                  frame "Station 3" {
                    n19 = Unbundle By Name(w82) -> ("1-3"=w81:T4)
                  }
                  frame "Station 4" {
                    n20 = Unbundle By Name(w84) -> ("1-4"=w83:T4)
                  }
                  frame "Station 5" {
                    n21 = Unbundle By Name(w86) -> ("1-5"=w85:T4)
                  }
                  frame "Station 6" {
                    n22 = Unbundle By Name(w88) -> ("1-6"=w87:T4)
                  }
                  frame "Station 7" {
                    n23 = Unbundle By Name(w90) -> ("1-7"=w89:T4)
                  }
                  frame "Station 8" {
                    n24 = Unbundle By Name(w92) -> ("1-8"=w91:T4)
                  }
                }
              }
              frame "Chamber 2" {
                n25 = property on="Chamber 2 Station Tab" class="TabCtl (strict)"() -> ("Value"=w93:T10)  [unwired: 2 in, 2 out]
                n26 = case shown="\"Station 8\"" w93 {
                  tunnel: w95 -> [w97 w99 w101 w103 w105 w107 w109 w111]
                  tunnel: [w96 w98 w100 w102 w104 w106 w108 w110] -> w94
                  frame "Station 1", Default {
                    n27 = Unbundle By Name(w97) -> ("2-1"=w96:T4)
                  }
                  frame "Station 2" {
                    n28 = Unbundle By Name(w99) -> ("2-2"=w98:T4)
                  }
                  frame "Station 3" {
                    n29 = Unbundle By Name(w101) -> ("2-3"=w100:T4)
                  }
                  frame "Station 4" {
                    n30 = Unbundle By Name(w103) -> ("2-4"=w102:T4)
                  }
                  frame "Station 5" {
                    n31 = Unbundle By Name(w105) -> ("2-5"=w104:T4)
                  }
                  frame "Station 6" {
                    n32 = Unbundle By Name(w107) -> ("2-6"=w106:T4)
                  }
                  frame "Station 7" {
                    n33 = Unbundle By Name(w109) -> ("2-7"=w108:T4)
                  }
                  frame "Station 8" {
                    n34 = Unbundle By Name(w111) -> ("2-8"=w110:T4)
                  }
                }
              }
              frame "Chamber 3" {
                n35 = property on="Chamber 3 Station Tab" class="TabCtl (strict)"() -> ("Value"=w112:T10)  [unwired: 2 in, 2 out]
                n36 = case shown="\"Station 8\"" w112 {
                  tunnel: w114 -> [w116 w118 w120 w122 w124 w126 w128 w130]
                  tunnel: [w115 w117 w119 w121 w123 w125 w127 w129] -> w113
                  frame "Station 1", Default {
                    n37 = Unbundle By Name(w116) -> ("3-1"=w115:T4)
                  }
                  frame "Station 2" {
                    n38 = Unbundle By Name(w118) -> ("3-2"=w117:T4)
                  }
                  frame "Station 3" {
                    n39 = Unbundle By Name(w120) -> ("3-3"=w119:T4)
                  }
                  frame "Station 4" {
                    n40 = Unbundle By Name(w122) -> ("3-4"=w121:T4)
                  }
                  frame "Station 5" {
                    n41 = Unbundle By Name(w124) -> ("3-5"=w123:T4)
                  }
                  frame "Station 6" {
                    n42 = Unbundle By Name(w126) -> ("3-6"=w125:T4)
                  }
                  frame "Station 7" {
                    n43 = Unbundle By Name(w128) -> ("3-7"=w127:T4)
                  }
                  frame "Station 8" {
                    n44 = Unbundle By Name(w130) -> ("3-8"=w129:T4)
                  }
                }
              }
              frame "Chamber 4" {
                n45 = property on="Chamber 4 Station Tab" class="TabCtl (strict)"() -> ("Value"=w131:T10)  [unwired: 2 in, 2 out]
                n46 = case shown="\"Station 2\"" w131 {
                  tunnel: w133 -> [w135 w137 w139 w141 w143 w145 w147 w149]
                  tunnel: [w134 w136 w138 w140 w142 w144 w146 w148] -> w132
                  frame "Station 1", Default {
                    n47 = Unbundle By Name(w135) -> ("4-1"=w134:T4)
                  }
                  frame "Station 2" {
                    n48 = Unbundle By Name(w137) -> ("4-2"=w136:T4)
                  }
                  frame "Station 3" {
                    n49 = Unbundle By Name(w139) -> ("4-3"=w138:T4)
                  }
                  frame "Station 4" {
                    n50 = Unbundle By Name(w141) -> ("4-4"=w140:T4)
                  }
                  frame "Station 5" {
                    n51 = Unbundle By Name(w143) -> ("4-5"=w142:T4)
                  }
                  frame "Station 6" {
                    n52 = Unbundle By Name(w145) -> ("4-6"=w144:T4)
                  }
                  frame "Station 7" {
                    n53 = Unbundle By Name(w147) -> ("4-7"=w146:T4)
                  }
                  frame "Station 8" {
                    n54 = Unbundle By Name(w149) -> ("4-8"=w148:T4)
                  }
                }
              }
            }
            n55 = Unbundle By Name(w46) -> ("Station Settings.Chamber Test Pattern"=w49:T3)
            n56 = case shown="\"Chamber 4\"" w53 {
              tunnel: [u16 1 u16 2 u16 3 u16 4] -> w52
              frame "Chamber 1", Default {
              }
              frame "Chamber 2" {
              }
              frame "Chamber 3" {
              }
              frame "Chamber 4" {
              }
            }
            "Chamber" <- w52
            n57 = case shown="\"Station 2\"" w51 {
              tunnel: [u16 1 u16 2 u16 3 u16 4 u16 5 u16 6 u16 7 u16 8] -> w50
              frame "Station 1", Default {
              }
              frame "Station 2" {
              }
              frame "Station 3" {
              }
              frame "Station 4" {
              }
              frame "Station 5" {
              }
              frame "Station 6" {
              }
              frame "Station 7" {
              }
              frame "Station 8" {
              }
            }
            "Station" <- w50
            n58 = call "RTS Write Test Sequence.vi"("Station Number"=w50, "Error In"=w55, "Station Settings.Chamber Test Pattern"=w49, "Current Config File"=w54) -> ("Error Out"=w48:errorcluster)  [unwired: 7 in]
            n59 = flat-sequence {
              tunnel: w46 -> [w61]
              tunnel: w48 -> [w59]
              tunnel: [w59] -> w47
              tunnel: [w58] -> w45
              frame #0 {
                n60 = Bundle By Name(cluster=w61, "Update Server"=TRUE) -> (w58:T13)
              }
            }
            n61 = call <vilib>:"Add State(s) to Queue__jki_lib_state_machine.vi"("State(s) in (\"\")"=w56) -> ("States Out"=w57:string)  [unwired: 14 in]
          }
          event Value Change {
            n62 = event-data() -> ("NewVal"=w155:T8)  [unwired: 1 in, 5 out]
            n63 = case shown="\"Standard ETPs\", \"Cancel Test\", Default" w155 {
              selector: w155 -> [w158 _ _ _ _ _ _ _ _]
              tunnel: [w157 w164 w167 w171 w175 w180 w183 w187 w190] -> w150
              tunnel: w154 -> [w160 w163 w166 w170 w174 w179 w181 w186 w189]
              tunnel: [w160 w162 w165 w169 w173 w178 w184 w188 w189] -> w153
              frame "Standard ETPs", "Cancel Test", Default {
                n64 = Bundle By Name(cluster=T4 {"Chamber 1-3"=[], "Chamber 1-2"=[], "Chamber 1-1"=[], "Standard Tests 1-1"=enum."Standard ETPs"} ("1-1"), "Standard Tests 1-1"=w158) -> (w157:T4)
              }
              frame "511-B113 EHUT" {
                # "This is basically a 14 HUT"
                n65 = call "RTS Standard Test Set Time.vi"("Error In"=w163, "Internal Moisture Test (511-B111) - 5 Days"="EHUT (511-B113)") -> ("Error Out"=w162:errorcluster, "Output"=w164:T4)  [unwired: 8 in]
              }
              frame "511-B110 HUT" {
                # "24 Hr HUT"
                n66 = call "RTS Standard Test Set Time.vi"("Error In"=w166, "Internal Moisture Test (511-B111) - 5 Days"="HUT (511-B110)") -> ("Error Out"=w165:errorcluster, "Output"=w167:T4)  [unwired: 8 in]
              }
              frame "512-C410 SLAT" {
                n67 = call "RTS Standard Test Set Time.vi"("Error In"=w170, "Internal Moisture Test (511-B111) - 5 Days"="SLAT (512-C419)") -> ("Error Out"=w169:errorcluster, "Output"=w171:T4)  [unwired: 8 in]
              }
              frame "511-B111 Internal Moisture" {
                # "This is a 5 day HUT"
                n68 = call "RTS Standard Test Set Time.vi"("Error In"=w174, "Internal Moisture Test (511-B111) - 5 Days"="Internal Moisture Test (511-B111) - 5 Days") -> ("Error Out"=w173:errorcluster, "Output"=w175:T4)  [unwired: 8 in]
              }
              frame "511-C401 Moisture Accumulation" {
                n69 = call "RTS Standard Test Set Time.vi"("Error In"=w179, "Internal Moisture Test (511-B111) - 5 Days"="Moisture Accumulation (511-C401)") -> ("Error Out"=w178:errorcluster, "Output"=w180:T4)  [unwired: 8 in]
              }
              frame "511-B100 No Door Opening (NDO)" {
                n70 = call "RTS Standard Test Set Time.vi"("Error In"=w181, "Internal Moisture Test (511-B111) - 5 Days"="NDO") -> ("Error Out"=w184:errorcluster, "Output"=w183:T4)  [unwired: 8 in]
              }
              frame "511-B304 ISO Energy Consumption" {
                n71 = call "RTS Standard Test Set Time.vi"("Error In"=w186, "Internal Moisture Test (511-B111) - 5 Days"="ISO Energy Consumption") -> ("Error Out"=w188:errorcluster, "Output"=w187:T4)  [unwired: 8 in]
              }
              frame "Custom Test" {
                n72 = local read "1-1"() -> (w190:T4)
              }
            }
            n73 = local write "1-1"(w150) -> ()
            n74 = Bundle By Name(cluster=w152, "1-1"=w150) -> (w151:T13)
          }
          event Value Change {
            n75 = event-data() -> ("NewVal"=w197:T8)  [unwired: 1 in, 5 out]
            n76 = case shown="\"Standard ETPs\", \"Cancel Test\", Default" w197 {
              selector: w197 -> [w198 _ _ _ _ _ _ _ _]
              tunnel: [w199 w205 w209 w213 w217 w221 w224 w228 w231] -> w191
              tunnel: w195 -> [w201 w204 w208 w212 w216 w220 w223 w227 w230]
              tunnel: [w201 w203 w207 w211 w215 w219 w225 w229 w230] -> w194
              frame "Standard ETPs", "Cancel Test", Default {
                n77 = Bundle By Name(cluster=T4 {"Chamber 1-3"=[], "Chamber 1-2"=[], "Chamber 1-1"=[], "Standard Tests 1-1"=enum."Standard ETPs"} ("1-1"), "Standard Tests 1-1"=w198) -> (w199:T4)
              }
              frame "511-B113 EHUT" {
                # "This is basically a 14 HUT"
                n78 = local read "EHUT (511-B113)"() -> (w202:T4)
                n79 = call "RTS Standard Test Set Time.vi"("Error In"=w204, "Internal Moisture Test (511-B111) - 5 Days"=w202) -> ("Error Out"=w203:errorcluster, "Output"=w205:T4)  [unwired: 8 in]
              }
              frame "511-B110 HUT" {
                # "24 Hr HUT"
                n80 = local read "HUT (511-B110)"() -> (w206:T4)
                n81 = call "RTS Standard Test Set Time.vi"("Error In"=w208, "Internal Moisture Test (511-B111) - 5 Days"=w206) -> ("Error Out"=w207:errorcluster, "Output"=w209:T4)  [unwired: 8 in]
              }
              frame "512-C410 SLAT" {
                n82 = local read "SLAT (512-C419)"() -> (w210:T4)
                n83 = call "RTS Standard Test Set Time.vi"("Error In"=w212, "Internal Moisture Test (511-B111) - 5 Days"=w210) -> ("Error Out"=w211:errorcluster, "Output"=w213:T4)  [unwired: 8 in]
              }
              frame "511-B111 Internal Moisture" {
                # "This is a 5 day HUT"
                n84 = local read "Internal Moisture Test (511-B111) - 5 Days"() -> (w214:T4)
                n85 = call "RTS Standard Test Set Time.vi"("Error In"=w216, "Internal Moisture Test (511-B111) - 5 Days"=w214) -> ("Error Out"=w215:errorcluster, "Output"=w217:T4)  [unwired: 8 in]
              }
              frame "511-C401 Moisture Accumulation" {
                n86 = local read "Moisture Accumulation (511-C401)"() -> (w218:T4)
                n87 = call "RTS Standard Test Set Time.vi"("Error In"=w220, "Internal Moisture Test (511-B111) - 5 Days"=w218) -> ("Error Out"=w219:errorcluster, "Output"=w221:T4)  [unwired: 8 in]
              }
              frame "511-B100 No Door Opening (NDO)" {
                n88 = local read "NDO"() -> (w222:T4)
                n89 = call "RTS Standard Test Set Time.vi"("Error In"=w223, "Internal Moisture Test (511-B111) - 5 Days"=w222) -> ("Error Out"=w225:errorcluster, "Output"=w224:T4)  [unwired: 8 in]
              }
              frame "511-B304 ISO Energy Consumption" {
                n90 = local read "ISO Energy Consumption"() -> (w226:T4)
                n91 = call "RTS Standard Test Set Time.vi"("Error In"=w227, "Internal Moisture Test (511-B111) - 5 Days"=w226) -> ("Error Out"=w229:errorcluster, "Output"=w228:T4)  [unwired: 8 in]
              }
              frame "Custom Test" {
                n92 = local read "1-2"() -> (w231:T4)
              }
            }
            n93 = local write "1-2"(w191) -> ()
            n94 = Bundle By Name(cluster=w193, "1-2"=w191) -> (w192:T13)
          }
          event Value Change {
            n95 = event-data() -> ("NewVal"=w235:T8)  [unwired: 1 in, 5 out]
            n96 = case shown="\"Standard ETPs\", \"Cancel Test\", Default" w235 {
              selector: w235 -> [w239 _ _ _ _ _ _ _ _]
              tunnel: [w240 w246 w250 w254 w258 w262 w265 w268 w271] -> w232
              tunnel: w238 -> [w242 w245 w249 w253 w257 w261 w264 w267 w270]
              tunnel: [w242 w244 w248 w252 w256 w260 w266 w267 w272] -> w237
              frame "Standard ETPs", "Cancel Test", Default {
                n97 = Bundle By Name(cluster=T4 {"Chamber 1-3"=[], "Chamber 1-2"=[], "Chamber 1-1"=[], "Standard Tests 1-1"=enum."Standard ETPs"} ("1-1"), "Standard Tests 1-1"=w239) -> (w240:T4)
              }
              frame "511-B113 EHUT" {
                # "This is basically a 14 HUT"
                n98 = local read "EHUT (511-B113)"() -> (w243:T4)
                n99 = call "RTS Standard Test Set Time.vi"("Error In"=w245, "Internal Moisture Test (511-B111) - 5 Days"=w243) -> ("Error Out"=w244:errorcluster, "Output"=w246:T4)  [unwired: 8 in]
              }
              frame "511-B110 HUT" {
                # "24 Hr HUT"
                n100 = local read "HUT (511-B110)"() -> (w247:T4)
                n101 = call "RTS Standard Test Set Time.vi"("Error In"=w249, "Internal Moisture Test (511-B111) - 5 Days"=w247) -> ("Error Out"=w248:errorcluster, "Output"=w250:T4)  [unwired: 8 in]
              }
              frame "512-C410 SLAT" {
                n102 = local read "SLAT (512-C419)"() -> (w251:T4)
                n103 = call "RTS Standard Test Set Time.vi"("Error In"=w253, "Internal Moisture Test (511-B111) - 5 Days"=w251) -> ("Error Out"=w252:errorcluster, "Output"=w254:T4)  [unwired: 8 in]
              }
              frame "511-B111 Internal Moisture" {
                # "This is a 5 day HUT"
                n104 = local read "Internal Moisture Test (511-B111) - 5 Days"() -> (w255:T4)
                n105 = call "RTS Standard Test Set Time.vi"("Error In"=w257, "Internal Moisture Test (511-B111) - 5 Days"=w255) -> ("Error Out"=w256:errorcluster, "Output"=w258:T4)  [unwired: 8 in]
              }
              frame "511-C401 Moisture Accumulation" {
                n106 = local read "Moisture Accumulation (511-C401)"() -> (w259:T4)
                n107 = call "RTS Standard Test Set Time.vi"("Error In"=w261, "Internal Moisture Test (511-B111) - 5 Days"=w259) -> ("Error Out"=w260:errorcluster, "Output"=w262:T4)  [unwired: 8 in]
              }
              frame "511-B100 No Door Opening (NDO)" {
                n108 = local read "NDO"() -> (w263:T4)
                n109 = call "RTS Standard Test Set Time.vi"("Error In"=w264, "Internal Moisture Test (511-B111) - 5 Days"=w263) -> ("Error Out"=w266:errorcluster, "Output"=w265:T4)  [unwired: 8 in]
              }
              frame "Custom Test" {
                n110 = local read "1-3"() -> (w268:T4)
              }
              frame "511-B304 ISO Energy Consumption" {
                n111 = local read "ISO Energy Consumption"() -> (w269:T4)
                n112 = call "RTS Standard Test Set Time.vi"("Error In"=w270, "Internal Moisture Test (511-B111) - 5 Days"=w269) -> ("Error Out"=w272:errorcluster, "Output"=w271:T4)  [unwired: 8 in]
              }
            }
            n113 = local write "1-3"(w232) -> ()
            n114 = Bundle By Name(cluster=w234, "1-3"=w232) -> (w233:T13)
          }
          event Value Change {
            n115 = event-data() -> ("NewVal"=w277:T8)  [unwired: 1 in, 5 out]
            n116 = case shown="\"Standard ETPs\", \"Cancel Test\", Default" w277 {
              selector: w277 -> [w280 _ _ _ _ _ _ _ _]
              tunnel: [w282 w287 w291 w295 w299 w303 w306 w309 w312] -> w273
              tunnel: w279 -> [w283 w286 w290 w294 w298 w302 w305 w308 w311]
              tunnel: [w283 w285 w289 w293 w297 w301 w307 w308 w313] -> w278
              frame "Standard ETPs", "Cancel Test", Default {
                n117 = Bundle By Name(cluster=T4 {"Chamber 1-3"=[], "Chamber 1-2"=[], "Chamber 1-1"=[], "Standard Tests 1-1"=enum."Standard ETPs"} ("1-1"), "Standard Tests 1-1"=w280) -> (w282:T4)
              }
              frame "511-B113 EHUT" {
                # "This is basically a 14 HUT"
                n118 = local read "EHUT (511-B113)"() -> (w284:T4)
                n119 = call "RTS Standard Test Set Time.vi"("Error In"=w286, "Internal Moisture Test (511-B111) - 5 Days"=w284) -> ("Error Out"=w285:errorcluster, "Output"=w287:T4)  [unwired: 8 in]
              }
              frame "511-B110 HUT" {
                # "24 Hr HUT"
                n120 = local read "HUT (511-B110)"() -> (w288:T4)
                n121 = call "RTS Standard Test Set Time.vi"("Error In"=w290, "Internal Moisture Test (511-B111) - 5 Days"=w288) -> ("Error Out"=w289:errorcluster, "Output"=w291:T4)  [unwired: 8 in]
              }
              frame "512-C410 SLAT" {
                n122 = local read "SLAT (512-C419)"() -> (w292:T4)
                n123 = call "RTS Standard Test Set Time.vi"("Error In"=w294, "Internal Moisture Test (511-B111) - 5 Days"=w292) -> ("Error Out"=w293:errorcluster, "Output"=w295:T4)  [unwired: 8 in]
              }
              frame "511-B111 Internal Moisture" {
                # "This is a 5 day HUT"
                n124 = local read "Internal Moisture Test (511-B111) - 5 Days"() -> (w296:T4)
                n125 = call "RTS Standard Test Set Time.vi"("Error In"=w298, "Internal Moisture Test (511-B111) - 5 Days"=w296) -> ("Error Out"=w297:errorcluster, "Output"=w299:T4)  [unwired: 8 in]
              }
              frame "511-C401 Moisture Accumulation" {
                n126 = local read "Moisture Accumulation (511-C401)"() -> (w300:T4)
                n127 = call "RTS Standard Test Set Time.vi"("Error In"=w302, "Internal Moisture Test (511-B111) - 5 Days"=w300) -> ("Error Out"=w301:errorcluster, "Output"=w303:T4)  [unwired: 8 in]
              }
              frame "511-B100 No Door Opening (NDO)" {
                n128 = local read "NDO"() -> (w304:T4)
                n129 = call "RTS Standard Test Set Time.vi"("Error In"=w305, "Internal Moisture Test (511-B111) - 5 Days"=w304) -> ("Error Out"=w307:errorcluster, "Output"=w306:T4)  [unwired: 8 in]
              }
              frame "Custom Test" {
                n130 = local read "1-4"() -> (w309:T4)
              }
              frame "511-B304 ISO Energy Consumption" {
                n131 = local read "ISO Energy Consumption"() -> (w310:T4)
                n132 = call "RTS Standard Test Set Time.vi"("Error In"=w311, "Internal Moisture Test (511-B111) - 5 Days"=w310) -> ("Error Out"=w313:errorcluster, "Output"=w312:T4)  [unwired: 8 in]
              }
            }
            n133 = local write "1-4"(w273) -> ()
            n134 = Bundle By Name(cluster=w275, "1-4"=w273) -> (w274:T13)
          }
          event Value Change {
            n135 = event-data() -> ("NewVal"=w320:T8)  [unwired: 1 in, 5 out]
            n136 = case shown="\"Standard ETPs\", \"Cancel Test\", Default" w320 {
              selector: w320 -> [w322 _ _ _ _ _ _ _ _]
              tunnel: [w321 w328 w332 w336 w340 w344 w347 w350 w354] -> w314
              tunnel: w319 -> [w324 w327 w331 w335 w339 w343 w346 w351 w353]
              tunnel: [w324 w326 w330 w334 w338 w342 w348 w352 w353] -> w318
              frame "Standard ETPs", "Cancel Test", Default {
                n137 = Bundle By Name(cluster=T4 {"Chamber 1-3"=[], "Chamber 1-2"=[], "Chamber 1-1"=[], "Standard Tests 1-1"=enum."Standard ETPs"} ("1-1"), "Standard Tests 1-1"=w322) -> (w321:T4)
              }
              frame "511-B113 EHUT" {
                # "This is basically a 14 HUT"
                n138 = local read "EHUT (511-B113)"() -> (w325:T4)
                n139 = call "RTS Standard Test Set Time.vi"("Error In"=w327, "Internal Moisture Test (511-B111) - 5 Days"=w325) -> ("Error Out"=w326:errorcluster, "Output"=w328:T4)  [unwired: 8 in]
              }
              frame "511-B110 HUT" {
                # "24 Hr HUT"
                n140 = local read "HUT (511-B110)"() -> (w329:T4)
                n141 = call "RTS Standard Test Set Time.vi"("Error In"=w331, "Internal Moisture Test (511-B111) - 5 Days"=w329) -> ("Error Out"=w330:errorcluster, "Output"=w332:T4)  [unwired: 8 in]
              }
              frame "512-C410 SLAT" {
                n142 = local read "SLAT (512-C419)"() -> (w333:T4)
                n143 = call "RTS Standard Test Set Time.vi"("Error In"=w335, "Internal Moisture Test (511-B111) - 5 Days"=w333) -> ("Error Out"=w334:errorcluster, "Output"=w336:T4)  [unwired: 8 in]
              }
              frame "511-B111 Internal Moisture" {
                # "This is a 5 day HUT"
                n144 = local read "Internal Moisture Test (511-B111) - 5 Days"() -> (w337:T4)
                n145 = call "RTS Standard Test Set Time.vi"("Error In"=w339, "Internal Moisture Test (511-B111) - 5 Days"=w337) -> ("Error Out"=w338:errorcluster, "Output"=w340:T4)  [unwired: 8 in]
              }
              frame "511-C401 Moisture Accumulation" {
                n146 = local read "Moisture Accumulation (511-C401)"() -> (w341:T4)
                n147 = call "RTS Standard Test Set Time.vi"("Error In"=w343, "Internal Moisture Test (511-B111) - 5 Days"=w341) -> ("Error Out"=w342:errorcluster, "Output"=w344:T4)  [unwired: 8 in]
              }
              frame "511-B100 No Door Opening (NDO)" {
                n148 = local read "NDO"() -> (w345:T4)
                n149 = call "RTS Standard Test Set Time.vi"("Error In"=w346, "Internal Moisture Test (511-B111) - 5 Days"=w345) -> ("Error Out"=w348:errorcluster, "Output"=w347:T4)  [unwired: 8 in]
              }
              frame "511-B304 ISO Energy Consumption" {
                n150 = local read "ISO Energy Consumption"() -> (w349:T4)
                n151 = call "RTS Standard Test Set Time.vi"("Error In"=w351, "Internal Moisture Test (511-B111) - 5 Days"=w349) -> ("Error Out"=w352:errorcluster, "Output"=w350:T4)  [unwired: 8 in]
              }
              frame "Custom Test" {
                n152 = local read "1-5"() -> (w354:T4)
              }
            }
            n153 = local write "1-5"(w314) -> ()
            n154 = Bundle By Name(cluster=w316, "1-5"=w314) -> (w315:T13)
          }
          event Value Change {
            n155 = event-data() -> ("NewVal"=w361:T8)  [unwired: 1 in, 5 out]
            n156 = case shown="\"Standard ETPs\", \"Cancel Test\", Default" w361 {
              selector: w361 -> [w363 _ _ _ _ _ _ _ _]
              tunnel: [w362 w369 w373 w377 w381 w385 w387 w391 w394] -> w355
              tunnel: w360 -> [w365 w368 w372 w376 w380 w384 w389 w390 w393]
              tunnel: [w365 w367 w371 w375 w379 w383 w388 w390 w395] -> w359
              frame "Standard ETPs", "Cancel Test", Default {
                n157 = Bundle By Name(cluster=T4 {"Chamber 1-3"=[], "Chamber 1-2"=[], "Chamber 1-1"=[], "Standard Tests 1-1"=enum."Standard ETPs"} ("1-1"), "Standard Tests 1-1"=w363) -> (w362:T4)
              }
              frame "511-B113 EHUT" {
                # "This is basically a 14 HUT"
                n158 = local read "EHUT (511-B113)"() -> (w366:T4)
                n159 = call "RTS Standard Test Set Time.vi"("Error In"=w368, "Internal Moisture Test (511-B111) - 5 Days"=w366) -> ("Error Out"=w367:errorcluster, "Output"=w369:T4)  [unwired: 8 in]
              }
              frame "511-B110 HUT" {
                # "24 Hr HUT"
                n160 = local read "HUT (511-B110)"() -> (w370:T4)
                n161 = call "RTS Standard Test Set Time.vi"("Error In"=w372, "Internal Moisture Test (511-B111) - 5 Days"=w370) -> ("Error Out"=w371:errorcluster, "Output"=w373:T4)  [unwired: 8 in]
              }
              frame "512-C410 SLAT" {
                n162 = local read "SLAT (512-C419)"() -> (w374:T4)
                n163 = call "RTS Standard Test Set Time.vi"("Error In"=w376, "Internal Moisture Test (511-B111) - 5 Days"=w374) -> ("Error Out"=w375:errorcluster, "Output"=w377:T4)  [unwired: 8 in]
              }
              frame "511-B111 Internal Moisture" {
                # "This is a 5 day HUT"
                n164 = local read "Internal Moisture Test (511-B111) - 5 Days"() -> (w378:T4)
                n165 = call "RTS Standard Test Set Time.vi"("Error In"=w380, "Internal Moisture Test (511-B111) - 5 Days"=w378) -> ("Error Out"=w379:errorcluster, "Output"=w381:T4)  [unwired: 8 in]
              }
              frame "511-C401 Moisture Accumulation" {
                n166 = local read "Moisture Accumulation (511-C401)"() -> (w382:T4)
                n167 = call "RTS Standard Test Set Time.vi"("Error In"=w384, "Internal Moisture Test (511-B111) - 5 Days"=w382) -> ("Error Out"=w383:errorcluster, "Output"=w385:T4)  [unwired: 8 in]
              }
              frame "511-B100 No Door Opening (NDO)" {
                n168 = local read "NDO"() -> (w386:T4)
                n169 = call "RTS Standard Test Set Time.vi"("Error In"=w389, "Internal Moisture Test (511-B111) - 5 Days"=w386) -> ("Error Out"=w388:errorcluster, "Output"=w387:T4)  [unwired: 8 in]
              }
              frame "Custom Test" {
                n170 = local read "1-6"() -> (w391:T4)
              }
              frame "511-B304 ISO Energy Consumption" {
                n171 = local read "ISO Energy Consumption"() -> (w392:T4)
                n172 = call "RTS Standard Test Set Time.vi"("Error In"=w393, "Internal Moisture Test (511-B111) - 5 Days"=w392) -> ("Error Out"=w395:errorcluster, "Output"=w394:T4)  [unwired: 8 in]
              }
            }
            n173 = local write "1-6"(w355) -> ()
            n174 = Bundle By Name(cluster=w357, "1-6"=w355) -> (w356:T13)
          }
          event Value Change {
            n175 = event-data() -> ("NewVal"=w402:T8)  [unwired: 1 in, 5 out]
            n176 = case shown="\"Standard ETPs\", \"Cancel Test\", Default" w402 {
              selector: w402 -> [w403 _ _ _ _ _ _ _ _]
              tunnel: [w404 w410 w414 w418 w422 w426 w428 w433 w436] -> w396
              tunnel: w401 -> [w406 w409 w413 w417 w421 w425 w429 w432 w435]
              tunnel: [w406 w408 w412 w416 w420 w424 w430 w434 w435] -> w400
              frame "Standard ETPs", "Cancel Test", Default {
                n177 = Bundle By Name(cluster=T4 {"Chamber 1-3"=[], "Chamber 1-2"=[], "Chamber 1-1"=[], "Standard Tests 1-1"=enum."Standard ETPs"} ("1-1"), "Standard Tests 1-1"=w403) -> (w404:T4)
              }
              frame "511-B113 EHUT" {
                # "This is basically a 14 HUT"
                n178 = local read "EHUT (511-B113)"() -> (w407:T4)
                n179 = call "RTS Standard Test Set Time.vi"("Error In"=w409, "Internal Moisture Test (511-B111) - 5 Days"=w407) -> ("Error Out"=w408:errorcluster, "Output"=w410:T4)  [unwired: 8 in]
              }
              frame "511-B110 HUT" {
                # "24 Hr HUT"
                n180 = local read "HUT (511-B110)"() -> (w411:T4)
                n181 = call "RTS Standard Test Set Time.vi"("Error In"=w413, "Internal Moisture Test (511-B111) - 5 Days"=w411) -> ("Error Out"=w412:errorcluster, "Output"=w414:T4)  [unwired: 8 in]
              }
              frame "512-C410 SLAT" {
                n182 = local read "SLAT (512-C419)"() -> (w415:T4)
                n183 = call "RTS Standard Test Set Time.vi"("Error In"=w417, "Internal Moisture Test (511-B111) - 5 Days"=w415) -> ("Error Out"=w416:errorcluster, "Output"=w418:T4)  [unwired: 8 in]
              }
              frame "511-B111 Internal Moisture" {
                # "This is a 5 day HUT"
                n184 = local read "Internal Moisture Test (511-B111) - 5 Days"() -> (w419:T4)
                n185 = call "RTS Standard Test Set Time.vi"("Error In"=w421, "Internal Moisture Test (511-B111) - 5 Days"=w419) -> ("Error Out"=w420:errorcluster, "Output"=w422:T4)  [unwired: 8 in]
              }
              frame "511-C401 Moisture Accumulation" {
                n186 = local read "Moisture Accumulation (511-C401)"() -> (w423:T4)
                n187 = call "RTS Standard Test Set Time.vi"("Error In"=w425, "Internal Moisture Test (511-B111) - 5 Days"=w423) -> ("Error Out"=w424:errorcluster, "Output"=w426:T4)  [unwired: 8 in]
              }
              frame "511-B100 No Door Opening (NDO)" {
                n188 = local read "NDO"() -> (w427:T4)
                n189 = call "RTS Standard Test Set Time.vi"("Error In"=w429, "Internal Moisture Test (511-B111) - 5 Days"=w427) -> ("Error Out"=w430:errorcluster, "Output"=w428:T4)  [unwired: 8 in]
              }
              frame "511-B304 ISO Energy Consumption" {
                n190 = local read "ISO Energy Consumption"() -> (w431:T4)
                n191 = call "RTS Standard Test Set Time.vi"("Error In"=w432, "Internal Moisture Test (511-B111) - 5 Days"=w431) -> ("Error Out"=w434:errorcluster, "Output"=w433:T4)  [unwired: 8 in]
              }
              frame "Custom Test" {
                n192 = local read "1-7"() -> (w436:T4)
              }
            }
            n193 = local write "1-7"(w396) -> ()
            n194 = Bundle By Name(cluster=w398, "1-7"=w396) -> (w397:T13)
          }
          event Value Change {
            n195 = event-data() -> ("NewVal"=w443:T8)  [unwired: 1 in, 5 out]
            n196 = case shown="\"Standard ETPs\", \"Cancel Test\", Default" w443 {
              selector: w443 -> [w444 _ _ _ _ _ _ _ _]
              tunnel: [w445 w451 w455 w459 w463 w467 w470 w473 w477] -> w437
              tunnel: w441 -> [w447 w450 w454 w458 w462 w466 w468 w474 w476]
              tunnel: [w447 w449 w453 w457 w461 w465 w471 w475 w476] -> w440
              frame "Standard ETPs", "Cancel Test", Default {
                n197 = Bundle By Name(cluster=T4 {"Chamber 1-3"=[], "Chamber 1-2"=[], "Chamber 1-1"=[], "Standard Tests 1-1"=enum."Standard ETPs"} ("1-1"), "Standard Tests 1-1"=w444) -> (w445:T4)
              }
              frame "511-B113 EHUT" {
                # "This is basically a 14 HUT"
                n198 = local read "EHUT (511-B113)"() -> (w448:T4)
                n199 = call "RTS Standard Test Set Time.vi"("Error In"=w450, "Internal Moisture Test (511-B111) - 5 Days"=w448) -> ("Error Out"=w449:errorcluster, "Output"=w451:T4)  [unwired: 8 in]
              }
              frame "511-B110 HUT" {
                # "24 Hr HUT"
                n200 = local read "HUT (511-B110)"() -> (w452:T4)
                n201 = call "RTS Standard Test Set Time.vi"("Error In"=w454, "Internal Moisture Test (511-B111) - 5 Days"=w452) -> ("Error Out"=w453:errorcluster, "Output"=w455:T4)  [unwired: 8 in]
              }
              frame "512-C410 SLAT" {
                n202 = local read "SLAT (512-C419)"() -> (w456:T4)
                n203 = call "RTS Standard Test Set Time.vi"("Error In"=w458, "Internal Moisture Test (511-B111) - 5 Days"=w456) -> ("Error Out"=w457:errorcluster, "Output"=w459:T4)  [unwired: 8 in]
              }
              frame "511-B111 Internal Moisture" {
                # "This is a 5 day HUT"
                n204 = local read "Internal Moisture Test (511-B111) - 5 Days"() -> (w460:T4)
                n205 = call "RTS Standard Test Set Time.vi"("Error In"=w462, "Internal Moisture Test (511-B111) - 5 Days"=w460) -> ("Error Out"=w461:errorcluster, "Output"=w463:T4)  [unwired: 8 in]
              }
              frame "511-C401 Moisture Accumulation" {
                n206 = local read "Moisture Accumulation (511-C401)"() -> (w464:T4)
                n207 = call "RTS Standard Test Set Time.vi"("Error In"=w466, "Internal Moisture Test (511-B111) - 5 Days"=w464) -> ("Error Out"=w465:errorcluster, "Output"=w467:T4)  [unwired: 8 in]
              }
              frame "511-B100 No Door Opening (NDO)" {
                n208 = local read "NDO"() -> (w469:T4)
                n209 = call "RTS Standard Test Set Time.vi"("Error In"=w468, "Internal Moisture Test (511-B111) - 5 Days"=w469) -> ("Error Out"=w471:errorcluster, "Output"=w470:T4)  [unwired: 8 in]
              }
              frame "511-B304 ISO Energy Consumption" {
                n210 = local read "ISO Energy Consumption"() -> (w472:T4)
                n211 = call "RTS Standard Test Set Time.vi"("Error In"=w474, "Internal Moisture Test (511-B111) - 5 Days"=w472) -> ("Error Out"=w475:errorcluster, "Output"=w473:T4)  [unwired: 8 in]
              }
              frame "Custom Test" {
                n212 = local read "1-8"() -> (w477:T4)
              }
            }
            n213 = local write "1-8"(w437) -> ()
            n214 = Bundle By Name(cluster=w439, "1-8"=w437) -> (w438:T13)
          }
          event Value Change {
            n215 = event-data() -> ("NewVal"=w484:T8)  [unwired: 1 in, 5 out]
            n216 = case shown="\"Standard ETPs\", \"Cancel Test\", Default" w484 {
              selector: w484 -> [w486 _ _ _ _ _ _ _ _]
              tunnel: [w485 w492 w496 w500 w504 w508 w511 w515 w518] -> w478
              tunnel: w482 -> [w488 w491 w495 w499 w503 w507 w510 w514 w517]
              tunnel: [w488 w490 w494 w498 w502 w506 w512 w516 w517] -> w481
              frame "Standard ETPs", "Cancel Test", Default {
                n217 = Bundle By Name(cluster=T4 {"Chamber 1-3"=[], "Chamber 1-2"=[], "Chamber 1-1"=[], "Standard Tests 1-1"=enum."Standard ETPs"} ("1-1"), "Standard Tests 1-1"=w486) -> (w485:T4)
              }
              frame "511-B113 EHUT" {
                # "This is basically a 14 HUT"
                n218 = local read "EHUT (511-B113)"() -> (w489:T4)
                n219 = call "RTS Standard Test Set Time.vi"("Error In"=w491, "Internal Moisture Test (511-B111) - 5 Days"=w489) -> ("Error Out"=w490:errorcluster, "Output"=w492:T4)  [unwired: 8 in]
              }
              frame "511-B110 HUT" {
                # "24 Hr HUT"
                n220 = local read "HUT (511-B110)"() -> (w493:T4)
                n221 = call "RTS Standard Test Set Time.vi"("Error In"=w495, "Internal Moisture Test (511-B111) - 5 Days"=w493) -> ("Error Out"=w494:errorcluster, "Output"=w496:T4)  [unwired: 8 in]
              }
              frame "512-C410 SLAT" {
                n222 = local read "SLAT (512-C419)"() -> (w497:T4)
                n223 = call "RTS Standard Test Set Time.vi"("Error In"=w499, "Internal Moisture Test (511-B111) - 5 Days"=w497) -> ("Error Out"=w498:errorcluster, "Output"=w500:T4)  [unwired: 8 in]
              }
              frame "511-B111 Internal Moisture" {
                # "This is a 5 day HUT"
                n224 = local read "Internal Moisture Test (511-B111) - 5 Days"() -> (w501:T4)
                n225 = call "RTS Standard Test Set Time.vi"("Error In"=w503, "Internal Moisture Test (511-B111) - 5 Days"=w501) -> ("Error Out"=w502:errorcluster, "Output"=w504:T4)  [unwired: 8 in]
              }
              frame "511-C401 Moisture Accumulation" {
                n226 = local read "Moisture Accumulation (511-C401)"() -> (w505:T4)
                n227 = call "RTS Standard Test Set Time.vi"("Error In"=w507, "Internal Moisture Test (511-B111) - 5 Days"=w505) -> ("Error Out"=w506:errorcluster, "Output"=w508:T4)  [unwired: 8 in]
              }
              frame "511-B100 No Door Opening (NDO)" {
                n228 = local read "NDO"() -> (w509:T4)
                n229 = call "RTS Standard Test Set Time.vi"("Error In"=w510, "Internal Moisture Test (511-B111) - 5 Days"=w509) -> ("Error Out"=w512:errorcluster, "Output"=w511:T4)  [unwired: 8 in]
              }
              frame "511-B304 ISO Energy Consumption" {
                n230 = local read "ISO Energy Consumption"() -> (w513:T4)
                n231 = call "RTS Standard Test Set Time.vi"("Error In"=w514, "Internal Moisture Test (511-B111) - 5 Days"=w513) -> ("Error Out"=w516:errorcluster, "Output"=w515:T4)  [unwired: 8 in]
              }
              frame "Custom Test" {
                n232 = local read "2-1"() -> (w518:T4)
              }
            }
            n233 = local write "2-1"(w478) -> ()
            n234 = Bundle By Name(cluster=w480, "2-1"=w478) -> (w479:T13)
          }
          event Value Change {
            n235 = event-data() -> ("NewVal"=w525:T8)  [unwired: 1 in, 5 out]
            n236 = case shown="\"Standard ETPs\", \"Cancel Test\", Default" w525 {
              selector: w525 -> [w527 _ _ _ _ _ _ _ _]
              tunnel: [w526 w533 w537 w541 w545 w549 w551 w556 w559] -> w519
              tunnel: w523 -> [w529 w532 w536 w540 w544 w548 w553 w555 w558]
              tunnel: [w529 w531 w535 w539 w543 w547 w552 w557 w558] -> w522
              frame "Standard ETPs", "Cancel Test", Default {
                n237 = Bundle By Name(cluster=T4 {"Chamber 1-3"=[], "Chamber 1-2"=[], "Chamber 1-1"=[], "Standard Tests 1-1"=enum."Standard ETPs"} ("1-1"), "Standard Tests 1-1"=w527) -> (w526:T4)
              }
              frame "511-B113 EHUT" {
                # "This is basically a 14 HUT"
                n238 = local read "EHUT (511-B113)"() -> (w530:T4)
                n239 = call "RTS Standard Test Set Time.vi"("Error In"=w532, "Internal Moisture Test (511-B111) - 5 Days"=w530) -> ("Error Out"=w531:errorcluster, "Output"=w533:T4)  [unwired: 8 in]
              }
              frame "511-B110 HUT" {
                # "24 Hr HUT"
                n240 = local read "HUT (511-B110)"() -> (w534:T4)
                n241 = call "RTS Standard Test Set Time.vi"("Error In"=w536, "Internal Moisture Test (511-B111) - 5 Days"=w534) -> ("Error Out"=w535:errorcluster, "Output"=w537:T4)  [unwired: 8 in]
              }
              frame "512-C410 SLAT" {
                n242 = local read "SLAT (512-C419)"() -> (w538:T4)
                n243 = call "RTS Standard Test Set Time.vi"("Error In"=w540, "Internal Moisture Test (511-B111) - 5 Days"=w538) -> ("Error Out"=w539:errorcluster, "Output"=w541:T4)  [unwired: 8 in]
              }
              frame "511-B111 Internal Moisture" {
                # "This is a 5 day HUT"
                n244 = local read "Internal Moisture Test (511-B111) - 5 Days"() -> (w542:T4)
                n245 = call "RTS Standard Test Set Time.vi"("Error In"=w544, "Internal Moisture Test (511-B111) - 5 Days"=w542) -> ("Error Out"=w543:errorcluster, "Output"=w545:T4)  [unwired: 8 in]
              }
              frame "511-C401 Moisture Accumulation" {
                n246 = local read "Moisture Accumulation (511-C401)"() -> (w546:T4)
                n247 = call "RTS Standard Test Set Time.vi"("Error In"=w548, "Internal Moisture Test (511-B111) - 5 Days"=w546) -> ("Error Out"=w547:errorcluster, "Output"=w549:T4)  [unwired: 8 in]
              }
              frame "511-B100 No Door Opening (NDO)" {
                n248 = local read "NDO"() -> (w550:T4)
                n249 = call "RTS Standard Test Set Time.vi"("Error In"=w553, "Internal Moisture Test (511-B111) - 5 Days"=w550) -> ("Error Out"=w552:errorcluster, "Output"=w551:T4)  [unwired: 8 in]
              }
              frame "511-B304 ISO Energy Consumption" {
                n250 = local read "ISO Energy Consumption"() -> (w554:T4)
                n251 = call "RTS Standard Test Set Time.vi"("Error In"=w555, "Internal Moisture Test (511-B111) - 5 Days"=w554) -> ("Error Out"=w557:errorcluster, "Output"=w556:T4)  [unwired: 8 in]
              }
              frame "Custom Test" {
                n252 = local read "2-2"() -> (w559:T4)
              }
            }
            n253 = local write "2-2"(w519) -> ()
            n254 = Bundle By Name(cluster=w521, "2-2"=w519) -> (w520:T13)
          }
          event Value Change {
            n255 = event-data() -> ("NewVal"=w566:T8)  [unwired: 1 in, 5 out]
            n256 = case shown="\"Standard ETPs\", \"Cancel Test\", Default" w566 {
              selector: w566 -> [w569 _ _ _ _ _ _ _ _]
              tunnel: [w567 w574 w578 w582 w586 w590 w592 w596 w600] -> w560
              tunnel: w565 -> [w570 w573 w577 w581 w585 w589 w593 w597 w599]
              tunnel: [w570 w572 w576 w580 w584 w588 w594 w598 w599] -> w564
              frame "Standard ETPs", "Cancel Test", Default {
                n257 = Bundle By Name(cluster=T4 {"Chamber 1-3"=[], "Chamber 1-2"=[], "Chamber 1-1"=[], "Standard Tests 1-1"=enum."Standard ETPs"} ("1-1"), "Standard Tests 1-1"=w569) -> (w567:T4)
              }
              frame "511-B113 EHUT" {
                # "This is basically a 14 HUT"
                n258 = local read "EHUT (511-B113)"() -> (w571:T4)
                n259 = call "RTS Standard Test Set Time.vi"("Error In"=w573, "Internal Moisture Test (511-B111) - 5 Days"=w571) -> ("Error Out"=w572:errorcluster, "Output"=w574:T4)  [unwired: 8 in]
              }
              frame "511-B110 HUT" {
                # "24 Hr HUT"
                n260 = local read "HUT (511-B110)"() -> (w575:T4)
                n261 = call "RTS Standard Test Set Time.vi"("Error In"=w577, "Internal Moisture Test (511-B111) - 5 Days"=w575) -> ("Error Out"=w576:errorcluster, "Output"=w578:T4)  [unwired: 8 in]
              }
              frame "512-C410 SLAT" {
                n262 = local read "SLAT (512-C419)"() -> (w579:T4)
                n263 = call "RTS Standard Test Set Time.vi"("Error In"=w581, "Internal Moisture Test (511-B111) - 5 Days"=w579) -> ("Error Out"=w580:errorcluster, "Output"=w582:T4)  [unwired: 8 in]
              }
              frame "511-B111 Internal Moisture" {
                # "This is a 5 day HUT"
                n264 = local read "Internal Moisture Test (511-B111) - 5 Days"() -> (w583:T4)
                n265 = call "RTS Standard Test Set Time.vi"("Error In"=w585, "Internal Moisture Test (511-B111) - 5 Days"=w583) -> ("Error Out"=w584:errorcluster, "Output"=w586:T4)  [unwired: 8 in]
              }
              frame "511-C401 Moisture Accumulation" {
                n266 = local read "Moisture Accumulation (511-C401)"() -> (w587:T4)
                n267 = call "RTS Standard Test Set Time.vi"("Error In"=w589, "Internal Moisture Test (511-B111) - 5 Days"=w587) -> ("Error Out"=w588:errorcluster, "Output"=w590:T4)  [unwired: 8 in]
              }
              frame "511-B100 No Door Opening (NDO)" {
                n268 = local read "NDO"() -> (w591:T4)
                n269 = call "RTS Standard Test Set Time.vi"("Error In"=w593, "Internal Moisture Test (511-B111) - 5 Days"=w591) -> ("Error Out"=w594:errorcluster, "Output"=w592:T4)  [unwired: 8 in]
              }
              frame "511-B304 ISO Energy Consumption" {
                n270 = local read "ISO Energy Consumption"() -> (w595:T4)
                n271 = call "RTS Standard Test Set Time.vi"("Error In"=w597, "Internal Moisture Test (511-B111) - 5 Days"=w595) -> ("Error Out"=w598:errorcluster, "Output"=w596:T4)  [unwired: 8 in]
              }
              frame "Custom Test" {
                n272 = local read "2-3"() -> (w600:T4)
              }
            }
            n273 = local write "2-3"(w560) -> ()
            n274 = Bundle By Name(cluster=w562, "2-3"=w560) -> (w561:T13)
          }
          event Value Change {
            n275 = event-data() -> ("NewVal"=w607:T8)  [unwired: 1 in, 5 out]
            n276 = case shown="\"Standard ETPs\", \"Cancel Test\", Default" w607 {
              selector: w607 -> [w608 _ _ _ _ _ _ _ _]
              tunnel: [w609 w615 w619 w623 w627 w631 w633 w639 w641] -> w601
              tunnel: w605 -> [w611 w614 w618 w622 w626 w630 w634 w637 w640]
              tunnel: [w611 w613 w617 w621 w625 w629 w635 w638 w640] -> w604
              frame "Standard ETPs", "Cancel Test", Default {
                n277 = Bundle By Name(cluster=T4 {"Chamber 1-3"=[], "Chamber 1-2"=[], "Chamber 1-1"=[], "Standard Tests 1-1"=enum."Standard ETPs"} ("1-1"), "Standard Tests 1-1"=w608) -> (w609:T4)
              }
              frame "511-B113 EHUT" {
                # "This is basically a 14 HUT"
                n278 = local read "EHUT (511-B113)"() -> (w612:T4)
                n279 = call "RTS Standard Test Set Time.vi"("Error In"=w614, "Internal Moisture Test (511-B111) - 5 Days"=w612) -> ("Error Out"=w613:errorcluster, "Output"=w615:T4)  [unwired: 8 in]
              }
              frame "511-B110 HUT" {
                # "24 Hr HUT"
                n280 = local read "HUT (511-B110)"() -> (w616:T4)
                n281 = call "RTS Standard Test Set Time.vi"("Error In"=w618, "Internal Moisture Test (511-B111) - 5 Days"=w616) -> ("Error Out"=w617:errorcluster, "Output"=w619:T4)  [unwired: 8 in]
              }
              frame "512-C410 SLAT" {
                n282 = local read "SLAT (512-C419)"() -> (w620:T4)
                n283 = call "RTS Standard Test Set Time.vi"("Error In"=w622, "Internal Moisture Test (511-B111) - 5 Days"=w620) -> ("Error Out"=w621:errorcluster, "Output"=w623:T4)  [unwired: 8 in]
              }
              frame "511-B111 Internal Moisture" {
                # "This is a 5 day HUT"
                n284 = local read "Internal Moisture Test (511-B111) - 5 Days"() -> (w624:T4)
                n285 = call "RTS Standard Test Set Time.vi"("Error In"=w626, "Internal Moisture Test (511-B111) - 5 Days"=w624) -> ("Error Out"=w625:errorcluster, "Output"=w627:T4)  [unwired: 8 in]
              }
              frame "511-C401 Moisture Accumulation" {
                n286 = local read "Moisture Accumulation (511-C401)"() -> (w628:T4)
                n287 = call "RTS Standard Test Set Time.vi"("Error In"=w630, "Internal Moisture Test (511-B111) - 5 Days"=w628) -> ("Error Out"=w629:errorcluster, "Output"=w631:T4)  [unwired: 8 in]
              }
              frame "511-B100 No Door Opening (NDO)" {
                n288 = local read "NDO"() -> (w632:T4)
                n289 = call "RTS Standard Test Set Time.vi"("Error In"=w634, "Internal Moisture Test (511-B111) - 5 Days"=w632) -> ("Error Out"=w635:errorcluster, "Output"=w633:T4)  [unwired: 8 in]
              }
              frame "511-B304 ISO Energy Consumption" {
                n290 = local read "ISO Energy Consumption"() -> (w636:T4)
                n291 = call "RTS Standard Test Set Time.vi"("Error In"=w637, "Internal Moisture Test (511-B111) - 5 Days"=w636) -> ("Error Out"=w638:errorcluster, "Output"=w639:T4)  [unwired: 8 in]
              }
              frame "Custom Test" {
                n292 = local read "2-4"() -> (w641:T4)
              }
            }
            n293 = local write "2-4"(w601) -> ()
            n294 = Bundle By Name(cluster=w603, "2-4"=w601) -> (w602:T13)
          }
          event Value Change {
            n295 = event-data() -> ("NewVal"=w648:T8)  [unwired: 1 in, 5 out]
            n296 = case shown="\"Standard ETPs\", \"Cancel Test\", Default" w648 {
              selector: w648 -> [w650 _ _ _ _ _ _ _ _]
              tunnel: [w649 w656 w660 w664 w668 w672 w675 w680 w682] -> w642
              tunnel: w647 -> [w652 w655 w659 w663 w667 w671 w674 w678 w681]
              tunnel: [w652 w654 w658 w662 w666 w670 w676 w679 w681] -> w646
              frame "Standard ETPs", "Cancel Test", Default {
                n297 = Bundle By Name(cluster=T4 {"Chamber 1-3"=[], "Chamber 1-2"=[], "Chamber 1-1"=[], "Standard Tests 1-1"=enum."Standard ETPs"} ("1-1"), "Standard Tests 1-1"=w650) -> (w649:T4)
              }
              frame "511-B113 EHUT" {
                # "This is basically a 14 HUT"
                n298 = local read "EHUT (511-B113)"() -> (w653:T4)
                n299 = call "RTS Standard Test Set Time.vi"("Error In"=w655, "Internal Moisture Test (511-B111) - 5 Days"=w653) -> ("Error Out"=w654:errorcluster, "Output"=w656:T4)  [unwired: 8 in]
              }
              frame "511-B110 HUT" {
                # "24 Hr HUT"
                n300 = local read "HUT (511-B110)"() -> (w657:T4)
                n301 = call "RTS Standard Test Set Time.vi"("Error In"=w659, "Internal Moisture Test (511-B111) - 5 Days"=w657) -> ("Error Out"=w658:errorcluster, "Output"=w660:T4)  [unwired: 8 in]
              }
              frame "512-C410 SLAT" {
                n302 = local read "SLAT (512-C419)"() -> (w661:T4)
                n303 = call "RTS Standard Test Set Time.vi"("Error In"=w663, "Internal Moisture Test (511-B111) - 5 Days"=w661) -> ("Error Out"=w662:errorcluster, "Output"=w664:T4)  [unwired: 8 in]
              }
              frame "511-B111 Internal Moisture" {
                # "This is a 5 day HUT"
                n304 = local read "Internal Moisture Test (511-B111) - 5 Days"() -> (w665:T4)
                n305 = call "RTS Standard Test Set Time.vi"("Error In"=w667, "Internal Moisture Test (511-B111) - 5 Days"=w665) -> ("Error Out"=w666:errorcluster, "Output"=w668:T4)  [unwired: 8 in]
              }
              frame "511-C401 Moisture Accumulation" {
                n306 = local read "Moisture Accumulation (511-C401)"() -> (w669:T4)
                n307 = call "RTS Standard Test Set Time.vi"("Error In"=w671, "Internal Moisture Test (511-B111) - 5 Days"=w669) -> ("Error Out"=w670:errorcluster, "Output"=w672:T4)  [unwired: 8 in]
              }
              frame "511-B100 No Door Opening (NDO)" {
                n308 = local read "NDO"() -> (w673:T4)
                n309 = call "RTS Standard Test Set Time.vi"("Error In"=w674, "Internal Moisture Test (511-B111) - 5 Days"=w673) -> ("Error Out"=w676:errorcluster, "Output"=w675:T4)  [unwired: 8 in]
              }
              frame "511-B304 ISO Energy Consumption" {
                n310 = local read "ISO Energy Consumption"() -> (w677:T4)
                n311 = call "RTS Standard Test Set Time.vi"("Error In"=w678, "Internal Moisture Test (511-B111) - 5 Days"=w677) -> ("Error Out"=w679:errorcluster, "Output"=w680:T4)  [unwired: 8 in]
              }
              frame "Custom Test" {
                n312 = local read "2-5"() -> (w682:T4)
              }
            }
            n313 = local write "2-5"(w642) -> ()
            n314 = Bundle By Name(cluster=w644, "2-5"=w642) -> (w643:T13)
          }
          event Value Change {
            n315 = event-data() -> ("NewVal"=w689:T8)  [unwired: 1 in, 5 out]
            n316 = case shown="\"Standard ETPs\", \"Cancel Test\", Default" w689 {
              selector: w689 -> [w690 _ _ _ _ _ _ _ _]
              tunnel: [w692 w697 w701 w705 w709 w713 w716 w720 w723] -> w683
              tunnel: w688 -> [w693 w696 w700 w704 w708 w712 w715 w719 w722]
              tunnel: [w693 w695 w699 w703 w707 w711 w717 w721 w722] -> w687
              frame "Standard ETPs", "Cancel Test", Default {
                n317 = Bundle By Name(cluster=T4 {"Chamber 1-3"=[], "Chamber 1-2"=[], "Chamber 1-1"=[], "Standard Tests 1-1"=enum."Standard ETPs"} ("1-1"), "Standard Tests 1-1"=w690) -> (w692:T4)
              }
              frame "511-B113 EHUT" {
                # "This is basically a 14 HUT"
                n318 = local read "EHUT (511-B113)"() -> (w694:T4)
                n319 = call "RTS Standard Test Set Time.vi"("Error In"=w696, "Internal Moisture Test (511-B111) - 5 Days"=w694) -> ("Error Out"=w695:errorcluster, "Output"=w697:T4)  [unwired: 8 in]
              }
              frame "511-B110 HUT" {
                # "24 Hr HUT"
                n320 = local read "HUT (511-B110)"() -> (w698:T4)
                n321 = call "RTS Standard Test Set Time.vi"("Error In"=w700, "Internal Moisture Test (511-B111) - 5 Days"=w698) -> ("Error Out"=w699:errorcluster, "Output"=w701:T4)  [unwired: 8 in]
              }
              frame "512-C410 SLAT" {
                n322 = local read "SLAT (512-C419)"() -> (w702:T4)
                n323 = call "RTS Standard Test Set Time.vi"("Error In"=w704, "Internal Moisture Test (511-B111) - 5 Days"=w702) -> ("Error Out"=w703:errorcluster, "Output"=w705:T4)  [unwired: 8 in]
              }
              frame "511-B111 Internal Moisture" {
                # "This is a 5 day HUT"
                n324 = local read "Internal Moisture Test (511-B111) - 5 Days"() -> (w706:T4)
                n325 = call "RTS Standard Test Set Time.vi"("Error In"=w708, "Internal Moisture Test (511-B111) - 5 Days"=w706) -> ("Error Out"=w707:errorcluster, "Output"=w709:T4)  [unwired: 8 in]
              }
              frame "511-C401 Moisture Accumulation" {
                n326 = local read "Moisture Accumulation (511-C401)"() -> (w710:T4)
                n327 = call "RTS Standard Test Set Time.vi"("Error In"=w712, "Internal Moisture Test (511-B111) - 5 Days"=w710) -> ("Error Out"=w711:errorcluster, "Output"=w713:T4)  [unwired: 8 in]
              }
              frame "511-B100 No Door Opening (NDO)" {
                n328 = local read "NDO"() -> (w714:T4)
                n329 = call "RTS Standard Test Set Time.vi"("Error In"=w715, "Internal Moisture Test (511-B111) - 5 Days"=w714) -> ("Error Out"=w717:errorcluster, "Output"=w716:T4)  [unwired: 8 in]
              }
              frame "511-B304 ISO Energy Consumption" {
                n330 = local read "ISO Energy Consumption"() -> (w718:T4)
                n331 = call "RTS Standard Test Set Time.vi"("Error In"=w719, "Internal Moisture Test (511-B111) - 5 Days"=w718) -> ("Error Out"=w721:errorcluster, "Output"=w720:T4)  [unwired: 8 in]
              }
              frame "Custom Test" {
                n332 = local read "2-6"() -> (w723:T4)
              }
            }
            n333 = local write "2-6"(w683) -> ()
            n334 = Bundle By Name(cluster=w685, "2-6"=w683) -> (w684:T13)
          }
          event Value Change {
            n335 = event-data() -> ("NewVal"=w730:T8)  [unwired: 1 in, 5 out]
            n336 = case shown="\"Standard ETPs\", \"Cancel Test\", Default" w730 {
              selector: w730 -> [w733 _ _ _ _ _ _ _ _]
              tunnel: [w731 w738 w742 w746 w750 w754 w757 w761 w764] -> w724
              tunnel: w728 -> [w734 w737 w741 w745 w749 w753 w756 w759 w763]
              tunnel: [w734 w736 w740 w744 w748 w752 w758 w762 w763] -> w727
              frame "Standard ETPs", "Cancel Test", Default {
                n337 = Bundle By Name(cluster=T4 {"Chamber 1-3"=[], "Chamber 1-2"=[], "Chamber 1-1"=[], "Standard Tests 1-1"=enum."Standard ETPs"} ("1-1"), "Standard Tests 1-1"=w733) -> (w731:T4)
              }
              frame "511-B113 EHUT" {
                # "This is basically a 14 HUT"
                n338 = local read "EHUT (511-B113)"() -> (w735:T4)
                n339 = call "RTS Standard Test Set Time.vi"("Error In"=w737, "Internal Moisture Test (511-B111) - 5 Days"=w735) -> ("Error Out"=w736:errorcluster, "Output"=w738:T4)  [unwired: 8 in]
              }
              frame "511-B110 HUT" {
                # "24 Hr HUT"
                n340 = local read "HUT (511-B110)"() -> (w739:T4)
                n341 = call "RTS Standard Test Set Time.vi"("Error In"=w741, "Internal Moisture Test (511-B111) - 5 Days"=w739) -> ("Error Out"=w740:errorcluster, "Output"=w742:T4)  [unwired: 8 in]
              }
              frame "512-C410 SLAT" {
                n342 = local read "SLAT (512-C419)"() -> (w743:T4)
                n343 = call "RTS Standard Test Set Time.vi"("Error In"=w745, "Internal Moisture Test (511-B111) - 5 Days"=w743) -> ("Error Out"=w744:errorcluster, "Output"=w746:T4)  [unwired: 8 in]
              }
              frame "511-B111 Internal Moisture" {
                # "This is a 5 day HUT"
                n344 = local read "Internal Moisture Test (511-B111) - 5 Days"() -> (w747:T4)
                n345 = call "RTS Standard Test Set Time.vi"("Error In"=w749, "Internal Moisture Test (511-B111) - 5 Days"=w747) -> ("Error Out"=w748:errorcluster, "Output"=w750:T4)  [unwired: 8 in]
              }
              frame "511-C401 Moisture Accumulation" {
                n346 = local read "Moisture Accumulation (511-C401)"() -> (w751:T4)
                n347 = call "RTS Standard Test Set Time.vi"("Error In"=w753, "Internal Moisture Test (511-B111) - 5 Days"=w751) -> ("Error Out"=w752:errorcluster, "Output"=w754:T4)  [unwired: 8 in]
              }
              frame "511-B100 No Door Opening (NDO)" {
                n348 = local read "NDO"() -> (w755:T4)
                n349 = call "RTS Standard Test Set Time.vi"("Error In"=w756, "Internal Moisture Test (511-B111) - 5 Days"=w755) -> ("Error Out"=w758:errorcluster, "Output"=w757:T4)  [unwired: 8 in]
              }
              frame "511-B304 ISO Energy Consumption" {
                n350 = local read "ISO Energy Consumption"() -> (w760:T4)
                n351 = call "RTS Standard Test Set Time.vi"("Error In"=w759, "Internal Moisture Test (511-B111) - 5 Days"=w760) -> ("Error Out"=w762:errorcluster, "Output"=w761:T4)  [unwired: 8 in]
              }
              frame "Custom Test" {
                n352 = local read "2-7"() -> (w764:T4)
              }
            }
            n353 = local write "2-7"(w724) -> ()
            n354 = Bundle By Name(cluster=w726, "2-7"=w724) -> (w725:T13)
          }
          event Value Change {
            n355 = event-data() -> ("NewVal"=w771:T8)  [unwired: 1 in, 5 out]
            n356 = case shown="\"Standard ETPs\", \"Cancel Test\", Default" w771 {
              selector: w771 -> [w772 _ _ _ _ _ _ _ _]
              tunnel: [w773 w779 w783 w787 w791 w795 w797 w802 w805] -> w765
              tunnel: w770 -> [w775 w778 w782 w786 w790 w794 w798 w801 w804]
              tunnel: [w775 w777 w781 w785 w789 w793 w799 w803 w804] -> w769
              frame "Standard ETPs", "Cancel Test", Default {
                n357 = Bundle By Name(cluster=T4 {"Chamber 1-3"=[], "Chamber 1-2"=[], "Chamber 1-1"=[], "Standard Tests 1-1"=enum."Standard ETPs"} ("1-1"), "Standard Tests 1-1"=w772) -> (w773:T4)
              }
              frame "511-B113 EHUT" {
                # "This is basically a 14 HUT"
                n358 = local read "EHUT (511-B113)"() -> (w776:T4)
                n359 = call "RTS Standard Test Set Time.vi"("Error In"=w778, "Internal Moisture Test (511-B111) - 5 Days"=w776) -> ("Error Out"=w777:errorcluster, "Output"=w779:T4)  [unwired: 8 in]
              }
              frame "511-B110 HUT" {
                # "24 Hr HUT"
                n360 = local read "HUT (511-B110)"() -> (w780:T4)
                n361 = call "RTS Standard Test Set Time.vi"("Error In"=w782, "Internal Moisture Test (511-B111) - 5 Days"=w780) -> ("Error Out"=w781:errorcluster, "Output"=w783:T4)  [unwired: 8 in]
              }
              frame "512-C410 SLAT" {
                n362 = local read "SLAT (512-C419)"() -> (w784:T4)
                n363 = call "RTS Standard Test Set Time.vi"("Error In"=w786, "Internal Moisture Test (511-B111) - 5 Days"=w784) -> ("Error Out"=w785:errorcluster, "Output"=w787:T4)  [unwired: 8 in]
              }
              frame "511-B111 Internal Moisture" {
                # "This is a 5 day HUT"
                n364 = local read "Internal Moisture Test (511-B111) - 5 Days"() -> (w788:T4)
                n365 = call "RTS Standard Test Set Time.vi"("Error In"=w790, "Internal Moisture Test (511-B111) - 5 Days"=w788) -> ("Error Out"=w789:errorcluster, "Output"=w791:T4)  [unwired: 8 in]
              }
              frame "511-C401 Moisture Accumulation" {
                n366 = local read "Moisture Accumulation (511-C401)"() -> (w792:T4)
                n367 = call "RTS Standard Test Set Time.vi"("Error In"=w794, "Internal Moisture Test (511-B111) - 5 Days"=w792) -> ("Error Out"=w793:errorcluster, "Output"=w795:T4)  [unwired: 8 in]
              }
              frame "511-B100 No Door Opening (NDO)" {
                n368 = local read "NDO"() -> (w796:T4)
                n369 = call "RTS Standard Test Set Time.vi"("Error In"=w798, "Internal Moisture Test (511-B111) - 5 Days"=w796) -> ("Error Out"=w799:errorcluster, "Output"=w797:T4)  [unwired: 8 in]
              }
              frame "511-B304 ISO Energy Consumption" {
                n370 = local read "ISO Energy Consumption"() -> (w800:T4)
                n371 = call "RTS Standard Test Set Time.vi"("Error In"=w801, "Internal Moisture Test (511-B111) - 5 Days"=w800) -> ("Error Out"=w803:errorcluster, "Output"=w802:T4)  [unwired: 8 in]
              }
              frame "Custom Test" {
                n372 = local read "2-8"() -> (w805:T4)
              }
            }
            n373 = local write "2-8"(w765) -> ()
            n374 = Bundle By Name(cluster=w767, "2-8"=w765) -> (w766:T13)
          }
          event Value Change {
            n375 = event-data() -> ("NewVal"=w812:T8)  [unwired: 1 in, 5 out]
            n376 = case shown="\"Standard ETPs\", \"Cancel Test\", Default" w812 {
              selector: w812 -> [w813 _ _ _ _ _ _ _ _]
              tunnel: [w814 w820 w824 w828 w832 w836 w839 w843 w846] -> w806
              tunnel: w810 -> [w816 w819 w823 w827 w831 w835 w838 w842 w845]
              tunnel: [w816 w818 w822 w826 w830 w834 w840 w844 w845] -> w809
              frame "Standard ETPs", "Cancel Test", Default {
                n377 = Bundle By Name(cluster=T4 {"Chamber 1-3"=[], "Chamber 1-2"=[], "Chamber 1-1"=[], "Standard Tests 1-1"=enum."Standard ETPs"} ("1-1"), "Standard Tests 1-1"=w813) -> (w814:T4)
              }
              frame "511-B113 EHUT" {
                # "This is basically a 14 HUT"
                n378 = local read "EHUT (511-B113)"() -> (w817:T4)
                n379 = call "RTS Standard Test Set Time.vi"("Error In"=w819, "Internal Moisture Test (511-B111) - 5 Days"=w817) -> ("Error Out"=w818:errorcluster, "Output"=w820:T4)  [unwired: 8 in]
              }
              frame "511-B110 HUT" {
                # "24 Hr HUT"
                n380 = local read "HUT (511-B110)"() -> (w821:T4)
                n381 = call "RTS Standard Test Set Time.vi"("Error In"=w823, "Internal Moisture Test (511-B111) - 5 Days"=w821) -> ("Error Out"=w822:errorcluster, "Output"=w824:T4)  [unwired: 8 in]
              }
              frame "512-C410 SLAT" {
                n382 = local read "SLAT (512-C419)"() -> (w825:T4)
                n383 = call "RTS Standard Test Set Time.vi"("Error In"=w827, "Internal Moisture Test (511-B111) - 5 Days"=w825) -> ("Error Out"=w826:errorcluster, "Output"=w828:T4)  [unwired: 8 in]
              }
              frame "511-B111 Internal Moisture" {
                # "This is a 5 day HUT"
                n384 = local read "Internal Moisture Test (511-B111) - 5 Days"() -> (w829:T4)
                n385 = call "RTS Standard Test Set Time.vi"("Error In"=w831, "Internal Moisture Test (511-B111) - 5 Days"=w829) -> ("Error Out"=w830:errorcluster, "Output"=w832:T4)  [unwired: 8 in]
              }
              frame "511-C401 Moisture Accumulation" {
                n386 = local read "Moisture Accumulation (511-C401)"() -> (w833:T4)
                n387 = call "RTS Standard Test Set Time.vi"("Error In"=w835, "Internal Moisture Test (511-B111) - 5 Days"=w833) -> ("Error Out"=w834:errorcluster, "Output"=w836:T4)  [unwired: 8 in]
              }
              frame "511-B100 No Door Opening (NDO)" {
                n388 = local read "NDO"() -> (w837:T4)
                n389 = call "RTS Standard Test Set Time.vi"("Error In"=w838, "Internal Moisture Test (511-B111) - 5 Days"=w837) -> ("Error Out"=w840:errorcluster, "Output"=w839:T4)  [unwired: 8 in]
              }
              frame "511-B304 ISO Energy Consumption" {
                n390 = local read "ISO Energy Consumption"() -> (w841:T4)
                n391 = call "RTS Standard Test Set Time.vi"("Error In"=w842, "Internal Moisture Test (511-B111) - 5 Days"=w841) -> ("Error Out"=w844:errorcluster, "Output"=w843:T4)  [unwired: 8 in]
              }
              frame "Custom Test" {
                n392 = local read "3-1"() -> (w846:T4)
              }
            }
            n393 = local write "3-1"(w806) -> ()
            n394 = Bundle By Name(cluster=w808, "3-1"=w806) -> (w807:T13)
          }
          event Value Change {
            n395 = event-data() -> ("NewVal"=w853:T8)  [unwired: 1 in, 5 out]
            n396 = case shown="\"Standard ETPs\", \"Cancel Test\", Default" w853 {
              selector: w853 -> [w854 _ _ _ _ _ _ _ _]
              tunnel: [w855 w861 w865 w869 w873 w877 w880 w884 w887] -> w847
              tunnel: w851 -> [w857 w860 w864 w868 w872 w876 w879 w882 w886]
              tunnel: [w857 w859 w863 w867 w871 w875 w881 w885 w886] -> w850
              frame "Standard ETPs", "Cancel Test", Default {
                n397 = Bundle By Name(cluster=T4 {"Chamber 1-3"=[], "Chamber 1-2"=[], "Chamber 1-1"=[], "Standard Tests 1-1"=enum."Standard ETPs"} ("1-1"), "Standard Tests 1-1"=w854) -> (w855:T4)
              }
              frame "511-B113 EHUT" {
                # "This is basically a 14 HUT"
                n398 = local read "EHUT (511-B113)"() -> (w858:T4)
                n399 = call "RTS Standard Test Set Time.vi"("Error In"=w860, "Internal Moisture Test (511-B111) - 5 Days"=w858) -> ("Error Out"=w859:errorcluster, "Output"=w861:T4)  [unwired: 8 in]
              }
              frame "511-B110 HUT" {
                # "24 Hr HUT"
                n400 = local read "HUT (511-B110)"() -> (w862:T4)
                n401 = call "RTS Standard Test Set Time.vi"("Error In"=w864, "Internal Moisture Test (511-B111) - 5 Days"=w862) -> ("Error Out"=w863:errorcluster, "Output"=w865:T4)  [unwired: 8 in]
              }
              frame "512-C410 SLAT" {
                n402 = local read "SLAT (512-C419)"() -> (w866:T4)
                n403 = call "RTS Standard Test Set Time.vi"("Error In"=w868, "Internal Moisture Test (511-B111) - 5 Days"=w866) -> ("Error Out"=w867:errorcluster, "Output"=w869:T4)  [unwired: 8 in]
              }
              frame "511-B111 Internal Moisture" {
                # "This is a 5 day HUT"
                n404 = local read "Internal Moisture Test (511-B111) - 5 Days"() -> (w870:T4)
                n405 = call "RTS Standard Test Set Time.vi"("Error In"=w872, "Internal Moisture Test (511-B111) - 5 Days"=w870) -> ("Error Out"=w871:errorcluster, "Output"=w873:T4)  [unwired: 8 in]
              }
              frame "511-C401 Moisture Accumulation" {
                n406 = local read "Moisture Accumulation (511-C401)"() -> (w874:T4)
                n407 = call "RTS Standard Test Set Time.vi"("Error In"=w876, "Internal Moisture Test (511-B111) - 5 Days"=w874) -> ("Error Out"=w875:errorcluster, "Output"=w877:T4)  [unwired: 8 in]
              }
              frame "511-B100 No Door Opening (NDO)" {
                n408 = local read "NDO"() -> (w878:T4)
                n409 = call "RTS Standard Test Set Time.vi"("Error In"=w879, "Internal Moisture Test (511-B111) - 5 Days"=w878) -> ("Error Out"=w881:errorcluster, "Output"=w880:T4)  [unwired: 8 in]
              }
              frame "511-B304 ISO Energy Consumption" {
                n410 = local read "ISO Energy Consumption"() -> (w883:T4)
                n411 = call "RTS Standard Test Set Time.vi"("Error In"=w882, "Internal Moisture Test (511-B111) - 5 Days"=w883) -> ("Error Out"=w885:errorcluster, "Output"=w884:T4)  [unwired: 8 in]
              }
              frame "Custom Test" {
                n412 = local read "3-2"() -> (w887:T4)
              }
            }
            n413 = local write "3-2"(w847) -> ()
            n414 = Bundle By Name(cluster=w849, "3-2"=w847) -> (w848:T13)
          }
          event Value Change {
            n415 = event-data() -> ("NewVal"=w894:T8)  [unwired: 1 in, 5 out]
            n416 = case shown="\"Standard ETPs\", \"Cancel Test\", Default" w894 {
              selector: w894 -> [w895 _ _ _ _ _ _ _ _]
              tunnel: [w896 w902 w906 w910 w914 w918 w920 w925 w928] -> w888
              tunnel: w892 -> [w898 w901 w905 w909 w913 w917 w921 w924 w927]
              tunnel: [w898 w900 w904 w908 w912 w916 w922 w926 w927] -> w891
              frame "Standard ETPs", "Cancel Test", Default {
                n417 = Bundle By Name(cluster=T4 {"Chamber 1-3"=[], "Chamber 1-2"=[], "Chamber 1-1"=[], "Standard Tests 1-1"=enum."Standard ETPs"} ("1-1"), "Standard Tests 1-1"=w895) -> (w896:T4)
              }
              frame "511-B113 EHUT" {
                # "This is basically a 14 HUT"
                n418 = local read "EHUT (511-B113)"() -> (w899:T4)
                n419 = call "RTS Standard Test Set Time.vi"("Error In"=w901, "Internal Moisture Test (511-B111) - 5 Days"=w899) -> ("Error Out"=w900:errorcluster, "Output"=w902:T4)  [unwired: 8 in]
              }
              frame "511-B110 HUT" {
                # "24 Hr HUT"
                n420 = local read "HUT (511-B110)"() -> (w903:T4)
                n421 = call "RTS Standard Test Set Time.vi"("Error In"=w905, "Internal Moisture Test (511-B111) - 5 Days"=w903) -> ("Error Out"=w904:errorcluster, "Output"=w906:T4)  [unwired: 8 in]
              }
              frame "512-C410 SLAT" {
                n422 = local read "SLAT (512-C419)"() -> (w907:T4)
                n423 = call "RTS Standard Test Set Time.vi"("Error In"=w909, "Internal Moisture Test (511-B111) - 5 Days"=w907) -> ("Error Out"=w908:errorcluster, "Output"=w910:T4)  [unwired: 8 in]
              }
              frame "511-B111 Internal Moisture" {
                # "This is a 5 day HUT"
                n424 = local read "Internal Moisture Test (511-B111) - 5 Days"() -> (w911:T4)
                n425 = call "RTS Standard Test Set Time.vi"("Error In"=w913, "Internal Moisture Test (511-B111) - 5 Days"=w911) -> ("Error Out"=w912:errorcluster, "Output"=w914:T4)  [unwired: 8 in]
              }
              frame "511-C401 Moisture Accumulation" {
                n426 = local read "Moisture Accumulation (511-C401)"() -> (w915:T4)
                n427 = call "RTS Standard Test Set Time.vi"("Error In"=w917, "Internal Moisture Test (511-B111) - 5 Days"=w915) -> ("Error Out"=w916:errorcluster, "Output"=w918:T4)  [unwired: 8 in]
              }
              frame "511-B100 No Door Opening (NDO)" {
                n428 = local read "NDO"() -> (w919:T4)
                n429 = call "RTS Standard Test Set Time.vi"("Error In"=w921, "Internal Moisture Test (511-B111) - 5 Days"=w919) -> ("Error Out"=w922:errorcluster, "Output"=w920:T4)  [unwired: 8 in]
              }
              frame "511-B304 ISO Energy Consumption" {
                n430 = local read "ISO Energy Consumption"() -> (w923:T4)
                n431 = call "RTS Standard Test Set Time.vi"("Error In"=w924, "Internal Moisture Test (511-B111) - 5 Days"=w923) -> ("Error Out"=w926:errorcluster, "Output"=w925:T4)  [unwired: 8 in]
              }
              frame "Custom Test" {
                n432 = local read "3-3"() -> (w928:T4)
              }
            }
            n433 = local write "3-3"(w888) -> ()
            n434 = Bundle By Name(cluster=w890, "3-3"=w888) -> (w889:T13)
          }
          event Value Change {
            n435 = event-data() -> ("NewVal"=w935:T8)  [unwired: 1 in, 5 out]
            n436 = case shown="\"Standard ETPs\", \"Cancel Test\", Default" w935 {
              selector: w935 -> [w936 _ _ _ _ _ _ _ _]
              tunnel: [w937 w943 w947 w951 w955 w959 w961 w967 w969] -> w929
              tunnel: w933 -> [w939 w942 w946 w950 w954 w958 w962 w965 w968]
              tunnel: [w939 w941 w945 w949 w953 w957 w963 w966 w968] -> w932
              frame "Standard ETPs", "Cancel Test", Default {
                n437 = Bundle By Name(cluster=T4 {"Chamber 1-3"=[], "Chamber 1-2"=[], "Chamber 1-1"=[], "Standard Tests 1-1"=enum."Standard ETPs"} ("1-1"), "Standard Tests 1-1"=w936) -> (w937:T4)
              }
              frame "511-B113 EHUT" {
                # "This is basically a 14 HUT"
                n438 = local read "EHUT (511-B113)"() -> (w940:T4)
                n439 = call "RTS Standard Test Set Time.vi"("Error In"=w942, "Internal Moisture Test (511-B111) - 5 Days"=w940) -> ("Error Out"=w941:errorcluster, "Output"=w943:T4)  [unwired: 8 in]
              }
              frame "511-B110 HUT" {
                # "24 Hr HUT"
                n440 = local read "HUT (511-B110)"() -> (w944:T4)
                n441 = call "RTS Standard Test Set Time.vi"("Error In"=w946, "Internal Moisture Test (511-B111) - 5 Days"=w944) -> ("Error Out"=w945:errorcluster, "Output"=w947:T4)  [unwired: 8 in]
              }
              frame "512-C410 SLAT" {
                n442 = local read "SLAT (512-C419)"() -> (w948:T4)
                n443 = call "RTS Standard Test Set Time.vi"("Error In"=w950, "Internal Moisture Test (511-B111) - 5 Days"=w948) -> ("Error Out"=w949:errorcluster, "Output"=w951:T4)  [unwired: 8 in]
              }
              frame "511-B111 Internal Moisture" {
                # "This is a 5 day HUT"
                n444 = local read "Internal Moisture Test (511-B111) - 5 Days"() -> (w952:T4)
                n445 = call "RTS Standard Test Set Time.vi"("Error In"=w954, "Internal Moisture Test (511-B111) - 5 Days"=w952) -> ("Error Out"=w953:errorcluster, "Output"=w955:T4)  [unwired: 8 in]
              }
              frame "511-C401 Moisture Accumulation" {
                n446 = local read "Moisture Accumulation (511-C401)"() -> (w956:T4)
                n447 = call "RTS Standard Test Set Time.vi"("Error In"=w958, "Internal Moisture Test (511-B111) - 5 Days"=w956) -> ("Error Out"=w957:errorcluster, "Output"=w959:T4)  [unwired: 8 in]
              }
              frame "511-B100 No Door Opening (NDO)" {
                n448 = local read "NDO"() -> (w960:T4)
                n449 = call "RTS Standard Test Set Time.vi"("Error In"=w962, "Internal Moisture Test (511-B111) - 5 Days"=w960) -> ("Error Out"=w963:errorcluster, "Output"=w961:T4)  [unwired: 8 in]
              }
              frame "511-B304 ISO Energy Consumption" {
                n450 = local read "ISO Energy Consumption"() -> (w964:T4)
                n451 = call "RTS Standard Test Set Time.vi"("Error In"=w965, "Internal Moisture Test (511-B111) - 5 Days"=w964) -> ("Error Out"=w966:errorcluster, "Output"=w967:T4)  [unwired: 8 in]
              }
              frame "Custom Test" {
                n452 = local read "3-4"() -> (w969:T4)
              }
            }
            n453 = local write "3-4"(w929) -> ()
            n454 = Bundle By Name(cluster=w931, "3-4"=w929) -> (w930:T13)
          }
          event Value Change {
            n455 = event-data() -> ("NewVal"=w976:T8)  [unwired: 1 in, 5 out]
            n456 = case shown="\"Standard ETPs\", \"Cancel Test\", Default" w976 {
              selector: w976 -> [w977 _ _ _ _ _ _ _ _]
              tunnel: [w978 w984 w988 w992 w996 w1000 w1003 w1008 w1010] -> w970
              tunnel: w974 -> [w980 w983 w987 w991 w995 w999 w1002 w1006 w1009]
              tunnel: [w980 w982 w986 w990 w994 w998 w1004 w1007 w1009] -> w973
              frame "Standard ETPs", "Cancel Test", Default {
                n457 = Bundle By Name(cluster=T4 {"Chamber 1-3"=[], "Chamber 1-2"=[], "Chamber 1-1"=[], "Standard Tests 1-1"=enum."Standard ETPs"} ("1-1"), "Standard Tests 1-1"=w977) -> (w978:T4)
              }
              frame "511-B113 EHUT" {
                # "This is basically a 14 HUT"
                n458 = local read "EHUT (511-B113)"() -> (w981:T4)
                n459 = call "RTS Standard Test Set Time.vi"("Error In"=w983, "Internal Moisture Test (511-B111) - 5 Days"=w981) -> ("Error Out"=w982:errorcluster, "Output"=w984:T4)  [unwired: 8 in]
              }
              frame "511-B110 HUT" {
                # "24 Hr HUT"
                n460 = local read "HUT (511-B110)"() -> (w985:T4)
                n461 = call "RTS Standard Test Set Time.vi"("Error In"=w987, "Internal Moisture Test (511-B111) - 5 Days"=w985) -> ("Error Out"=w986:errorcluster, "Output"=w988:T4)  [unwired: 8 in]
              }
              frame "512-C410 SLAT" {
                n462 = local read "SLAT (512-C419)"() -> (w989:T4)
                n463 = call "RTS Standard Test Set Time.vi"("Error In"=w991, "Internal Moisture Test (511-B111) - 5 Days"=w989) -> ("Error Out"=w990:errorcluster, "Output"=w992:T4)  [unwired: 8 in]
              }
              frame "511-B111 Internal Moisture" {
                # "This is a 5 day HUT"
                n464 = local read "Internal Moisture Test (511-B111) - 5 Days"() -> (w993:T4)
                n465 = call "RTS Standard Test Set Time.vi"("Error In"=w995, "Internal Moisture Test (511-B111) - 5 Days"=w993) -> ("Error Out"=w994:errorcluster, "Output"=w996:T4)  [unwired: 8 in]
              }
              frame "511-C401 Moisture Accumulation" {
                n466 = local read "Moisture Accumulation (511-C401)"() -> (w997:T4)
                n467 = call "RTS Standard Test Set Time.vi"("Error In"=w999, "Internal Moisture Test (511-B111) - 5 Days"=w997) -> ("Error Out"=w998:errorcluster, "Output"=w1000:T4)  [unwired: 8 in]
              }
              frame "511-B100 No Door Opening (NDO)" {
                n468 = local read "NDO"() -> (w1001:T4)
                n469 = call "RTS Standard Test Set Time.vi"("Error In"=w1002, "Internal Moisture Test (511-B111) - 5 Days"=w1001) -> ("Error Out"=w1004:errorcluster, "Output"=w1003:T4)  [unwired: 8 in]
              }
              frame "511-B304 ISO Energy Consumption" {
                n470 = local read "ISO Energy Consumption"() -> (w1005:T4)
                n471 = call "RTS Standard Test Set Time.vi"("Error In"=w1006, "Internal Moisture Test (511-B111) - 5 Days"=w1005) -> ("Error Out"=w1007:errorcluster, "Output"=w1008:T4)  [unwired: 8 in]
              }
              frame "Custom Test" {
                n472 = local read "3-5"() -> (w1010:T4)
              }
            }
            n473 = local write "3-5"(w970) -> ()
            n474 = Bundle By Name(cluster=w972, "3-5"=w970) -> (w971:T13)
          }
          event Value Change {
            n475 = event-data() -> ("NewVal"=w1017:T8)  [unwired: 1 in, 5 out]
            n476 = case shown="\"Standard ETPs\", \"Cancel Test\", Default" w1017 {
              selector: w1017 -> [w1018 _ _ _ _ _ _ _ _]
              tunnel: [w1019 w1025 w1029 w1033 w1037 w1041 w1044 w1048 w1051] -> w1011
              tunnel: w1015 -> [w1021 w1024 w1028 w1032 w1036 w1040 w1042 w1047 w1050]
              tunnel: [w1021 w1023 w1027 w1031 w1035 w1039 w1045 w1049 w1050] -> w1014
              frame "Standard ETPs", "Cancel Test", Default {
                n477 = Bundle By Name(cluster=T4 {"Chamber 1-3"=[], "Chamber 1-2"=[], "Chamber 1-1"=[], "Standard Tests 1-1"=enum."Standard ETPs"} ("1-1"), "Standard Tests 1-1"=w1018) -> (w1019:T4)
              }
              frame "511-B113 EHUT" {
                # "This is basically a 14 HUT"
                n478 = local read "EHUT (511-B113)"() -> (w1022:T4)
                n479 = call "RTS Standard Test Set Time.vi"("Error In"=w1024, "Internal Moisture Test (511-B111) - 5 Days"=w1022) -> ("Error Out"=w1023:errorcluster, "Output"=w1025:T4)  [unwired: 8 in]
              }
              frame "511-B110 HUT" {
                # "24 Hr HUT"
                n480 = local read "HUT (511-B110)"() -> (w1026:T4)
                n481 = call "RTS Standard Test Set Time.vi"("Error In"=w1028, "Internal Moisture Test (511-B111) - 5 Days"=w1026) -> ("Error Out"=w1027:errorcluster, "Output"=w1029:T4)  [unwired: 8 in]
              }
              frame "512-C410 SLAT" {
                n482 = local read "SLAT (512-C419)"() -> (w1030:T4)
                n483 = call "RTS Standard Test Set Time.vi"("Error In"=w1032, "Internal Moisture Test (511-B111) - 5 Days"=w1030) -> ("Error Out"=w1031:errorcluster, "Output"=w1033:T4)  [unwired: 8 in]
              }
              frame "511-B111 Internal Moisture" {
                # "This is a 5 day HUT"
                n484 = local read "Internal Moisture Test (511-B111) - 5 Days"() -> (w1034:T4)
                n485 = call "RTS Standard Test Set Time.vi"("Error In"=w1036, "Internal Moisture Test (511-B111) - 5 Days"=w1034) -> ("Error Out"=w1035:errorcluster, "Output"=w1037:T4)  [unwired: 8 in]
              }
              frame "511-C401 Moisture Accumulation" {
                n486 = local read "Moisture Accumulation (511-C401)"() -> (w1038:T4)
                n487 = call "RTS Standard Test Set Time.vi"("Error In"=w1040, "Internal Moisture Test (511-B111) - 5 Days"=w1038) -> ("Error Out"=w1039:errorcluster, "Output"=w1041:T4)  [unwired: 8 in]
              }
              frame "511-B100 No Door Opening (NDO)" {
                n488 = local read "NDO"() -> (w1043:T4)
                n489 = call "RTS Standard Test Set Time.vi"("Error In"=w1042, "Internal Moisture Test (511-B111) - 5 Days"=w1043) -> ("Error Out"=w1045:errorcluster, "Output"=w1044:T4)  [unwired: 8 in]
              }
              frame "511-B304 ISO Energy Consumption" {
                n490 = local read "ISO Energy Consumption"() -> (w1046:T4)
                n491 = call "RTS Standard Test Set Time.vi"("Error In"=w1047, "Internal Moisture Test (511-B111) - 5 Days"=w1046) -> ("Error Out"=w1049:errorcluster, "Output"=w1048:T4)  [unwired: 8 in]
              }
              frame "Custom Test" {
                n492 = local read "3-6"() -> (w1051:T4)
              }
            }
            n493 = local write "3-6"(w1011) -> ()
            n494 = Bundle By Name(cluster=w1013, "3-6"=w1011) -> (w1012:T13)
          }
          event Value Change {
            n495 = event-data() -> ("NewVal"=w1058:T8)  [unwired: 1 in, 5 out]
            n496 = case shown="\"Standard ETPs\", \"Cancel Test\", Default" w1058 {
              selector: w1058 -> [w1059 _ _ _ _ _ _ _ _]
              tunnel: [w1060 w1066 w1070 w1074 w1078 w1082 w1084 w1089 w1092] -> w1052
              tunnel: w1056 -> [w1062 w1065 w1069 w1073 w1077 w1081 w1086 w1088 w1091]
              tunnel: [w1062 w1064 w1068 w1072 w1076 w1080 w1085 w1090 w1091] -> w1055
              frame "Standard ETPs", "Cancel Test", Default {
                n497 = Bundle By Name(cluster=T4 {"Chamber 1-3"=[], "Chamber 1-2"=[], "Chamber 1-1"=[], "Standard Tests 1-1"=enum."Standard ETPs"} ("1-1"), "Standard Tests 1-1"=w1059) -> (w1060:T4)
              }
              frame "511-B113 EHUT" {
                # "This is basically a 14 HUT"
                n498 = local read "EHUT (511-B113)"() -> (w1063:T4)
                n499 = call "RTS Standard Test Set Time.vi"("Error In"=w1065, "Internal Moisture Test (511-B111) - 5 Days"=w1063) -> ("Error Out"=w1064:errorcluster, "Output"=w1066:T4)  [unwired: 8 in]
              }
              frame "511-B110 HUT" {
                # "24 Hr HUT"
                n500 = local read "HUT (511-B110)"() -> (w1067:T4)
                n501 = call "RTS Standard Test Set Time.vi"("Error In"=w1069, "Internal Moisture Test (511-B111) - 5 Days"=w1067) -> ("Error Out"=w1068:errorcluster, "Output"=w1070:T4)  [unwired: 8 in]
              }
              frame "512-C410 SLAT" {
                n502 = local read "SLAT (512-C419)"() -> (w1071:T4)
                n503 = call "RTS Standard Test Set Time.vi"("Error In"=w1073, "Internal Moisture Test (511-B111) - 5 Days"=w1071) -> ("Error Out"=w1072:errorcluster, "Output"=w1074:T4)  [unwired: 8 in]
              }
              frame "511-B111 Internal Moisture" {
                # "This is a 5 day HUT"
                n504 = local read "Internal Moisture Test (511-B111) - 5 Days"() -> (w1075:T4)
                n505 = call "RTS Standard Test Set Time.vi"("Error In"=w1077, "Internal Moisture Test (511-B111) - 5 Days"=w1075) -> ("Error Out"=w1076:errorcluster, "Output"=w1078:T4)  [unwired: 8 in]
              }
              frame "511-C401 Moisture Accumulation" {
                n506 = local read "Moisture Accumulation (511-C401)"() -> (w1079:T4)
                n507 = call "RTS Standard Test Set Time.vi"("Error In"=w1081, "Internal Moisture Test (511-B111) - 5 Days"=w1079) -> ("Error Out"=w1080:errorcluster, "Output"=w1082:T4)  [unwired: 8 in]
              }
              frame "511-B100 No Door Opening (NDO)" {
                n508 = local read "NDO"() -> (w1083:T4)
                n509 = call "RTS Standard Test Set Time.vi"("Error In"=w1086, "Internal Moisture Test (511-B111) - 5 Days"=w1083) -> ("Error Out"=w1085:errorcluster, "Output"=w1084:T4)  [unwired: 8 in]
              }
              frame "511-B304 ISO Energy Consumption" {
                n510 = local read "ISO Energy Consumption"() -> (w1087:T4)
                n511 = call "RTS Standard Test Set Time.vi"("Error In"=w1088, "Internal Moisture Test (511-B111) - 5 Days"=w1087) -> ("Error Out"=w1090:errorcluster, "Output"=w1089:T4)  [unwired: 8 in]
              }
              frame "Custom Test" {
                n512 = local read "3-7"() -> (w1092:T4)
              }
            }
            n513 = local write "3-7"(w1052) -> ()
            n514 = Bundle By Name(cluster=w1054, "3-7"=w1052) -> (w1053:T13)
          }
          event Value Change {
            n515 = event-data() -> ("NewVal"=w1099:T8)  [unwired: 1 in, 5 out]
            n516 = case shown="\"Standard ETPs\", \"Cancel Test\", Default" w1099 {
              selector: w1099 -> [w1100 _ _ _ _ _ _ _ _]
              tunnel: [w1101 w1107 w1111 w1115 w1119 w1123 w1126 w1130 w1133] -> w1093
              tunnel: w1097 -> [w1103 w1106 w1110 w1114 w1118 w1122 w1125 w1128 w1132]
              tunnel: [w1103 w1105 w1109 w1113 w1117 w1121 w1127 w1131 w1132] -> w1096
              frame "Standard ETPs", "Cancel Test", Default {
                n517 = Bundle By Name(cluster=T4 {"Chamber 1-3"=[], "Chamber 1-2"=[], "Chamber 1-1"=[], "Standard Tests 1-1"=enum."Standard ETPs"} ("1-1"), "Standard Tests 1-1"=w1100) -> (w1101:T4)
              }
              frame "511-B113 EHUT" {
                # "This is basically a 14 HUT"
                n518 = local read "EHUT (511-B113)"() -> (w1104:T4)
                n519 = call "RTS Standard Test Set Time.vi"("Error In"=w1106, "Internal Moisture Test (511-B111) - 5 Days"=w1104) -> ("Error Out"=w1105:errorcluster, "Output"=w1107:T4)  [unwired: 8 in]
              }
              frame "511-B110 HUT" {
                # "24 Hr HUT"
                n520 = local read "HUT (511-B110)"() -> (w1108:T4)
                n521 = call "RTS Standard Test Set Time.vi"("Error In"=w1110, "Internal Moisture Test (511-B111) - 5 Days"=w1108) -> ("Error Out"=w1109:errorcluster, "Output"=w1111:T4)  [unwired: 8 in]
              }
              frame "512-C410 SLAT" {
                n522 = local read "SLAT (512-C419)"() -> (w1112:T4)
                n523 = call "RTS Standard Test Set Time.vi"("Error In"=w1114, "Internal Moisture Test (511-B111) - 5 Days"=w1112) -> ("Error Out"=w1113:errorcluster, "Output"=w1115:T4)  [unwired: 8 in]
              }
              frame "511-B111 Internal Moisture" {
                # "This is a 5 day HUT"
                n524 = local read "Internal Moisture Test (511-B111) - 5 Days"() -> (w1116:T4)
                n525 = call "RTS Standard Test Set Time.vi"("Error In"=w1118, "Internal Moisture Test (511-B111) - 5 Days"=w1116) -> ("Error Out"=w1117:errorcluster, "Output"=w1119:T4)  [unwired: 8 in]
              }
              frame "511-C401 Moisture Accumulation" {
                n526 = local read "Moisture Accumulation (511-C401)"() -> (w1120:T4)
                n527 = call "RTS Standard Test Set Time.vi"("Error In"=w1122, "Internal Moisture Test (511-B111) - 5 Days"=w1120) -> ("Error Out"=w1121:errorcluster, "Output"=w1123:T4)  [unwired: 8 in]
              }
              frame "511-B100 No Door Opening (NDO)" {
                n528 = local read "NDO"() -> (w1124:T4)
                n529 = call "RTS Standard Test Set Time.vi"("Error In"=w1125, "Internal Moisture Test (511-B111) - 5 Days"=w1124) -> ("Error Out"=w1127:errorcluster, "Output"=w1126:T4)  [unwired: 8 in]
              }
              frame "511-B304 ISO Energy Consumption" {
                n530 = local read "ISO Energy Consumption"() -> (w1129:T4)
                n531 = call "RTS Standard Test Set Time.vi"("Error In"=w1128, "Internal Moisture Test (511-B111) - 5 Days"=w1129) -> ("Error Out"=w1131:errorcluster, "Output"=w1130:T4)  [unwired: 8 in]
              }
              frame "Custom Test" {
                n532 = local read "3-8"() -> (w1133:T4)
              }
            }
            n533 = local write "3-8"(w1093) -> ()
            n534 = Bundle By Name(cluster=w1095, "3-8"=w1093) -> (w1094:T13)
          }
          event Value Change {
            n535 = event-data() -> ("NewVal"=w1140:T8)  [unwired: 1 in, 5 out]
            n536 = case shown="\"Standard ETPs\", \"Cancel Test\", Default" w1140 {
              selector: w1140 -> [w1141 _ _ _ _ _ _ _ _]
              tunnel: [w1142 w1148 w1152 w1156 w1160 w1164 w1166 w1171 w1174] -> w1134
              tunnel: w1139 -> [w1144 w1147 w1151 w1155 w1159 w1163 w1167 w1170 w1173]
              tunnel: [w1144 w1146 w1150 w1154 w1158 w1162 w1168 w1172 w1173] -> w1138
              frame "Standard ETPs", "Cancel Test", Default {
                n537 = Bundle By Name(cluster=T4 {"Chamber 1-3"=[], "Chamber 1-2"=[], "Chamber 1-1"=[], "Standard Tests 1-1"=enum."Standard ETPs"} ("1-1"), "Standard Tests 1-1"=w1141) -> (w1142:T4)
              }
              frame "511-B113 EHUT" {
                # "This is basically a 14 HUT"
                n538 = local read "EHUT (511-B113)"() -> (w1145:T4)
                n539 = call "RTS Standard Test Set Time.vi"("Error In"=w1147, "Internal Moisture Test (511-B111) - 5 Days"=w1145) -> ("Error Out"=w1146:errorcluster, "Output"=w1148:T4)  [unwired: 8 in]
              }
              frame "511-B110 HUT" {
                # "24 Hr HUT"
                n540 = local read "HUT (511-B110)"() -> (w1149:T4)
                n541 = call "RTS Standard Test Set Time.vi"("Error In"=w1151, "Internal Moisture Test (511-B111) - 5 Days"=w1149) -> ("Error Out"=w1150:errorcluster, "Output"=w1152:T4)  [unwired: 8 in]
              }
              frame "512-C410 SLAT" {
                n542 = local read "SLAT (512-C419)"() -> (w1153:T4)
                n543 = call "RTS Standard Test Set Time.vi"("Error In"=w1155, "Internal Moisture Test (511-B111) - 5 Days"=w1153) -> ("Error Out"=w1154:errorcluster, "Output"=w1156:T4)  [unwired: 8 in]
              }
              frame "511-B111 Internal Moisture" {
                # "This is a 5 day HUT"
                n544 = local read "Internal Moisture Test (511-B111) - 5 Days"() -> (w1157:T4)
                n545 = call "RTS Standard Test Set Time.vi"("Error In"=w1159, "Internal Moisture Test (511-B111) - 5 Days"=w1157) -> ("Error Out"=w1158:errorcluster, "Output"=w1160:T4)  [unwired: 8 in]
              }
              frame "511-C401 Moisture Accumulation" {
                n546 = local read "Moisture Accumulation (511-C401)"() -> (w1161:T4)
                n547 = call "RTS Standard Test Set Time.vi"("Error In"=w1163, "Internal Moisture Test (511-B111) - 5 Days"=w1161) -> ("Error Out"=w1162:errorcluster, "Output"=w1164:T4)  [unwired: 8 in]
              }
              frame "511-B100 No Door Opening (NDO)" {
                n548 = local read "NDO"() -> (w1165:T4)
                n549 = call "RTS Standard Test Set Time.vi"("Error In"=w1167, "Internal Moisture Test (511-B111) - 5 Days"=w1165) -> ("Error Out"=w1168:errorcluster, "Output"=w1166:T4)  [unwired: 8 in]
              }
              frame "511-B304 ISO Energy Consumption" {
                n550 = local read "ISO Energy Consumption"() -> (w1169:T4)
                n551 = call "RTS Standard Test Set Time.vi"("Error In"=w1170, "Internal Moisture Test (511-B111) - 5 Days"=w1169) -> ("Error Out"=w1172:errorcluster, "Output"=w1171:T4)  [unwired: 8 in]
              }
              frame "Custom Test" {
                n552 = local read "4-1"() -> (w1174:T4)
              }
            }
            n553 = local write "4-1"(w1134) -> ()
            n554 = Bundle By Name(cluster=w1136, "4-1"=w1134) -> (w1135:T13)
          }
          event Value Change {
            n555 = event-data() -> ("NewVal"=w1181:T8)  [unwired: 1 in, 5 out]
            n556 = case shown="\"Standard ETPs\", \"Cancel Test\", Default" w1181 {
              selector: w1181 -> [w1182 _ _ _ _ _ _ _ _]
              tunnel: [w1183 w1189 w1193 w1197 w1201 w1205 w1208 w1211 w1214] -> w1175
              tunnel: w1179 -> [w1185 w1188 w1192 w1196 w1200 w1204 w1207 w1212 w1215]
              tunnel: [w1185 w1187 w1191 w1195 w1199 w1203 w1209 w1213 w1215] -> w1178
              frame "Standard ETPs", "Cancel Test", Default {
                n557 = Bundle By Name(cluster=T4 {"Chamber 1-3"=[], "Chamber 1-2"=[], "Chamber 1-1"=[], "Standard Tests 1-1"=enum."Standard ETPs"} ("1-1"), "Standard Tests 1-1"=w1182) -> (w1183:T4)
              }
              frame "511-B113 EHUT" {
                # "This is basically a 14 HUT"
                n558 = local read "EHUT (511-B113)"() -> (w1186:T4)
                n559 = call "RTS Standard Test Set Time.vi"("Error In"=w1188, "Internal Moisture Test (511-B111) - 5 Days"=w1186) -> ("Error Out"=w1187:errorcluster, "Output"=w1189:T4)  [unwired: 8 in]
              }
              frame "511-B110 HUT" {
                # "24 Hr HUT"
                n560 = local read "HUT (511-B110)"() -> (w1190:T4)
                n561 = call "RTS Standard Test Set Time.vi"("Error In"=w1192, "Internal Moisture Test (511-B111) - 5 Days"=w1190) -> ("Error Out"=w1191:errorcluster, "Output"=w1193:T4)  [unwired: 8 in]
              }
              frame "512-C410 SLAT" {
                n562 = local read "SLAT (512-C419)"() -> (w1194:T4)
                n563 = call "RTS Standard Test Set Time.vi"("Error In"=w1196, "Internal Moisture Test (511-B111) - 5 Days"=w1194) -> ("Error Out"=w1195:errorcluster, "Output"=w1197:T4)  [unwired: 8 in]
              }
              frame "511-B111 Internal Moisture" {
                # "This is a 5 day HUT"
                n564 = local read "Internal Moisture Test (511-B111) - 5 Days"() -> (w1198:T4)
                n565 = call "RTS Standard Test Set Time.vi"("Error In"=w1200, "Internal Moisture Test (511-B111) - 5 Days"=w1198) -> ("Error Out"=w1199:errorcluster, "Output"=w1201:T4)  [unwired: 8 in]
              }
              frame "511-C401 Moisture Accumulation" {
                n566 = local read "Moisture Accumulation (511-C401)"() -> (w1202:T4)
                n567 = call "RTS Standard Test Set Time.vi"("Error In"=w1204, "Internal Moisture Test (511-B111) - 5 Days"=w1202) -> ("Error Out"=w1203:errorcluster, "Output"=w1205:T4)  [unwired: 8 in]
              }
              frame "511-B100 No Door Opening (NDO)" {
                n568 = local read "NDO"() -> (w1206:T4)
                n569 = call "RTS Standard Test Set Time.vi"("Error In"=w1207, "Internal Moisture Test (511-B111) - 5 Days"=w1206) -> ("Error Out"=w1209:errorcluster, "Output"=w1208:T4)  [unwired: 8 in]
              }
              frame "511-B304 ISO Energy Consumption" {
                n570 = local read "ISO Energy Consumption"() -> (w1210:T4)
                n571 = call "RTS Standard Test Set Time.vi"("Error In"=w1212, "Internal Moisture Test (511-B111) - 5 Days"=w1210) -> ("Error Out"=w1213:errorcluster, "Output"=w1211:T4)  [unwired: 8 in]
              }
              frame "Custom Test" {
                n572 = local read "4-2"() -> (w1214:T4)
              }
            }
            n573 = local write "4-2"(w1175) -> ()
            n574 = Bundle By Name(cluster=w1177, "4-2"=w1175) -> (w1176:T13)
          }
          event Value Change {
            n575 = event-data() -> ("NewVal"=w1222:T8)  [unwired: 1 in, 5 out]
            n576 = case shown="\"Standard ETPs\", \"Cancel Test\", Default" w1222 {
              selector: w1222 -> [w1223 _ _ _ _ _ _ _ _]
              tunnel: [w1224 w1230 w1234 w1238 w1242 w1246 w1249 w1252 w1256] -> w1216
              tunnel: w1221 -> [w1226 w1229 w1233 w1237 w1241 w1245 w1248 w1253 w1255]
              tunnel: [w1226 w1228 w1232 w1236 w1240 w1244 w1250 w1254 w1255] -> w1220
              frame "Standard ETPs", "Cancel Test", Default {
                n577 = Bundle By Name(cluster=T4 {"Chamber 1-3"=[], "Chamber 1-2"=[], "Chamber 1-1"=[], "Standard Tests 1-1"=enum."Standard ETPs"} ("1-1"), "Standard Tests 1-1"=w1223) -> (w1224:T4)
              }
              frame "511-B113 EHUT" {
                # "This is basically a 14 HUT"
                n578 = local read "EHUT (511-B113)"() -> (w1227:T4)
                n579 = call "RTS Standard Test Set Time.vi"("Error In"=w1229, "Internal Moisture Test (511-B111) - 5 Days"=w1227) -> ("Error Out"=w1228:errorcluster, "Output"=w1230:T4)  [unwired: 8 in]
              }
              frame "511-B110 HUT" {
                # "24 Hr HUT"
                n580 = local read "HUT (511-B110)"() -> (w1231:T4)
                n581 = call "RTS Standard Test Set Time.vi"("Error In"=w1233, "Internal Moisture Test (511-B111) - 5 Days"=w1231) -> ("Error Out"=w1232:errorcluster, "Output"=w1234:T4)  [unwired: 8 in]
              }
              frame "512-C410 SLAT" {
                n582 = local read "SLAT (512-C419)"() -> (w1235:T4)
                n583 = call "RTS Standard Test Set Time.vi"("Error In"=w1237, "Internal Moisture Test (511-B111) - 5 Days"=w1235) -> ("Error Out"=w1236:errorcluster, "Output"=w1238:T4)  [unwired: 8 in]
              }
              frame "511-B111 Internal Moisture" {
                # "This is a 5 day HUT"
                n584 = local read "Internal Moisture Test (511-B111) - 5 Days"() -> (w1239:T4)
                n585 = call "RTS Standard Test Set Time.vi"("Error In"=w1241, "Internal Moisture Test (511-B111) - 5 Days"=w1239) -> ("Error Out"=w1240:errorcluster, "Output"=w1242:T4)  [unwired: 8 in]
              }
              frame "511-C401 Moisture Accumulation" {
                n586 = local read "Moisture Accumulation (511-C401)"() -> (w1243:T4)
                n587 = call "RTS Standard Test Set Time.vi"("Error In"=w1245, "Internal Moisture Test (511-B111) - 5 Days"=w1243) -> ("Error Out"=w1244:errorcluster, "Output"=w1246:T4)  [unwired: 8 in]
              }
              frame "511-B100 No Door Opening (NDO)" {
                n588 = local read "NDO"() -> (w1247:T4)
                n589 = call "RTS Standard Test Set Time.vi"("Error In"=w1248, "Internal Moisture Test (511-B111) - 5 Days"=w1247) -> ("Error Out"=w1250:errorcluster, "Output"=w1249:T4)  [unwired: 8 in]
              }
              frame "511-B304 ISO Energy Consumption" {
                n590 = local read "ISO Energy Consumption"() -> (w1251:T4)
                n591 = call "RTS Standard Test Set Time.vi"("Error In"=w1253, "Internal Moisture Test (511-B111) - 5 Days"=w1251) -> ("Error Out"=w1254:errorcluster, "Output"=w1252:T4)  [unwired: 8 in]
              }
              frame "Custom Test" {
                n592 = local read "4-3"() -> (w1256:T4)
              }
            }
            n593 = local write "4-3"(w1216) -> ()
            n594 = Bundle By Name(cluster=w1218, "4-3"=w1216) -> (w1217:T13)
          }
          event Value Change {
            n595 = event-data() -> ("NewVal"=w1263:T8)  [unwired: 1 in, 5 out]
            n596 = case shown="\"Standard ETPs\", \"Cancel Test\", Default" w1263 {
              selector: w1263 -> [w1264 _ _ _ _ _ _ _ _]
              tunnel: [w1265 w1271 w1275 w1279 w1283 w1287 w1290 w1294 w1297] -> w1257
              tunnel: w1261 -> [w1267 w1270 w1274 w1278 w1282 w1286 w1288 w1293 w1296]
              tunnel: [w1267 w1269 w1273 w1277 w1281 w1285 w1291 w1295 w1296] -> w1260
              frame "Standard ETPs", "Cancel Test", Default {
                n597 = Bundle By Name(cluster=T4 {"Chamber 1-3"=[], "Chamber 1-2"=[], "Chamber 1-1"=[], "Standard Tests 1-1"=enum."Standard ETPs"} ("1-1"), "Standard Tests 1-1"=w1264) -> (w1265:T4)
              }
              frame "511-B113 EHUT" {
                # "This is basically a 14 HUT"
                n598 = local read "EHUT (511-B113)"() -> (w1268:T4)
                n599 = call "RTS Standard Test Set Time.vi"("Error In"=w1270, "Internal Moisture Test (511-B111) - 5 Days"=w1268) -> ("Error Out"=w1269:errorcluster, "Output"=w1271:T4)  [unwired: 8 in]
              }
              frame "511-B110 HUT" {
                # "24 Hr HUT"
                n600 = local read "HUT (511-B110)"() -> (w1272:T4)
                n601 = call "RTS Standard Test Set Time.vi"("Error In"=w1274, "Internal Moisture Test (511-B111) - 5 Days"=w1272) -> ("Error Out"=w1273:errorcluster, "Output"=w1275:T4)  [unwired: 8 in]
              }
              frame "512-C410 SLAT" {
                n602 = local read "SLAT (512-C419)"() -> (w1276:T4)
                n603 = call "RTS Standard Test Set Time.vi"("Error In"=w1278, "Internal Moisture Test (511-B111) - 5 Days"=w1276) -> ("Error Out"=w1277:errorcluster, "Output"=w1279:T4)  [unwired: 8 in]
              }
              frame "511-B111 Internal Moisture" {
                # "This is a 5 day HUT"
                n604 = local read "Internal Moisture Test (511-B111) - 5 Days"() -> (w1280:T4)
                n605 = call "RTS Standard Test Set Time.vi"("Error In"=w1282, "Internal Moisture Test (511-B111) - 5 Days"=w1280) -> ("Error Out"=w1281:errorcluster, "Output"=w1283:T4)  [unwired: 8 in]
              }
              frame "511-C401 Moisture Accumulation" {
                n606 = local read "Moisture Accumulation (511-C401)"() -> (w1284:T4)
                n607 = call "RTS Standard Test Set Time.vi"("Error In"=w1286, "Internal Moisture Test (511-B111) - 5 Days"=w1284) -> ("Error Out"=w1285:errorcluster, "Output"=w1287:T4)  [unwired: 8 in]
              }
              frame "511-B100 No Door Opening (NDO)" {
                n608 = local read "NDO"() -> (w1289:T4)
                n609 = call "RTS Standard Test Set Time.vi"("Error In"=w1288, "Internal Moisture Test (511-B111) - 5 Days"=w1289) -> ("Error Out"=w1291:errorcluster, "Output"=w1290:T4)  [unwired: 8 in]
              }
              frame "511-B304 ISO Energy Consumption" {
                n610 = local read "ISO Energy Consumption"() -> (w1292:T4)
                n611 = call "RTS Standard Test Set Time.vi"("Error In"=w1293, "Internal Moisture Test (511-B111) - 5 Days"=w1292) -> ("Error Out"=w1295:errorcluster, "Output"=w1294:T4)  [unwired: 8 in]
              }
              frame "Custom Test" {
                n612 = local read "4-4"() -> (w1297:T4)
              }
            }
            n613 = local write "4-4"(w1257) -> ()
            n614 = Bundle By Name(cluster=w1259, "4-4"=w1257) -> (w1258:T13)
          }
          event Value Change {
            n615 = event-data() -> ("NewVal"=w1304:T8)  [unwired: 1 in, 5 out]
            n616 = case shown="\"Standard ETPs\", \"Cancel Test\", Default" w1304 {
              selector: w1304 -> [w1307 _ _ _ _ _ _ _ _]
              tunnel: [w1305 w1312 w1316 w1320 w1324 w1328 w1330 w1334 w1338] -> w1298
              tunnel: w1302 -> [w1308 w1311 w1315 w1319 w1323 w1327 w1332 w1336 w1337]
              tunnel: [w1308 w1310 w1314 w1318 w1322 w1326 w1331 w1335 w1337] -> w1301
              frame "Standard ETPs", "Cancel Test", Default {
                n617 = Bundle By Name(cluster=T4 {"Chamber 1-3"=[], "Chamber 1-2"=[], "Chamber 1-1"=[], "Standard Tests 1-1"=enum."Standard ETPs"} ("1-1"), "Standard Tests 1-1"=w1307) -> (w1305:T4)
              }
              frame "511-B113 EHUT" {
                # "This is basically a 14 HUT"
                n618 = local read "EHUT (511-B113)"() -> (w1309:T4)
                n619 = call "RTS Standard Test Set Time.vi"("Error In"=w1311, "Internal Moisture Test (511-B111) - 5 Days"=w1309) -> ("Error Out"=w1310:errorcluster, "Output"=w1312:T4)  [unwired: 8 in]
              }
              frame "511-B110 HUT" {
                # "24 Hr HUT"
                n620 = local read "HUT (511-B110)"() -> (w1313:T4)
                n621 = call "RTS Standard Test Set Time.vi"("Error In"=w1315, "Internal Moisture Test (511-B111) - 5 Days"=w1313) -> ("Error Out"=w1314:errorcluster, "Output"=w1316:T4)  [unwired: 8 in]
              }
              frame "512-C410 SLAT" {
                n622 = local read "SLAT (512-C419)"() -> (w1317:T4)
                n623 = call "RTS Standard Test Set Time.vi"("Error In"=w1319, "Internal Moisture Test (511-B111) - 5 Days"=w1317) -> ("Error Out"=w1318:errorcluster, "Output"=w1320:T4)  [unwired: 8 in]
              }
              frame "511-B111 Internal Moisture" {
                # "This is a 5 day HUT"
                n624 = local read "Internal Moisture Test (511-B111) - 5 Days"() -> (w1321:T4)
                n625 = call "RTS Standard Test Set Time.vi"("Error In"=w1323, "Internal Moisture Test (511-B111) - 5 Days"=w1321) -> ("Error Out"=w1322:errorcluster, "Output"=w1324:T4)  [unwired: 8 in]
              }
              frame "511-C401 Moisture Accumulation" {
                n626 = local read "Moisture Accumulation (511-C401)"() -> (w1325:T4)
                n627 = call "RTS Standard Test Set Time.vi"("Error In"=w1327, "Internal Moisture Test (511-B111) - 5 Days"=w1325) -> ("Error Out"=w1326:errorcluster, "Output"=w1328:T4)  [unwired: 8 in]
              }
              frame "511-B100 No Door Opening (NDO)" {
                n628 = local read "NDO"() -> (w1329:T4)
                n629 = call "RTS Standard Test Set Time.vi"("Error In"=w1332, "Internal Moisture Test (511-B111) - 5 Days"=w1329) -> ("Error Out"=w1331:errorcluster, "Output"=w1330:T4)  [unwired: 8 in]
              }
              frame "511-B304 ISO Energy Consumption" {
                n630 = local read "ISO Energy Consumption"() -> (w1333:T4)
                n631 = call "RTS Standard Test Set Time.vi"("Error In"=w1336, "Internal Moisture Test (511-B111) - 5 Days"=w1333) -> ("Error Out"=w1335:errorcluster, "Output"=w1334:T4)  [unwired: 8 in]
              }
              frame "Custom Test" {
                n632 = local read "4-5"() -> (w1338:T4)
              }
            }
            n633 = local write "4-5"(w1298) -> ()
            n634 = Bundle By Name(cluster=w1300, "4-5"=w1298) -> (w1299:T13)
          }
          event Value Change {
            n635 = event-data() -> ("NewVal"=w1344:T8)  [unwired: 1 in, 5 out]
            n636 = case shown="\"Standard ETPs\", \"Cancel Test\", Default" w1344 {
              selector: w1344 -> [w1347 _ _ _ _ _ _ _ _]
              tunnel: [w1346 w1353 w1357 w1361 w1365 w1369 w1371 w1375 w1379] -> w1339
              tunnel: w1343 -> [w1349 w1352 w1356 w1360 w1364 w1368 w1372 w1376 w1378]
              tunnel: [w1349 w1351 w1355 w1359 w1363 w1367 w1373 w1377 w1378] -> w1342
              frame "Standard ETPs", "Cancel Test", Default {
                n637 = Bundle By Name(cluster=T4 {"Chamber 1-3"=[], "Chamber 1-2"=[], "Chamber 1-1"=[], "Standard Tests 1-1"=enum."Standard ETPs"} ("1-1"), "Standard Tests 1-1"=w1347) -> (w1346:T4)
              }
              frame "511-B113 EHUT" {
                # "This is basically a 14 HUT"
                n638 = local read "EHUT (511-B113)"() -> (w1350:T4)
                n639 = call "RTS Standard Test Set Time.vi"("Error In"=w1352, "Internal Moisture Test (511-B111) - 5 Days"=w1350) -> ("Error Out"=w1351:errorcluster, "Output"=w1353:T4)  [unwired: 8 in]
              }
              frame "511-B110 HUT" {
                # "24 Hr HUT"
                n640 = local read "HUT (511-B110)"() -> (w1354:T4)
                n641 = call "RTS Standard Test Set Time.vi"("Error In"=w1356, "Internal Moisture Test (511-B111) - 5 Days"=w1354) -> ("Error Out"=w1355:errorcluster, "Output"=w1357:T4)  [unwired: 8 in]
              }
              frame "512-C410 SLAT" {
                n642 = local read "SLAT (512-C419)"() -> (w1358:T4)
                n643 = call "RTS Standard Test Set Time.vi"("Error In"=w1360, "Internal Moisture Test (511-B111) - 5 Days"=w1358) -> ("Error Out"=w1359:errorcluster, "Output"=w1361:T4)  [unwired: 8 in]
              }
              frame "511-B111 Internal Moisture" {
                # "This is a 5 day HUT"
                n644 = local read "Internal Moisture Test (511-B111) - 5 Days"() -> (w1362:T4)
                n645 = call "RTS Standard Test Set Time.vi"("Error In"=w1364, "Internal Moisture Test (511-B111) - 5 Days"=w1362) -> ("Error Out"=w1363:errorcluster, "Output"=w1365:T4)  [unwired: 8 in]
              }
              frame "511-C401 Moisture Accumulation" {
                n646 = local read "Moisture Accumulation (511-C401)"() -> (w1366:T4)
                n647 = call "RTS Standard Test Set Time.vi"("Error In"=w1368, "Internal Moisture Test (511-B111) - 5 Days"=w1366) -> ("Error Out"=w1367:errorcluster, "Output"=w1369:T4)  [unwired: 8 in]
              }
              frame "511-B100 No Door Opening (NDO)" {
                n648 = local read "NDO"() -> (w1370:T4)
                n649 = call "RTS Standard Test Set Time.vi"("Error In"=w1372, "Internal Moisture Test (511-B111) - 5 Days"=w1370) -> ("Error Out"=w1373:errorcluster, "Output"=w1371:T4)  [unwired: 8 in]
              }
              frame "511-B304 ISO Energy Consumption" {
                n650 = local read "ISO Energy Consumption"() -> (w1374:T4)
                n651 = call "RTS Standard Test Set Time.vi"("Error In"=w1376, "Internal Moisture Test (511-B111) - 5 Days"=w1374) -> ("Error Out"=w1377:errorcluster, "Output"=w1375:T4)  [unwired: 8 in]
              }
              frame "Custom Test" {
                n652 = local read "4-6"() -> (w1379:T4)
              }
            }
            n653 = local write "4-6"(w1339) -> ()
            n654 = Bundle By Name(cluster=w1341, "4-6"=w1339) -> (w1340:T13)
          }
          event Value Change {
            n655 = event-data() -> ("NewVal"=w1386:T8)  [unwired: 1 in, 5 out]
            n656 = case shown="\"Standard ETPs\", \"Cancel Test\", Default" w1386 {
              selector: w1386 -> [w1387 _ _ _ _ _ _ _ _]
              tunnel: [w1388 w1394 w1398 w1402 w1406 w1410 w1413 w1417 w1420] -> w1380
              tunnel: w1384 -> [w1390 w1393 w1397 w1401 w1405 w1409 w1412 w1416 w1419]
              tunnel: [w1390 w1392 w1396 w1400 w1404 w1408 w1414 w1418 w1419] -> w1383
              frame "Standard ETPs", "Cancel Test", Default {
                n657 = Bundle By Name(cluster=T4 {"Chamber 1-3"=[], "Chamber 1-2"=[], "Chamber 1-1"=[], "Standard Tests 1-1"=enum."Standard ETPs"} ("1-1"), "Standard Tests 1-1"=w1387) -> (w1388:T4)
              }
              frame "511-B113 EHUT" {
                # "This is basically a 14 HUT"
                n658 = local read "EHUT (511-B113)"() -> (w1391:T4)
                n659 = call "RTS Standard Test Set Time.vi"("Error In"=w1393, "Internal Moisture Test (511-B111) - 5 Days"=w1391) -> ("Error Out"=w1392:errorcluster, "Output"=w1394:T4)  [unwired: 8 in]
              }
              frame "511-B110 HUT" {
                # "24 Hr HUT"
                n660 = local read "HUT (511-B110)"() -> (w1395:T4)
                n661 = call "RTS Standard Test Set Time.vi"("Error In"=w1397, "Internal Moisture Test (511-B111) - 5 Days"=w1395) -> ("Error Out"=w1396:errorcluster, "Output"=w1398:T4)  [unwired: 8 in]
              }
              frame "512-C410 SLAT" {
                n662 = local read "SLAT (512-C419)"() -> (w1399:T4)
                n663 = call "RTS Standard Test Set Time.vi"("Error In"=w1401, "Internal Moisture Test (511-B111) - 5 Days"=w1399) -> ("Error Out"=w1400:errorcluster, "Output"=w1402:T4)  [unwired: 8 in]
              }
              frame "511-B111 Internal Moisture" {
                # "This is a 5 day HUT"
                n664 = local read "Internal Moisture Test (511-B111) - 5 Days"() -> (w1403:T4)
                n665 = call "RTS Standard Test Set Time.vi"("Error In"=w1405, "Internal Moisture Test (511-B111) - 5 Days"=w1403) -> ("Error Out"=w1404:errorcluster, "Output"=w1406:T4)  [unwired: 8 in]
              }
              frame "511-C401 Moisture Accumulation" {
                n666 = local read "Moisture Accumulation (511-C401)"() -> (w1407:T4)
                n667 = call "RTS Standard Test Set Time.vi"("Error In"=w1409, "Internal Moisture Test (511-B111) - 5 Days"=w1407) -> ("Error Out"=w1408:errorcluster, "Output"=w1410:T4)  [unwired: 8 in]
              }
              frame "511-B100 No Door Opening (NDO)" {
                n668 = local read "NDO"() -> (w1411:T4)
                n669 = call "RTS Standard Test Set Time.vi"("Error In"=w1412, "Internal Moisture Test (511-B111) - 5 Days"=w1411) -> ("Error Out"=w1414:errorcluster, "Output"=w1413:T4)  [unwired: 8 in]
              }
              frame "511-B304 ISO Energy Consumption" {
                n670 = local read "ISO Energy Consumption"() -> (w1415:T4)
                n671 = call "RTS Standard Test Set Time.vi"("Error In"=w1416, "Internal Moisture Test (511-B111) - 5 Days"=w1415) -> ("Error Out"=w1418:errorcluster, "Output"=w1417:T4)  [unwired: 8 in]
              }
              frame "Custom Test" {
                n672 = local read "4-7"() -> (w1420:T4)
              }
            }
            n673 = Bundle By Name(cluster=w1382, "4-7"=w1380) -> (w1381:T13)
            n674 = local write "4-7"(w1380) -> ()
          }
          event Value Change {
            n675 = event-data() -> ("NewVal"=w1427:T8)  [unwired: 1 in, 5 out]
            n676 = case shown="\"Standard ETPs\", \"Cancel Test\", Default" w1427 {
              selector: w1427 -> [w1428 _ _ _ _ _ _ _ _]
              tunnel: [w1429 w1435 w1439 w1443 w1447 w1451 w1454 w1458 w1461] -> w1421
              tunnel: w1425 -> [w1431 w1434 w1438 w1442 w1446 w1450 w1453 w1457 w1460]
              tunnel: [w1431 w1433 w1437 w1441 w1445 w1449 w1455 w1459 w1460] -> w1424
              frame "Standard ETPs", "Cancel Test", Default {
                n677 = Bundle By Name(cluster=T4 {"Chamber 1-3"=[], "Chamber 1-2"=[], "Chamber 1-1"=[], "Standard Tests 1-1"=enum."Standard ETPs"} ("1-1"), "Standard Tests 1-1"=w1428) -> (w1429:T4)
              }
              frame "511-B113 EHUT" {
                # "This is basically a 14 HUT"
                n678 = local read "EHUT (511-B113)"() -> (w1432:T4)
                n679 = call "RTS Standard Test Set Time.vi"("Error In"=w1434, "Internal Moisture Test (511-B111) - 5 Days"=w1432) -> ("Error Out"=w1433:errorcluster, "Output"=w1435:T4)  [unwired: 8 in]
              }
              frame "511-B110 HUT" {
                # "24 Hr HUT"
                n680 = local read "HUT (511-B110)"() -> (w1436:T4)
                n681 = call "RTS Standard Test Set Time.vi"("Error In"=w1438, "Internal Moisture Test (511-B111) - 5 Days"=w1436) -> ("Error Out"=w1437:errorcluster, "Output"=w1439:T4)  [unwired: 8 in]
              }
              frame "512-C410 SLAT" {
                n682 = local read "SLAT (512-C419)"() -> (w1440:T4)
                n683 = call "RTS Standard Test Set Time.vi"("Error In"=w1442, "Internal Moisture Test (511-B111) - 5 Days"=w1440) -> ("Error Out"=w1441:errorcluster, "Output"=w1443:T4)  [unwired: 8 in]
              }
              frame "511-B111 Internal Moisture" {
                # "This is a 5 day HUT"
                n684 = local read "Internal Moisture Test (511-B111) - 5 Days"() -> (w1444:T4)
                n685 = call "RTS Standard Test Set Time.vi"("Error In"=w1446, "Internal Moisture Test (511-B111) - 5 Days"=w1444) -> ("Error Out"=w1445:errorcluster, "Output"=w1447:T4)  [unwired: 8 in]
              }
              frame "511-C401 Moisture Accumulation" {
                n686 = local read "Moisture Accumulation (511-C401)"() -> (w1448:T4)
                n687 = call "RTS Standard Test Set Time.vi"("Error In"=w1450, "Internal Moisture Test (511-B111) - 5 Days"=w1448) -> ("Error Out"=w1449:errorcluster, "Output"=w1451:T4)  [unwired: 8 in]
              }
              frame "511-B100 No Door Opening (NDO)" {
                n688 = local read "NDO"() -> (w1452:T4)
                n689 = call "RTS Standard Test Set Time.vi"("Error In"=w1453, "Internal Moisture Test (511-B111) - 5 Days"=w1452) -> ("Error Out"=w1455:errorcluster, "Output"=w1454:T4)  [unwired: 8 in]
              }
              frame "511-B304 ISO Energy Consumption" {
                n690 = local read "ISO Energy Consumption"() -> (w1456:T4)
                n691 = call "RTS Standard Test Set Time.vi"("Error In"=w1457, "Internal Moisture Test (511-B111) - 5 Days"=w1456) -> ("Error Out"=w1459:errorcluster, "Output"=w1458:T4)  [unwired: 8 in]
              }
              frame "Custom Test" {
                n692 = local read "4-8"() -> (w1461:T4)
              }
            }
            n693 = local write "4-8"(w1421) -> ()
            n694 = Bundle By Name(cluster=w1423, "4-8"=w1421) -> (w1422:T13)
          }
          event Value Change {
            n695 = event-data() -> ("NewVal"=w1470:T5[])  [unwired: 1 in, 5 out]
            n696 = property on="Chamber 1-1" class="Arr (strict)"() -> ("Index Values"=w1467:u32[])  [unwired: 2 in, 2 out]
            n697 = local read "1-1"() -> (w1466:T4)
            n698 = Unbundle By Name(w1466) -> ("Standard Tests 1-1"=w1465:T8)
            n699 = Index Array(array=w1467, index=u32 0) -> (element=w1471:u32)
            n700 = call "RTS Calculate Door Openings.vi"("Error In"=w1469, "Standard Tests 1-1"=w1465, "Current Index"=w1471, "Input"=w1470) -> ("Error Out"=w1468:errorcluster, "Output"=w1462:T5[])  [unwired: 6 in]
            n701 = Bundle By Name(cluster=w1464, "1-1.Chamber 1-1"=w1462) -> (w1463:T13)
            n702 = property on="Chamber 1-1" class="Arr (strict)"("Value"=w1462) -> ()  [unwired: 2 in, 2 out]
          }
          event Value Change {
            n703 = event-data() -> ("NewVal"=w1482:T5[])  [unwired: 1 in, 5 out]
            n704 = property on="Chamber 1-2" class="Arr (strict)"() -> ("Index Values"=w1485:u32[])  [unwired: 2 in, 2 out]
            n705 = local read "1-1"() -> (w1478:T4)
            n706 = Unbundle By Name(w1478) -> ("Standard Tests 1-1"=w1477:T8)
            n707 = Index Array(array=w1485, index=u32 0) -> (element=w1483:u32)
            n708 = call "RTS Calculate Door Openings.vi"("Error In"=w1481, "Standard Tests 1-1"=w1477, "Current Index"=w1483, "Input"=w1482) -> ("Error Out"=w1480:errorcluster, "Output"=w1474:T5[])  [unwired: 6 in]
            n709 = Bundle By Name(cluster=w1476, "1-1.Chamber 1-2"=w1474) -> (w1475:T13)
            n710 = property on="Chamber 1-2" class="Arr (strict)"("Value"=w1474) -> ()  [unwired: 2 in, 2 out]
          }
          event Value Change {
            n711 = event-data() -> ("NewVal"=w1495:T5[])  [unwired: 1 in, 5 out]
            n712 = local read "1-1"() -> (w1490:T4)
            n713 = property on="Chamber 1-3" class="Arr (strict)"() -> ("Index Values"=w1492:u32[])  [unwired: 2 in, 2 out]
            n714 = Unbundle By Name(w1490) -> ("Standard Tests 1-1"=w1489:T8)
            n715 = Index Array(array=w1492, index=u32 0) -> (element=w1496:u32)
            n716 = call "RTS Calculate Door Openings.vi"("Error In"=w1493, "Standard Tests 1-1"=w1489, "Current Index"=w1496, "Input"=w1495) -> ("Error Out"=w1494:errorcluster, "Output"=w1486:T5[])  [unwired: 6 in]
            n717 = Bundle By Name(cluster=w1488, "1-1.Chamber 1-3"=w1486) -> (w1487:T13)
            n718 = property on="Chamber 1-3" class="Arr (strict)"("Value"=w1486) -> ()  [unwired: 2 in, 2 out]
          }
          event Value Change {
            n719 = event-data() -> ("NewVal"=w1503:T5[])  [unwired: 1 in, 5 out]
            n720 = property on="Chamber 1-1" class="Arr (strict)"() -> ("Index Values"=w1504:u32[])  [unwired: 2 in, 2 out]
            n721 = Index Array(array=w1504, index=u32 0) -> (element=w1505:u32)
            n722 = call "RTS Calculate Door Openings.vi"("Error In"=w1502, "Current Index"=w1505, "Input"=w1503) -> ("Error Out"=w1501:errorcluster, "Output"=w1498:T5[])  [unwired: 7 in]
            n723 = property on="Chamber 1-1" class="Arr (strict)"("Value"=w1498) -> ()  [unwired: 2 in, 2 out]
            n724 = Bundle By Name(cluster=w1500, "1-2.Chamber 1-1"=w1498) -> (w1499:T13)
          }
          event Value Change {
            n725 = event-data() -> ("NewVal"=w1514:T5[])  [unwired: 1 in, 5 out]
            n726 = property on="Chamber 1-2" class="Arr (strict)"() -> ("Index Values"=w1515:u32[])  [unwired: 2 in, 2 out]
            n727 = Index Array(array=w1515, index=u32 0) -> (element=w1516:u32)
            n728 = call "RTS Calculate Door Openings.vi"("Error In"=w1513, "Current Index"=w1516, "Input"=w1514) -> ("Error Out"=w1512:errorcluster, "Output"=w1508:T5[])  [unwired: 7 in]
            n729 = Bundle By Name(cluster=w1510, "1-2.Chamber 1-2"=w1508) -> (w1509:T13)
            n730 = property on="Chamber 1-2" class="Arr (strict)"("Value"=w1508) -> ()  [unwired: 2 in, 2 out]
          }
          event Value Change {
            n731 = event-data() -> ("NewVal"=w1523:T5[])  [unwired: 1 in, 5 out]
            n732 = property on="Chamber 1-3" class="Arr (strict)"() -> ("Index Values"=w1524:u32[])  [unwired: 2 in, 2 out]
            n733 = Index Array(array=w1524, index=u32 0) -> (element=w1525:u32)
            n734 = call "RTS Calculate Door Openings.vi"("Error In"=w1522, "Current Index"=w1525, "Input"=w1523) -> ("Error Out"=w1521:errorcluster, "Output"=w1518:T5[])  [unwired: 7 in]
            n735 = Bundle By Name(cluster=w1520, "1-2.Chamber 1-3"=w1518) -> (w1519:T13)
            n736 = property on="Chamber 1-3" class="Arr (strict)"("Value"=w1518) -> ()  [unwired: 2 in, 2 out]
          }
          event Value Change {
            n737 = event-data() -> ("NewVal"=w1534:T5[])  [unwired: 1 in, 5 out]
            n738 = property on="Chamber 1-1" class="Arr (strict)"() -> ("Index Values"=w1535:u32[])  [unwired: 2 in, 2 out]
            n739 = Index Array(array=w1535, index=u32 0) -> (element=w1536:u32)
            n740 = call "RTS Calculate Door Openings.vi"("Error In"=w1533, "Current Index"=w1536, "Input"=w1534) -> ("Error Out"=w1532:errorcluster, "Output"=w1528:T5[])  [unwired: 7 in]
            n741 = Bundle By Name(cluster=w1530, "1-3.Chamber 1-1"=w1528) -> (w1529:T13)
            n742 = property on="Chamber 1-1" class="Arr (strict)"("Value"=w1528) -> ()  [unwired: 2 in, 2 out]
          }
          event Value Change {
            n743 = event-data() -> ("NewVal"=w1544:T5[])  [unwired: 1 in, 5 out]
            n744 = property on="Chamber 1-2" class="Arr (strict)"() -> ("Index Values"=w1547:u32[])  [unwired: 2 in, 2 out]
            n745 = Index Array(array=w1547, index=u32 0) -> (element=w1545:u32)
            n746 = call "RTS Calculate Door Openings.vi"("Error In"=w1543, "Current Index"=w1545, "Input"=w1544) -> ("Error Out"=w1542:errorcluster, "Output"=w1538:T5[])  [unwired: 7 in]
            n747 = Bundle By Name(cluster=w1540, "1-3.Chamber 1-2"=w1538) -> (w1539:T13)
            n748 = property on="Chamber 1-2" class="Arr (strict)"("Value"=w1538) -> ()  [unwired: 2 in, 2 out]
          }
          event Value Change {
            n749 = event-data() -> ("NewVal"=w1554:T5[])  [unwired: 1 in, 5 out]
            n750 = property on="Chamber 1-3" class="Arr (strict)"() -> ("Index Values"=w1557:u32[])  [unwired: 2 in, 2 out]
            n751 = Index Array(array=w1557, index=u32 0) -> (element=w1555:u32)
            n752 = call "RTS Calculate Door Openings.vi"("Error In"=w1553, "Current Index"=w1555, "Input"=w1554) -> ("Error Out"=w1552:errorcluster, "Output"=w1548:T5[])  [unwired: 7 in]
            n753 = Bundle By Name(cluster=w1550, "1-3.Chamber 1-3"=w1548) -> (w1549:T13)
            n754 = property on="Chamber 1-3" class="Arr (strict)"("Value"=w1548) -> ()  [unwired: 2 in, 2 out]
          }
          event Value Change {
            n755 = event-data() -> ("NewVal"=w1564:T5[])  [unwired: 1 in, 5 out]
            n756 = property on="Chamber 1-1" class="Arr (strict)"() -> ("Index Values"=w1565:u32[])  [unwired: 2 in, 2 out]
            n757 = Index Array(array=w1565, index=u32 0) -> (element=w1566:u32)
            n758 = call "RTS Calculate Door Openings.vi"("Error In"=w1563, "Current Index"=w1566, "Input"=w1564) -> ("Error Out"=w1562:errorcluster, "Output"=w1558:T5[])  [unwired: 7 in]
            n759 = Bundle By Name(cluster=w1560, "1-4.Chamber 1-1"=w1558) -> (w1559:T13)
            n760 = property on="Chamber 1-1" class="Arr (strict)"("Value"=w1558) -> ()  [unwired: 2 in, 2 out]
          }
          event Value Change {
            n761 = event-data() -> ("NewVal"=w1575:T5[])  [unwired: 1 in, 5 out]
            n762 = property on="Chamber 1-2" class="Arr (strict)"() -> ("Index Values"=w1574:u32[])  [unwired: 2 in, 2 out]
            n763 = Index Array(array=w1574, index=u32 0) -> (element=w1576:u32)
            n764 = call "RTS Calculate Door Openings.vi"("Error In"=w1573, "Current Index"=w1576, "Input"=w1575) -> ("Error Out"=w1572:errorcluster, "Output"=w1568:T5[])  [unwired: 7 in]
            n765 = Bundle By Name(cluster=w1570, "1-4.Chamber 1-2"=w1568) -> (w1569:T13)
            n766 = property on="Chamber 1-2" class="Arr (strict)"("Value"=w1568) -> ()  [unwired: 2 in, 2 out]
          }
          event Value Change {
            n767 = event-data() -> ("NewVal"=w1584:T5[])  [unwired: 1 in, 5 out]
            n768 = property on="Chamber 1-3" class="Arr (strict)"() -> ("Index Values"=w1587:u32[])  [unwired: 2 in, 2 out]
            n769 = Index Array(array=w1587, index=u32 0) -> (element=w1585:u32)
            n770 = call "RTS Calculate Door Openings.vi"("Error In"=w1583, "Current Index"=w1585, "Input"=w1584) -> ("Error Out"=w1582:errorcluster, "Output"=w1578:T5[])  [unwired: 7 in]
            n771 = Bundle By Name(cluster=w1580, "1-4.Chamber 1-3"=w1578) -> (w1579:T13)
            n772 = property on="Chamber 1-3" class="Arr (strict)"("Value"=w1578) -> ()  [unwired: 2 in, 2 out]
          }
          event Value Change {
            n773 = event-data() -> ("NewVal"=w1595:T5[])  [unwired: 1 in, 5 out]
            n774 = property on="Chamber 1-1" class="Arr (strict)"() -> ("Index Values"=w1594:u32[])  [unwired: 2 in, 2 out]
            n775 = Index Array(array=w1594, index=u32 0) -> (element=w1596:u32)
            n776 = call "RTS Calculate Door Openings.vi"("Error In"=w1593, "Current Index"=w1596, "Input"=w1595) -> ("Error Out"=w1592:errorcluster, "Output"=w1588:T5[])  [unwired: 7 in]
            n777 = Bundle By Name(cluster=w1590, "1-5.Chamber 1-1"=w1588) -> (w1589:T13)
            n778 = property on="Chamber 1-1" class="Arr (strict)"("Value"=w1588) -> ()  [unwired: 2 in, 2 out]
          }
          event Value Change {
            n779 = event-data() -> ("NewVal"=w1604:T5[])  [unwired: 1 in, 5 out]
            n780 = property on="Chamber 1-2" class="Arr (strict)"() -> ("Index Values"=w1607:u32[])  [unwired: 2 in, 2 out]
            n781 = Index Array(array=w1607, index=u32 0) -> (element=w1605:u32)
            n782 = call "RTS Calculate Door Openings.vi"("Error In"=w1603, "Current Index"=w1605, "Input"=w1604) -> ("Error Out"=w1602:errorcluster, "Output"=w1598:T5[])  [unwired: 7 in]
            n783 = Bundle By Name(cluster=w1600, "1-5.Chamber 1-2"=w1598) -> (w1599:T13)
            n784 = property on="Chamber 1-2" class="Arr (strict)"("Value"=w1598) -> ()  [unwired: 2 in, 2 out]
          }
          event Value Change {
            n785 = event-data() -> ("NewVal"=w1613:T5[])  [unwired: 1 in, 5 out]
            n786 = property on="Chamber 1-3" class="Arr (strict)"() -> ("Index Values"=w1612:u32[])  [unwired: 2 in, 2 out]
            n787 = Index Array(array=w1612, index=u32 0) -> (element=w1616:u32)
            n788 = call "RTS Calculate Door Openings.vi"("Error In"=w1615, "Current Index"=w1616, "Input"=w1613) -> ("Error Out"=w1614:errorcluster, "Output"=w1608:T5[])  [unwired: 7 in]
            n789 = Bundle By Name(cluster=w1610, "1-5.Chamber 1-3"=w1608) -> (w1609:T13)
            n790 = property on="Chamber 1-3" class="Arr (strict)"("Value"=w1608) -> ()  [unwired: 2 in, 2 out]
          }
          event Value Change {
            n791 = event-data() -> ("NewVal"=w1624:T5[])  [unwired: 1 in, 5 out]
            n792 = property on="Chamber 1-1" class="Arr (strict)"() -> ("Index Values"=w1627:u32[])  [unwired: 2 in, 2 out]
            n793 = Index Array(array=w1627, index=u32 0) -> (element=w1625:u32)
            n794 = call "RTS Calculate Door Openings.vi"("Error In"=w1623, "Current Index"=w1625, "Input"=w1624) -> ("Error Out"=w1622:errorcluster, "Output"=w1618:T5[])  [unwired: 7 in]
            n795 = Bundle By Name(cluster=w1620, "1-6.Chamber 1-1"=w1618) -> (w1619:T13)
            n796 = property on="Chamber 1-1" class="Arr (strict)"("Value"=w1618) -> ()  [unwired: 2 in, 2 out]
          }
          event Value Change {
            n797 = event-data() -> ("NewVal"=w1632:T5[])  [unwired: 1 in, 5 out]
            n798 = property on="Chamber 1-2" class="Arr (strict)"() -> ("Index Values"=w1637:u32[])  [unwired: 2 in, 2 out]
            n799 = Index Array(array=w1637, index=u32 0) -> (element=w1635:u32)
            n800 = call "RTS Calculate Door Openings.vi"("Error In"=w1634, "Current Index"=w1635, "Input"=w1632) -> ("Error Out"=w1633:errorcluster, "Output"=w1628:T5[])  [unwired: 7 in]
            n801 = Bundle By Name(cluster=w1630, "1-6.Chamber 1-2"=w1628) -> (w1629:T13)
            n802 = property on="Chamber 1-2" class="Arr (strict)"("Value"=w1628) -> ()  [unwired: 2 in, 2 out]
          }
          event Value Change {
            n803 = event-data() -> ("NewVal"=w1644:T5[])  [unwired: 1 in, 5 out]
            n804 = property on="Chamber 1-3" class="Arr (strict)"() -> ("Index Values"=w1647:u32[])  [unwired: 2 in, 2 out]
            n805 = Index Array(array=w1647, index=u32 0) -> (element=w1645:u32)
            n806 = call "RTS Calculate Door Openings.vi"("Error In"=w1643, "Current Index"=w1645, "Input"=w1644) -> ("Error Out"=w1642:errorcluster, "Output"=w1638:T5[])  [unwired: 7 in]
            n807 = Bundle By Name(cluster=w1640, "1-6.Chamber 1-3"=w1638) -> (w1639:T13)
            n808 = property on="Chamber 1-3" class="Arr (strict)"("Value"=w1638) -> ()  [unwired: 2 in, 2 out]
          }
          event Value Change {
            n809 = event-data() -> ("NewVal"=w1652:T5[])  [unwired: 1 in, 5 out]
            n810 = property on="Chamber 1-1" class="Arr (strict)"() -> ("Index Values"=w1657:u32[])  [unwired: 2 in, 2 out]
            n811 = Index Array(array=w1657, index=u32 0) -> (element=w1655:u32)
            n812 = call "RTS Calculate Door Openings.vi"("Error In"=w1654, "Current Index"=w1655, "Input"=w1652) -> ("Error Out"=w1653:errorcluster, "Output"=w1648:T5[])  [unwired: 7 in]
            n813 = Bundle By Name(cluster=w1650, "1-7.Chamber 1-1"=w1648) -> (w1649:T13)
            n814 = property on="Chamber 1-1" class="Arr (strict)"("Value"=w1648) -> ()  [unwired: 2 in, 2 out]
          }
          event Value Change {
            n815 = event-data() -> ("NewVal"=w1663:T5[])  [unwired: 1 in, 5 out]
            n816 = property on="Chamber 1-2" class="Arr (strict)"() -> ("Index Values"=w1664:u32[])  [unwired: 2 in, 2 out]
            n817 = Index Array(array=w1664, index=u32 0) -> (element=w1665:u32)
            n818 = call "RTS Calculate Door Openings.vi"("Error In"=w1662, "Current Index"=w1665, "Input"=w1663) -> ("Error Out"=w1661:errorcluster, "Output"=w1658:T5[])  [unwired: 7 in]
            n819 = Bundle By Name(cluster=w1660, "1-7.Chamber 1-2"=w1658) -> (w1659:T13)
            n820 = property on="Chamber 1-2" class="Arr (strict)"("Value"=w1658) -> ()  [unwired: 2 in, 2 out]
          }
          event Value Change {
            n821 = event-data() -> ("NewVal"=w1674:T5[])  [unwired: 1 in, 5 out]
            n822 = property on="Chamber 1-3" class="Arr (strict)"() -> ("Index Values"=w1677:u32[])  [unwired: 2 in, 2 out]
            n823 = Index Array(array=w1677, index=u32 0) -> (element=w1675:u32)
            n824 = call "RTS Calculate Door Openings.vi"("Error In"=w1673, "Current Index"=w1675, "Input"=w1674) -> ("Error Out"=w1672:errorcluster, "Output"=w1668:T5[])  [unwired: 7 in]
            n825 = Bundle By Name(cluster=w1670, "1-7.Chamber 1-3"=w1668) -> (w1669:T13)
            n826 = property on="Chamber 1-3" class="Arr (strict)"("Value"=w1668) -> ()  [unwired: 2 in, 2 out]
          }
          event Value Change {
            n827 = event-data() -> ("NewVal"=w1684:T5[])  [unwired: 1 in, 5 out]
            n828 = property on="Chamber 1-1" class="Arr (strict)"() -> ("Index Values"=w1687:u32[])  [unwired: 2 in, 2 out]
            n829 = Index Array(array=w1687, index=u32 0) -> (element=w1685:u32)
            n830 = call "RTS Calculate Door Openings.vi"("Error In"=w1683, "Current Index"=w1685, "Input"=w1684) -> ("Error Out"=w1682:errorcluster, "Output"=w1678:T5[])  [unwired: 7 in]
            n831 = property on="Chamber 1-1" class="Arr (strict)"("Value"=w1678) -> ()  [unwired: 2 in, 2 out]
            n832 = Bundle By Name(cluster=w1680, "1-8.Chamber 1-1"=w1678) -> (w1679:T13)
          }
          event Value Change {
            n833 = event-data() -> ("NewVal"=w1692:T5[])  [unwired: 1 in, 5 out]
            n834 = property on="Chamber 1-2" class="Arr (strict)"() -> ("Index Values"=w1697:u32[])  [unwired: 2 in, 2 out]
            n835 = Index Array(array=w1697, index=u32 0) -> (element=w1695:u32)
            n836 = call "RTS Calculate Door Openings.vi"("Error In"=w1694, "Current Index"=w1695, "Input"=w1692) -> ("Error Out"=w1693:errorcluster, "Output"=w1688:T5[])  [unwired: 7 in]
            n837 = Bundle By Name(cluster=w1690, "1-8.Chamber 1-2"=w1688) -> (w1689:T13)
            n838 = property on="Chamber 1-2" class="Arr (strict)"("Value"=w1688) -> ()  [unwired: 2 in, 2 out]
          }
          event Value Change {
            n839 = event-data() -> ("NewVal"=w1702:T5[])  [unwired: 1 in, 5 out]
            n840 = property on="Chamber 1-3" class="Arr (strict)"() -> ("Index Values"=w1707:u32[])  [unwired: 2 in, 2 out]
            n841 = Index Array(array=w1707, index=u32 0) -> (element=w1705:u32)
            n842 = call "RTS Calculate Door Openings.vi"("Error In"=w1704, "Current Index"=w1705, "Input"=w1702) -> ("Error Out"=w1703:errorcluster, "Output"=w1698:T5[])  [unwired: 7 in]
            n843 = Bundle By Name(cluster=w1700, "1-8.Chamber 1-3"=w1698) -> (w1699:T13)
            n844 = property on="Chamber 1-3" class="Arr (strict)"("Value"=w1698) -> ()  [unwired: 2 in, 2 out]
          }
          event Value Change {
            n845 = event-data() -> ("NewVal"=w1714:T5[])  [unwired: 1 in, 5 out]
            n846 = property on="Chamber 1-1" class="Arr (strict)"() -> ("Index Values"=w1717:u32[])  [unwired: 2 in, 2 out]
            n847 = Index Array(array=w1717, index=u32 0) -> (element=w1715:u32)
            n848 = call "RTS Calculate Door Openings.vi"("Error In"=w1713, "Current Index"=w1715, "Input"=w1714) -> ("Error Out"=w1712:errorcluster, "Output"=w1708:T5[])  [unwired: 7 in]
            n849 = Bundle By Name(cluster=w1710, "2-1.Chamber 1-1"=w1708) -> (w1709:T13)
            n850 = property on="Chamber 1-1" class="Arr (strict)"("Value"=w1708) -> ()  [unwired: 2 in, 2 out]
          }
          event Value Change {
            n851 = event-data() -> ("NewVal"=w1724:T5[])  [unwired: 1 in, 5 out]
            n852 = property on="Chamber 1-2" class="Arr (strict)"() -> ("Index Values"=w1725:u32[])  [unwired: 2 in, 2 out]
            n853 = Index Array(array=w1725, index=u32 0) -> (element=w1726:u32)
            n854 = call "RTS Calculate Door Openings.vi"("Error In"=w1722, "Current Index"=w1726, "Input"=w1724) -> ("Error Out"=w1721:errorcluster, "Output"=w1718:T5[])  [unwired: 7 in]
            n855 = Bundle By Name(cluster=w1720, "2-1.Chamber 1-2"=w1718) -> (w1719:T13)
            n856 = property on="Chamber 1-2" class="Arr (strict)"("Value"=w1718) -> ()  [unwired: 2 in, 2 out]
          }
          event Value Change {
            n857 = event-data() -> ("NewVal"=w1733:T5[])  [unwired: 1 in, 5 out]
            n858 = property on="Chamber 1-3" class="Arr (strict)"() -> ("Index Values"=w1734:u32[])  [unwired: 2 in, 2 out]
            n859 = Index Array(array=w1734, index=u32 0) -> (element=w1736:u32)
            n860 = call "RTS Calculate Door Openings.vi"("Error In"=w1732, "Current Index"=w1736, "Input"=w1733) -> ("Error Out"=w1731:errorcluster, "Output"=w1728:T5[])  [unwired: 7 in]
            n861 = Bundle By Name(cluster=w1730, "2-1.Chamber 1-3"=w1728) -> (w1729:T13)
            n862 = property on="Chamber 1-3" class="Arr (strict)"("Value"=w1728) -> ()  [unwired: 2 in, 2 out]
          }
          event Value Change {
            n863 = event-data() -> ("NewVal"=w1744:T5[])  [unwired: 1 in, 5 out]
            n864 = property on="Chamber 1-1" class="Arr (strict)"() -> ("Index Values"=w1745:u32[])  [unwired: 2 in, 2 out]
            n865 = Index Array(array=w1745, index=u32 0) -> (element=w1746:u32)
            n866 = call "RTS Calculate Door Openings.vi"("Error In"=w1743, "Current Index"=w1746, "Input"=w1744) -> ("Error Out"=w1742:errorcluster, "Output"=w1738:T5[])  [unwired: 7 in]
            n867 = Bundle By Name(cluster=w1740, "2-2.Chamber 1-1"=w1738) -> (w1739:T13)
            n868 = property on="Chamber 1-1" class="Arr (strict)"("Value"=w1738) -> ()  [unwired: 2 in, 2 out]
          }
          event Value Change {
            n869 = event-data() -> ("NewVal"=w1754:T5[])  [unwired: 1 in, 5 out]
            n870 = property on="Chamber 1-2" class="Arr (strict)"() -> ("Index Values"=w1755:u32[])  [unwired: 2 in, 2 out]
            n871 = Index Array(array=w1755, index=u32 0) -> (element=w1756:u32)
            n872 = call "RTS Calculate Door Openings.vi"("Error In"=w1752, "Current Index"=w1756, "Input"=w1754) -> ("Error Out"=w1751:errorcluster, "Output"=w1748:T5[])  [unwired: 7 in]
            n873 = Bundle By Name(cluster=w1750, "2-2.Chamber 1-2"=w1748) -> (w1749:T13)
            n874 = property on="Chamber 1-2" class="Arr (strict)"("Value"=w1748) -> ()  [unwired: 2 in, 2 out]
          }
          event Value Change {
            n875 = event-data() -> ("NewVal"=w1764:T5[])  [unwired: 1 in, 5 out]
            n876 = property on="Chamber 1-3" class="Arr (strict)"() -> ("Index Values"=w1765:u32[])  [unwired: 2 in, 2 out]
            n877 = Index Array(array=w1765, index=u32 0) -> (element=w1766:u32)
            n878 = call "RTS Calculate Door Openings.vi"("Error In"=w1762, "Current Index"=w1766, "Input"=w1764) -> ("Error Out"=w1761:errorcluster, "Output"=w1758:T5[])  [unwired: 7 in]
            n879 = Bundle By Name(cluster=w1760, "2-2.Chamber 1-3"=w1758) -> (w1759:T13)
            n880 = property on="Chamber 1-3" class="Arr (strict)"("Value"=w1758) -> ()  [unwired: 2 in, 2 out]
          }
          event Value Change {
            n881 = event-data() -> ("NewVal"=w1771:T5[])  [unwired: 1 in, 5 out]
            n882 = property on="Chamber 1-1" class="Arr (strict)"() -> ("Index Values"=w1772:u32[])  [unwired: 2 in, 2 out]
            n883 = Index Array(array=w1772, index=u32 0) -> (element=w1776:u32)
            n884 = call "RTS Calculate Door Openings.vi"("Error In"=w1774, "Current Index"=w1776, "Input"=w1771) -> ("Error Out"=w1773:errorcluster, "Output"=w1768:T5[])  [unwired: 7 in]
            n885 = Bundle By Name(cluster=w1770, "2-3.Chamber 1-1"=w1768) -> (w1769:T13)
            n886 = property on="Chamber 1-1" class="Arr (strict)"("Value"=w1768) -> ()  [unwired: 2 in, 2 out]
          }
          event Value Change {
            n887 = event-data() -> ("NewVal"=w1782:T5[])  [unwired: 1 in, 5 out]
            n888 = property on="Chamber 1-2" class="Arr (strict)"() -> ("Index Values"=w1783:u32[])  [unwired: 2 in, 2 out]
            n889 = Index Array(array=w1783, index=u32 0) -> (element=w1786:u32)
            n890 = call "RTS Calculate Door Openings.vi"("Error In"=w1785, "Current Index"=w1786, "Input"=w1782) -> ("Error Out"=w1784:errorcluster, "Output"=w1778:T5[])  [unwired: 7 in]
            n891 = Bundle By Name(cluster=w1780, "2-3.Chamber 1-2"=w1778) -> (w1779:T13)
            n892 = property on="Chamber 1-2" class="Arr (strict)"("Value"=w1778) -> ()  [unwired: 2 in, 2 out]
          }
          event Value Change {
            n893 = event-data() -> ("NewVal"=w1795:T5[])  [unwired: 1 in, 5 out]
            n894 = property on="Chamber 1-3" class="Arr (strict)"() -> ("Index Values"=w1791:u32[])  [unwired: 2 in, 2 out]
            n895 = Index Array(array=w1791, index=u32 0) -> (element=w1796:u32)
            n896 = call "RTS Calculate Door Openings.vi"("Error In"=w1794, "Current Index"=w1796, "Input"=w1795) -> ("Error Out"=w1793:errorcluster, "Output"=w1788:T5[])  [unwired: 7 in]
            n897 = Bundle By Name(cluster=w1790, "2-3.Chamber 1-3"=w1788) -> (w1789:T13)
            n898 = property on="Chamber 1-3" class="Arr (strict)"("Value"=w1788) -> ()  [unwired: 2 in, 2 out]
          }
          event Value Change {
            n899 = event-data() -> ("NewVal"=w1803:T5[])  [unwired: 1 in, 5 out]
            n900 = property on="Chamber 1-1" class="Arr (strict)"() -> ("Index Values"=w1802:u32[])  [unwired: 2 in, 2 out]
            n901 = Index Array(array=w1802, index=u32 0) -> (element=w1806:u32)
            n902 = call "RTS Calculate Door Openings.vi"("Error In"=w1805, "Current Index"=w1806, "Input"=w1803) -> ("Error Out"=w1804:errorcluster, "Output"=w1798:T5[])  [unwired: 7 in]
            n903 = Bundle By Name(cluster=w1800, "2-4.Chamber 1-1"=w1798) -> (w1799:T13)
            n904 = property on="Chamber 1-1" class="Arr (strict)"("Value"=w1798) -> ()  [unwired: 2 in, 2 out]
          }
          event Value Change {
            n905 = event-data() -> ("NewVal"=w1815:T5[])  [unwired: 1 in, 5 out]
            n906 = property on="Chamber 1-2" class="Arr (strict)"() -> ("Index Values"=w1811:u32[])  [unwired: 2 in, 2 out]
            n907 = Index Array(array=w1811, index=u32 0) -> (element=w1816:u32)
            n908 = call "RTS Calculate Door Openings.vi"("Error In"=w1813, "Current Index"=w1816, "Input"=w1815) -> ("Error Out"=w1812:errorcluster, "Output"=w1808:T5[])  [unwired: 7 in]
            n909 = property on="Chamber 1-2" class="Arr (strict)"("Value"=w1808) -> ()  [unwired: 2 in, 2 out]
            n910 = Bundle By Name(cluster=w1810, "2-4.Chamber 1-2"=w1808) -> (w1809:T13)
          }
          event Value Change {
            n911 = event-data() -> ("NewVal"=w1822:T5[])  [unwired: 1 in, 5 out]
            n912 = property on="Chamber 1-3" class="Arr (strict)"() -> ("Index Values"=w1823:u32[])  [unwired: 2 in, 2 out]
            n913 = Index Array(array=w1823, index=u32 0) -> (element=w1826:u32)
            n914 = call "RTS Calculate Door Openings.vi"("Error In"=w1825, "Current Index"=w1826, "Input"=w1822) -> ("Error Out"=w1824:errorcluster, "Output"=w1818:T5[])  [unwired: 7 in]
            n915 = Bundle By Name(cluster=w1820, "2-4.Chamber 1-3"=w1818) -> (w1819:T13)
            n916 = property on="Chamber 1-3" class="Arr (strict)"("Value"=w1818) -> ()  [unwired: 2 in, 2 out]
          }
          event Value Change {
            n917 = event-data() -> ("NewVal"=w1831:T5[])  [unwired: 1 in, 5 out]
            n918 = property on="Chamber 1-1" class="Arr (strict)"() -> ("Index Values"=w1832:u32[])  [unwired: 2 in, 2 out]
            n919 = Index Array(array=w1832, index=u32 0) -> (element=w1836:u32)
            n920 = call "RTS Calculate Door Openings.vi"("Error In"=w1835, "Current Index"=w1836, "Input"=w1831) -> ("Error Out"=w1834:errorcluster, "Output"=w1828:T5[])  [unwired: 7 in]
            n921 = property on="Chamber 1-1" class="Arr (strict)"("Value"=w1828) -> ()  [unwired: 2 in, 2 out]
            n922 = Bundle By Name(cluster=w1830, "2-5.Chamber 1-1"=w1828) -> (w1829:T13)
          }
          event Value Change {
            n923 = event-data() -> ("NewVal"=w1843:T5[])  [unwired: 1 in, 5 out]
            n924 = property on="Chamber 1-2" class="Arr (strict)"() -> ("Index Values"=w1842:u32[])  [unwired: 2 in, 2 out]
            n925 = Index Array(array=w1842, index=u32 0) -> (element=w1846:u32)
            n926 = call "RTS Calculate Door Openings.vi"("Error In"=w1845, "Current Index"=w1846, "Input"=w1843) -> ("Error Out"=w1844:errorcluster, "Output"=w1838:T5[])  [unwired: 7 in]
            n927 = property on="Chamber 1-2" class="Arr (strict)"("Value"=w1838) -> ()  [unwired: 2 in, 2 out]
            n928 = Bundle By Name(cluster=w1840, "2-5.Chamber 1-2"=w1838) -> (w1839:T13)
          }
          event Value Change {
            n929 = event-data() -> ("NewVal"=w1852:T5[])  [unwired: 1 in, 5 out]
            n930 = property on="Chamber 1-3" class="Arr (strict)"() -> ("Index Values"=w1853:u32[])  [unwired: 2 in, 2 out]
            n931 = Index Array(array=w1853, index=u32 0) -> (element=w1856:u32)
            n932 = call "RTS Calculate Door Openings.vi"("Error In"=w1855, "Current Index"=w1856, "Input"=w1852) -> ("Error Out"=w1854:errorcluster, "Output"=w1848:T5[])  [unwired: 7 in]
            n933 = Bundle By Name(cluster=w1850, "2-5.Chamber 1-3"=w1848) -> (w1849:T13)
            n934 = property on="Chamber 1-3" class="Arr (strict)"("Value"=w1848) -> ()  [unwired: 2 in, 2 out]
          }
          event Value Change {
            n935 = event-data() -> ("NewVal"=w1864:T5[])  [unwired: 1 in, 5 out]
            n936 = property on="Chamber 1-1" class="Arr (strict)"() -> ("Index Values"=w1865:u32[])  [unwired: 2 in, 2 out]
            n937 = Index Array(array=w1865, index=u32 0) -> (element=w1866:u32)
            n938 = call "RTS Calculate Door Openings.vi"("Error In"=w1862, "Current Index"=w1866, "Input"=w1864) -> ("Error Out"=w1861:errorcluster, "Output"=w1858:T5[])  [unwired: 7 in]
            n939 = Bundle By Name(cluster=w1860, "2-6.Chamber 1-1"=w1858) -> (w1859:T13)
            n940 = property on="Chamber 1-1" class="Arr (strict)"("Value"=w1858) -> ()  [unwired: 2 in, 2 out]
          }
          event Value Change {
            n941 = event-data() -> ("NewVal"=w1872:T5[])  [unwired: 1 in, 5 out]
            n942 = property on="Chamber 1-2" class="Arr (strict)"() -> ("Index Values"=w1871:u32[])  [unwired: 2 in, 2 out]
            n943 = Index Array(array=w1871, index=u32 0) -> (element=w1875:u32)
            n944 = call "RTS Calculate Door Openings.vi"("Error In"=w1874, "Current Index"=w1875, "Input"=w1872) -> ("Error Out"=w1873:errorcluster, "Output"=w1868:T5[])  [unwired: 7 in]
            n945 = Bundle By Name(cluster=w1870, "2-6.Chamber 1-2"=w1868) -> (w1869:T13)
            n946 = property on="Chamber 1-2" class="Arr (strict)"("Value"=w1868) -> ()  [unwired: 2 in, 2 out]
          }
          event Value Change {
            n947 = event-data() -> ("NewVal"=w1885:T5[])  [unwired: 1 in, 5 out]
            n948 = property on="Chamber 1-3" class="Arr (strict)"() -> ("Index Values"=w1882:u32[])  [unwired: 2 in, 2 out]
            n949 = Index Array(array=w1882, index=u32 0) -> (element=w1886:u32)
            n950 = call "RTS Calculate Door Openings.vi"("Error In"=w1884, "Current Index"=w1886, "Input"=w1885) -> ("Error Out"=w1883:errorcluster, "Output"=w1878:T5[])  [unwired: 7 in]
            n951 = Bundle By Name(cluster=w1880, "2-6.Chamber 1-3"=w1878) -> (w1879:T13)
            n952 = property on="Chamber 1-3" class="Arr (strict)"("Value"=w1878) -> ()  [unwired: 2 in, 2 out]
          }
          event Value Change {
            n953 = event-data() -> ("NewVal"=w1891:T5[])  [unwired: 1 in, 5 out]
            n954 = property on="Chamber 1-1" class="Arr (strict)"() -> ("Index Values"=w1892:u32[])  [unwired: 2 in, 2 out]
            n955 = Index Array(array=w1892, index=u32 0) -> (element=w1896:u32)
            n956 = call "RTS Calculate Door Openings.vi"("Error In"=w1894, "Current Index"=w1896, "Input"=w1891) -> ("Error Out"=w1895:errorcluster, "Output"=w1888:T5[])  [unwired: 7 in]
            n957 = property on="Chamber 1-1" class="Arr (strict)"("Value"=w1888) -> ()  [unwired: 2 in, 2 out]
            n958 = Bundle By Name(cluster=w1890, "2-7.Chamber 1-1"=w1888) -> (w1889:T13)
          }
          event Value Change {
            n959 = event-data() -> ("NewVal"=w1903:T5[])  [unwired: 1 in, 5 out]
            n960 = property on="Chamber 1-2" class="Arr (strict)"() -> ("Index Values"=w1902:u32[])  [unwired: 2 in, 2 out]
            n961 = Index Array(array=w1902, index=u32 0) -> (element=w1906:u32)
            n962 = call "RTS Calculate Door Openings.vi"("Error In"=w1905, "Current Index"=w1906, "Input"=w1903) -> ("Error Out"=w1904:errorcluster, "Output"=w1898:T5[])  [unwired: 7 in]
            n963 = Bundle By Name(cluster=w1900, "2-7.Chamber 1-2"=w1898) -> (w1899:T13)
            n964 = property on="Chamber 1-2" class="Arr (strict)"("Value"=w1898) -> ()  [unwired: 2 in, 2 out]
          }
          event Value Change {
            n965 = event-data() -> ("NewVal"=w1911:T5[])  [unwired: 1 in, 5 out]
            n966 = property on="Chamber 1-3" class="Arr (strict)"() -> ("Index Values"=w1912:u32[])  [unwired: 2 in, 2 out]
            n967 = Index Array(array=w1912, index=u32 0) -> (element=w1915:u32)
            n968 = call "RTS Calculate Door Openings.vi"("Error In"=w1914, "Current Index"=w1915, "Input"=w1911) -> ("Error Out"=w1913:errorcluster, "Output"=w1908:T5[])  [unwired: 7 in]
            n969 = Bundle By Name(cluster=w1910, "2-7.Chamber 1-3"=w1908) -> (w1909:T13)
            n970 = property on="Chamber 1-3" class="Arr (strict)"("Value"=w1908) -> ()  [unwired: 2 in, 2 out]
          }
          event Value Change {
            n971 = event-data() -> ("NewVal"=w1924:T5[])  [unwired: 1 in, 5 out]
            n972 = property on="Chamber 1-1" class="Arr (strict)"() -> ("Index Values"=w1927:u32[])  [unwired: 2 in, 2 out]
            n973 = Index Array(array=w1927, index=u32 0) -> (element=w1925:u32)
            n974 = call "RTS Calculate Door Openings.vi"("Error In"=w1922, "Current Index"=w1925, "Input"=w1924) -> ("Error Out"=w1921:errorcluster, "Output"=w1918:T5[])  [unwired: 7 in]
            n975 = Bundle By Name(cluster=w1920, "2-8.Chamber 1-1"=w1918) -> (w1919:T13)
            n976 = property on="Chamber 1-1" class="Arr (strict)"("Value"=w1918) -> ()  [unwired: 2 in, 2 out]
          }
          event Value Change {
            n977 = event-data() -> ("NewVal"=w1932:T5[])  [unwired: 1 in, 5 out]
            n978 = property on="Chamber 1-2" class="Arr (strict)"() -> ("Index Values"=w1931:u32[])  [unwired: 2 in, 2 out]
            n979 = Index Array(array=w1931, index=u32 0) -> (element=w1935:u32)
            n980 = call "RTS Calculate Door Openings.vi"("Error In"=w1934, "Current Index"=w1935, "Input"=w1932) -> ("Error Out"=w1933:errorcluster, "Output"=w1928:T5[])  [unwired: 7 in]
            n981 = Bundle By Name(cluster=w1930, "2-8.Chamber 1-2"=w1928) -> (w1929:T13)
            n982 = property on="Chamber 1-2" class="Arr (strict)"("Value"=w1928) -> ()  [unwired: 2 in, 2 out]
          }
          event Value Change {
            n983 = event-data() -> ("NewVal"=w1945:T5[])  [unwired: 1 in, 5 out]
            n984 = property on="Chamber 1-3" class="Arr (strict)"() -> ("Index Values"=w1941:u32[])  [unwired: 2 in, 2 out]
            n985 = Index Array(array=w1941, index=u32 0) -> (element=w1946:u32)
            n986 = call "RTS Calculate Door Openings.vi"("Error In"=w1943, "Current Index"=w1946, "Input"=w1945) -> ("Error Out"=w1942:errorcluster, "Output"=w1938:T5[])  [unwired: 7 in]
            n987 = Bundle By Name(cluster=w1940, "2-8.Chamber 1-3"=w1938) -> (w1939:T13)
            n988 = property on="Chamber 1-3" class="Arr (strict)"("Value"=w1938) -> ()  [unwired: 2 in, 2 out]
          }
          event Value Change {
            n989 = event-data() -> ("NewVal"=w1953:T5[])  [unwired: 1 in, 5 out]
            n990 = property on="Chamber 1-1" class="Arr (strict)"() -> ("Index Values"=w1951:u32[])  [unwired: 2 in, 2 out]
            n991 = Index Array(array=w1951, index=u32 0) -> (element=w1956:u32)
            n992 = call "RTS Calculate Door Openings.vi"("Error In"=w1955, "Current Index"=w1956, "Input"=w1953) -> ("Error Out"=w1954:errorcluster, "Output"=w1948:T5[])  [unwired: 7 in]
            n993 = Bundle By Name(cluster=w1950, "3-1.Chamber 1-1"=w1948) -> (w1949:T13)
            n994 = property on="Chamber 1-1" class="Arr (strict)"("Value"=w1948) -> ()  [unwired: 2 in, 2 out]
          }
          event Value Change {
            n995 = event-data() -> ("NewVal"=w1963:T5[])  [unwired: 1 in, 5 out]
            n996 = property on="Chamber 1-2" class="Arr (strict)"() -> ("Index Values"=w1961:u32[])  [unwired: 2 in, 2 out]
            n997 = Index Array(array=w1961, index=u32 0) -> (element=w1966:u32)
            n998 = call "RTS Calculate Door Openings.vi"("Error In"=w1965, "Current Index"=w1966, "Input"=w1963) -> ("Error Out"=w1964:errorcluster, "Output"=w1958:T5[])  [unwired: 7 in]
            n999 = Bundle By Name(cluster=w1960, "3-1.Chamber 1-2"=w1958) -> (w1959:T13)
            n1000 = property on="Chamber 1-2" class="Arr (strict)"("Value"=w1958) -> ()  [unwired: 2 in, 2 out]
          }
          event Value Change {
            n1001 = event-data() -> ("NewVal"=w1973:T5[])  [unwired: 1 in, 5 out]
            n1002 = property on="Chamber 1-3" class="Arr (strict)"() -> ("Index Values"=w1971:u32[])  [unwired: 2 in, 2 out]
            n1003 = Index Array(array=w1971, index=u32 0) -> (element=w1976:u32)
            n1004 = call "RTS Calculate Door Openings.vi"("Error In"=w1975, "Current Index"=w1976, "Input"=w1973) -> ("Error Out"=w1974:errorcluster, "Output"=w1968:T5[])  [unwired: 7 in]
            n1005 = Bundle By Name(cluster=w1970, "3-1.Chamber 1-3"=w1968) -> (w1969:T13)
            n1006 = property on="Chamber 1-3" class="Arr (strict)"("Value"=w1968) -> ()  [unwired: 2 in, 2 out]
          }
          event Value Change {
            n1007 = event-data() -> ("NewVal"=w1983:T5[])  [unwired: 1 in, 5 out]
            n1008 = property on="Chamber 1-1" class="Arr (strict)"() -> ("Index Values"=w1982:u32[])  [unwired: 2 in, 2 out]
            n1009 = Index Array(array=w1982, index=u32 0) -> (element=w1986:u32)
            n1010 = call "RTS Calculate Door Openings.vi"("Error In"=w1985, "Current Index"=w1986, "Input"=w1983) -> ("Error Out"=w1984:errorcluster, "Output"=w1978:T5[])  [unwired: 7 in]
            n1011 = Bundle By Name(cluster=w1980, "3-2.Chamber 1-1"=w1978) -> (w1979:T13)
            n1012 = property on="Chamber 1-1" class="Arr (strict)"("Value"=w1978) -> ()  [unwired: 2 in, 2 out]
          }
          event Value Change {
            n1013 = event-data() -> ("NewVal"=w1992:T5[])  [unwired: 1 in, 5 out]
            n1014 = property on="Chamber 1-2" class="Arr (strict)"() -> ("Index Values"=w1991:u32[])  [unwired: 2 in, 2 out]
            n1015 = Index Array(array=w1991, index=u32 0) -> (element=w1995:u32)
            n1016 = call "RTS Calculate Door Openings.vi"("Error In"=w1994, "Current Index"=w1995, "Input"=w1992) -> ("Error Out"=w1993:errorcluster, "Output"=w1988:T5[])  [unwired: 7 in]
            n1017 = Bundle By Name(cluster=w1990, "3-2.Chamber 1-2"=w1988) -> (w1989:T13)
            n1018 = property on="Chamber 1-2" class="Arr (strict)"("Value"=w1988) -> ()  [unwired: 2 in, 2 out]
          }
          event Value Change {
            n1019 = event-data() -> ("NewVal"=w2002:T5[])  [unwired: 1 in, 5 out]
            n1020 = property on="Chamber 1-3" class="Arr (strict)"() -> ("Index Values"=w2001:u32[])  [unwired: 2 in, 2 out]
            n1021 = Index Array(array=w2001, index=u32 0) -> (element=w2006:u32)
            n1022 = call "RTS Calculate Door Openings.vi"("Error In"=w2004, "Current Index"=w2006, "Input"=w2002) -> ("Error Out"=w2005:errorcluster, "Output"=w1998:T5[])  [unwired: 7 in]
            n1023 = Bundle By Name(cluster=w2000, "3-2.Chamber 1-3"=w1998) -> (w1999:T13)
            n1024 = property on="Chamber 1-3" class="Arr (strict)"("Value"=w1998) -> ()  [unwired: 2 in, 2 out]
          }
          event Value Change {
            n1025 = event-data() -> ("NewVal"=w2013:T5[])  [unwired: 1 in, 5 out]
            n1026 = property on="Chamber 1-1" class="Arr (strict)"() -> ("Index Values"=w2011:u32[])  [unwired: 2 in, 2 out]
            n1027 = Index Array(array=w2011, index=u32 0) -> (element=w2016:u32)
            n1028 = call "RTS Calculate Door Openings.vi"("Error In"=w2015, "Current Index"=w2016, "Input"=w2013) -> ("Error Out"=w2014:errorcluster, "Output"=w2008:T5[])  [unwired: 7 in]
            n1029 = property on="Chamber 1-1" class="Arr (strict)"("Value"=w2008) -> ()  [unwired: 2 in, 2 out]
            n1030 = Bundle By Name(cluster=w2010, "3-3.Chamber 1-1"=w2008) -> (w2009:T13)
          }
          event Value Change {
            n1031 = event-data() -> ("NewVal"=w2022:T5[])  [unwired: 1 in, 5 out]
            n1032 = property on="Chamber 1-2" class="Arr (strict)"() -> ("Index Values"=w2021:u32[])  [unwired: 2 in, 2 out]
            n1033 = Index Array(array=w2021, index=u32 0) -> (element=w2025:u32)
            n1034 = call "RTS Calculate Door Openings.vi"("Error In"=w2024, "Current Index"=w2025, "Input"=w2022) -> ("Error Out"=w2023:errorcluster, "Output"=w2018:T5[])  [unwired: 7 in]
            n1035 = Bundle By Name(cluster=w2020, "3-3.Chamber 1-2"=w2018) -> (w2019:T13)
            n1036 = property on="Chamber 1-2" class="Arr (strict)"("Value"=w2018) -> ()  [unwired: 2 in, 2 out]
          }
          event Value Change {
            n1037 = event-data() -> ("NewVal"=w2032:T5[])  [unwired: 1 in, 5 out]
            n1038 = property on="Chamber 1-3" class="Arr (strict)"() -> ("Index Values"=w2031:u32[])  [unwired: 2 in, 2 out]
            n1039 = Index Array(array=w2031, index=u32 0) -> (element=w2036:u32)
            n1040 = call "RTS Calculate Door Openings.vi"("Error In"=w2034, "Current Index"=w2036, "Input"=w2032) -> ("Error Out"=w2033:errorcluster, "Output"=w2028:T5[])  [unwired: 7 in]
            n1041 = Bundle By Name(cluster=w2030, "3-2.Chamber 1-3"=w2028) -> (w2029:T13)
            n1042 = property on="Chamber 1-3" class="Arr (strict)"("Value"=w2028) -> ()  [unwired: 2 in, 2 out]
          }
          event Value Change {
            n1043 = event-data() -> ("NewVal"=w2045:T5[])  [unwired: 1 in, 5 out]
            n1044 = property on="Chamber 1-1" class="Arr (strict)"() -> ("Index Values"=w2041:u32[])  [unwired: 2 in, 2 out]
            n1045 = Index Array(array=w2041, index=u32 0) -> (element=w2046:u32)
            n1046 = call "RTS Calculate Door Openings.vi"("Error In"=w2043, "Current Index"=w2046, "Input"=w2045) -> ("Error Out"=w2042:errorcluster, "Output"=w2038:T5[])  [unwired: 7 in]
            n1047 = Bundle By Name(cluster=w2040, "3-4.Chamber 1-1"=w2038) -> (w2039:T13)
            n1048 = property on="Chamber 1-1" class="Arr (strict)"("Value"=w2038) -> ()  [unwired: 2 in, 2 out]
          }
          event Value Change {
            n1049 = event-data() -> ("NewVal"=w2052:T5[])  [unwired: 1 in, 5 out]
            n1050 = property on="Chamber 1-2" class="Arr (strict)"() -> ("Index Values"=w2051:u32[])  [unwired: 2 in, 2 out]
            n1051 = Index Array(array=w2051, index=u32 0) -> (element=w2056:u32)
            n1052 = call "RTS Calculate Door Openings.vi"("Error In"=w2054, "Current Index"=w2056, "Input"=w2052) -> ("Error Out"=w2053:errorcluster, "Output"=w2048:T5[])  [unwired: 7 in]
            n1053 = Bundle By Name(cluster=w2050, "3-4.Chamber 1-2"=w2048) -> (w2049:T13)
            n1054 = property on="Chamber 1-2" class="Arr (strict)"("Value"=w2048) -> ()  [unwired: 2 in, 2 out]
          }
          event Value Change {
            n1055 = event-data() -> ("NewVal"=w2063:T5[])  [unwired: 1 in, 5 out]
            n1056 = property on="Chamber 1-3" class="Arr (strict)"() -> ("Index Values"=w2062:u32[])  [unwired: 2 in, 2 out]
            n1057 = Index Array(array=w2062, index=u32 0) -> (element=w2066:u32)
            n1058 = call "RTS Calculate Door Openings.vi"("Error In"=w2065, "Current Index"=w2066, "Input"=w2063) -> ("Error Out"=w2064:errorcluster, "Output"=w2058:T5[])  [unwired: 7 in]
            n1059 = Bundle By Name(cluster=w2060, "3-4.Chamber 1-3"=w2058) -> (w2059:T13)
            n1060 = property on="Chamber 1-3" class="Arr (strict)"("Value"=w2058) -> ()  [unwired: 2 in, 2 out]
          }
          event Value Change {
            n1061 = event-data() -> ("NewVal"=w2075:T5[])  [unwired: 1 in, 5 out]
            n1062 = property on="Chamber 1-1" class="Arr (strict)"() -> ("Index Values"=w2071:u32[])  [unwired: 2 in, 2 out]
            n1063 = Index Array(array=w2071, index=u32 0) -> (element=w2076:u32)
            n1064 = call "RTS Calculate Door Openings.vi"("Error In"=w2073, "Current Index"=w2076, "Input"=w2075) -> ("Error Out"=w2072:errorcluster, "Output"=w2068:T5[])  [unwired: 7 in]
            n1065 = Bundle By Name(cluster=w2070, "3-5.Chamber 1-1"=w2068) -> (w2069:T13)
            n1066 = property on="Chamber 1-1" class="Arr (strict)"("Value"=w2068) -> ()  [unwired: 2 in, 2 out]
          }
          event Value Change {
            n1067 = event-data() -> ("NewVal"=w2082:T5[])  [unwired: 1 in, 5 out]
            n1068 = property on="Chamber 1-2" class="Arr (strict)"() -> ("Index Values"=w2083:u32[])  [unwired: 2 in, 2 out]
            n1069 = Index Array(array=w2083, index=u32 0) -> (element=w2086:u32)
            n1070 = call "RTS Calculate Door Openings.vi"("Error In"=w2085, "Current Index"=w2086, "Input"=w2082) -> ("Error Out"=w2084:errorcluster, "Output"=w2078:T5[])  [unwired: 7 in]
            n1071 = Bundle By Name(cluster=w2080, "3-5.Chamber 1-2"=w2078) -> (w2079:T13)
            n1072 = property on="Chamber 1-2" class="Arr (strict)"("Value"=w2078) -> ()  [unwired: 2 in, 2 out]
          }
          event Value Change {
            n1073 = event-data() -> ("NewVal"=w2095:T5[])  [unwired: 1 in, 5 out]
            n1074 = property on="Chamber 1-3" class="Arr (strict)"() -> ("Index Values"=w2091:u32[])  [unwired: 2 in, 2 out]
            n1075 = Index Array(array=w2091, index=u32 0) -> (element=w2096:u32)
            n1076 = call "RTS Calculate Door Openings.vi"("Error In"=w2093, "Current Index"=w2096, "Input"=w2095) -> ("Error Out"=w2092:errorcluster, "Output"=w2088:T5[])  [unwired: 7 in]
            n1077 = Bundle By Name(cluster=w2090, "3-5.Chamber 1-3"=w2088) -> (w2089:T13)
            n1078 = property on="Chamber 1-3" class="Arr (strict)"("Value"=w2088) -> ()  [unwired: 2 in, 2 out]
          }
          event Value Change {
            n1079 = event-data() -> ("NewVal"=w2102:T5[])  [unwired: 1 in, 5 out]
            n1080 = property on="Chamber 1-1" class="Arr (strict)"() -> ("Index Values"=w2101:u32[])  [unwired: 2 in, 2 out]
            n1081 = Index Array(array=w2101, index=u32 0) -> (element=w2106:u32)
            n1082 = call "RTS Calculate Door Openings.vi"("Error In"=w2105, "Current Index"=w2106, "Input"=w2102) -> ("Error Out"=w2104:errorcluster, "Output"=w2098:T5[])  [unwired: 7 in]
            n1083 = Bundle By Name(cluster=w2100, "3-6.Chamber 1-1"=w2098) -> (w2099:T13)
            n1084 = property on="Chamber 1-1" class="Arr (strict)"("Value"=w2098) -> ()  [unwired: 2 in, 2 out]
          }
          event Value Change {
            n1085 = event-data() -> ("NewVal"=w2112:T5[])  [unwired: 1 in, 5 out]
            n1086 = property on="Chamber 1-2" class="Arr (strict)"() -> ("Index Values"=w2111:u32[])  [unwired: 2 in, 2 out]
            n1087 = Index Array(array=w2111, index=u32 0) -> (element=w2115:u32)
            n1088 = call "RTS Calculate Door Openings.vi"("Error In"=w2114, "Current Index"=w2115, "Input"=w2112) -> ("Error Out"=w2113:errorcluster, "Output"=w2108:T5[])  [unwired: 7 in]
            n1089 = Bundle By Name(cluster=w2110, "3-6.Chamber 1-2"=w2108) -> (w2109:T13)
            n1090 = property on="Chamber 1-2" class="Arr (strict)"("Value"=w2108) -> ()  [unwired: 2 in, 2 out]
          }
          event Value Change {
            n1091 = event-data() -> ("NewVal"=w2125:T5[])  [unwired: 1 in, 5 out]
            n1092 = property on="Chamber 1-3" class="Arr (strict)"() -> ("Index Values"=w2122:u32[])  [unwired: 2 in, 2 out]
            n1093 = Index Array(array=w2122, index=u32 0) -> (element=w2126:u32)
            n1094 = call "RTS Calculate Door Openings.vi"("Error In"=w2124, "Current Index"=w2126, "Input"=w2125) -> ("Error Out"=w2123:errorcluster, "Output"=w2118:T5[])  [unwired: 7 in]
            n1095 = Bundle By Name(cluster=w2120, "3-6.Chamber 1-3"=w2118) -> (w2119:T13)
            n1096 = property on="Chamber 1-3" class="Arr (strict)"("Value"=w2118) -> ()  [unwired: 2 in, 2 out]
          }
          event Value Change {
            n1097 = event-data() -> ("NewVal"=w2135:T5[])  [unwired: 1 in, 5 out]
            n1098 = property on="Chamber 1-1" class="Arr (strict)"() -> ("Index Values"=w2131:u32[])  [unwired: 2 in, 2 out]
            n1099 = Index Array(array=w2131, index=u32 0) -> (element=w2136:u32)
            n1100 = call "RTS Calculate Door Openings.vi"("Error In"=w2134, "Current Index"=w2136, "Input"=w2135) -> ("Error Out"=w2133:errorcluster, "Output"=w2128:T5[])  [unwired: 7 in]
            n1101 = Bundle By Name(cluster=w2130, "3-7.Chamber 1-1"=w2128) -> (w2129:T13)
            n1102 = property on="Chamber 1-1" class="Arr (strict)"("Value"=w2128) -> ()  [unwired: 2 in, 2 out]
          }
          event Value Change {
            n1103 = event-data() -> ("NewVal"=w2143:T5[])  [unwired: 1 in, 5 out]
            n1104 = property on="Chamber 1-2" class="Arr (strict)"() -> ("Index Values"=w2141:u32[])  [unwired: 2 in, 2 out]
            n1105 = Index Array(array=w2141, index=u32 0) -> (element=w2146:u32)
            n1106 = call "RTS Calculate Door Openings.vi"("Error In"=w2145, "Current Index"=w2146, "Input"=w2143) -> ("Error Out"=w2144:errorcluster, "Output"=w2138:T5[])  [unwired: 7 in]
            n1107 = Bundle By Name(cluster=w2140, "3-7.Chamber 1-2"=w2138) -> (w2139:T13)
            n1108 = property on="Chamber 1-2" class="Arr (strict)"("Value"=w2138) -> ()  [unwired: 2 in, 2 out]
          }
          event Value Change {
            n1109 = event-data() -> ("NewVal"=w2151:T5[])  [unwired: 1 in, 5 out]
            n1110 = property on="Chamber 1-3" class="Arr (strict)"() -> ("Index Values"=w2152:u32[])  [unwired: 2 in, 2 out]
            n1111 = Index Array(array=w2152, index=u32 0) -> (element=w2156:u32)
            n1112 = call "RTS Calculate Door Openings.vi"("Error In"=w2155, "Current Index"=w2156, "Input"=w2151) -> ("Error Out"=w2154:errorcluster, "Output"=w2148:T5[])  [unwired: 7 in]
            n1113 = Bundle By Name(cluster=w2150, "3-7.Chamber 1-3"=w2148) -> (w2149:T13)
            n1114 = property on="Chamber 1-3" class="Arr (strict)"("Value"=w2148) -> ()  [unwired: 2 in, 2 out]
          }
          event Value Change {
            n1115 = event-data() -> ("NewVal"=w2162:T5[])  [unwired: 1 in, 5 out]
            n1116 = property on="Chamber 1-1" class="Arr (strict)"() -> ("Index Values"=w2165:u32[])  [unwired: 2 in, 2 out]
            n1117 = Index Array(array=w2165, index=u32 0) -> (element=w2166:u32)
            n1118 = call "RTS Calculate Door Openings.vi"("Error In"=w2164, "Current Index"=w2166, "Input"=w2162) -> ("Error Out"=w2163:errorcluster, "Output"=w2158:T5[])  [unwired: 7 in]
            n1119 = Bundle By Name(cluster=w2160, "3-8.Chamber 1-1"=w2158) -> (w2159:T13)
            n1120 = property on="Chamber 1-1" class="Arr (strict)"("Value"=w2158) -> ()  [unwired: 2 in, 2 out]
          }
          event Value Change {
            n1121 = event-data() -> ("NewVal"=w2172:T5[])  [unwired: 1 in, 5 out]
            n1122 = property on="Chamber 1-2" class="Arr (strict)"() -> ("Index Values"=w2171:u32[])  [unwired: 2 in, 2 out]
            n1123 = Index Array(array=w2171, index=u32 0) -> (element=w2176:u32)
            n1124 = call "RTS Calculate Door Openings.vi"("Error In"=w2174, "Current Index"=w2176, "Input"=w2172) -> ("Error Out"=w2173:errorcluster, "Output"=w2168:T5[])  [unwired: 7 in]
            n1125 = Bundle By Name(cluster=w2170, "3-8.Chamber 1-2"=w2168) -> (w2169:T13)
            n1126 = property on="Chamber 1-2" class="Arr (strict)"("Value"=w2168) -> ()  [unwired: 2 in, 2 out]
          }
          event Value Change {
            n1127 = event-data() -> ("NewVal"=w2184:T5[])  [unwired: 1 in, 5 out]
            n1128 = property on="Chamber 1-3" class="Arr (strict)"() -> ("Index Values"=w2181:u32[])  [unwired: 2 in, 2 out]
            n1129 = Index Array(array=w2181, index=u32 0) -> (element=w2185:u32)
            n1130 = call "RTS Calculate Door Openings.vi"("Error In"=w2183, "Current Index"=w2185, "Input"=w2184) -> ("Error Out"=w2182:errorcluster, "Output"=w2178:T5[])  [unwired: 7 in]
            n1131 = Bundle By Name(cluster=w2180, "3-8.Chamber 1-3"=w2178) -> (w2179:T13)
            n1132 = property on="Chamber 1-3" class="Arr (strict)"("Value"=w2178) -> ()  [unwired: 2 in, 2 out]
          }
          event Value Change {
            n1133 = event-data() -> ("NewVal"=w2194:T5[])  [unwired: 1 in, 5 out]
            n1134 = property on="Chamber 1-1" class="Arr (strict)"() -> ("Index Values"=w2191:u32[])  [unwired: 2 in, 2 out]
            n1135 = Index Array(array=w2191, index=u32 0) -> (element=w2195:u32)
            n1136 = call "RTS Calculate Door Openings.vi"("Error In"=w2193, "Current Index"=w2195, "Input"=w2194) -> ("Error Out"=w2192:errorcluster, "Output"=w2188:T5[])  [unwired: 7 in]
            n1137 = Bundle By Name(cluster=w2190, "4-1.Chamber 1-1"=w2188) -> (w2189:T13)
            n1138 = property on="Chamber 1-1" class="Arr (strict)"("Value"=w2188) -> ()  [unwired: 2 in, 2 out]
          }
          event Value Change {
            n1139 = event-data() -> ("NewVal"=w2203:T5[])  [unwired: 1 in, 5 out]
            n1140 = property on="Chamber 1-2" class="Arr (strict)"() -> ("Index Values"=w2202:u32[])  [unwired: 2 in, 2 out]
            n1141 = Index Array(array=w2202, index=u32 0) -> (element=w2206:u32)
            n1142 = call "RTS Calculate Door Openings.vi"("Error In"=w2205, "Current Index"=w2206, "Input"=w2203) -> ("Error Out"=w2204:errorcluster, "Output"=w2198:T5[])  [unwired: 7 in]
            n1143 = Bundle By Name(cluster=w2200, "4-1.Chamber 1-2"=w2198) -> (w2199:T13)
            n1144 = property on="Chamber 1-2" class="Arr (strict)"("Value"=w2198) -> ()  [unwired: 2 in, 2 out]
          }
          event Value Change {
            n1145 = event-data() -> ("NewVal"=w2212:T5[])  [unwired: 1 in, 5 out]
            n1146 = property on="Chamber 1-3" class="Arr (strict)"() -> ("Index Values"=w2211:u32[])  [unwired: 2 in, 2 out]
            n1147 = Index Array(array=w2211, index=u32 0) -> (element=w2216:u32)
            n1148 = call "RTS Calculate Door Openings.vi"("Error In"=w2215, "Current Index"=w2216, "Input"=w2212) -> ("Error Out"=w2214:errorcluster, "Output"=w2208:T5[])  [unwired: 7 in]
            n1149 = Bundle By Name(cluster=w2210, "4-1.Chamber 1-3"=w2208) -> (w2209:T13)
            n1150 = property on="Chamber 1-3" class="Arr (strict)"("Value"=w2208) -> ()  [unwired: 2 in, 2 out]
          }
          event Value Change {
            n1151 = event-data() -> ("NewVal"=w2225:T5[])  [unwired: 1 in, 5 out]
            n1152 = property on="Chamber 1-1" class="Arr (strict)"() -> ("Index Values"=w2221:u32[])  [unwired: 2 in, 2 out]
            n1153 = Index Array(array=w2221, index=u32 0) -> (element=w2226:u32)
            n1154 = call "RTS Calculate Door Openings.vi"("Error In"=w2223, "Current Index"=w2226, "Input"=w2225) -> ("Error Out"=w2222:errorcluster, "Output"=w2218:T5[])  [unwired: 7 in]
            n1155 = Bundle By Name(cluster=w2220, "4-2.Chamber 1-1"=w2218) -> (w2219:T13)
            n1156 = property on="Chamber 1-1" class="Arr (strict)"("Value"=w2218) -> ()  [unwired: 2 in, 2 out]
          }
          event Value Change {
            n1157 = event-data() -> ("NewVal"=w2233:T5[])  [unwired: 1 in, 5 out]
            n1158 = property on="Chamber 1-2" class="Arr (strict)"() -> ("Index Values"=w2232:u32[])  [unwired: 2 in, 2 out]
            n1159 = Index Array(array=w2232, index=u32 0) -> (element=w2236:u32)
            n1160 = call "RTS Calculate Door Openings.vi"("Error In"=w2235, "Current Index"=w2236, "Input"=w2233) -> ("Error Out"=w2234:errorcluster, "Output"=w2228:T5[])  [unwired: 7 in]
            n1161 = property on="Chamber 1-2" class="Arr (strict)"("Value"=w2228) -> ()  [unwired: 2 in, 2 out]
            n1162 = Bundle By Name(cluster=w2230, "4-2.Chamber 1-2"=w2228) -> (w2229:T13)
          }
          event Value Change {
            n1163 = event-data() -> ("NewVal"=w2245:T5[])  [unwired: 1 in, 5 out]
            n1164 = property on="Chamber 1-3" class="Arr (strict)"() -> ("Index Values"=w2241:u32[])  [unwired: 2 in, 2 out]
            n1165 = Index Array(array=w2241, index=u32 0) -> (element=w2246:u32)
            n1166 = call "RTS Calculate Door Openings.vi"("Error In"=w2243, "Current Index"=w2246, "Input"=w2245) -> ("Error Out"=w2242:errorcluster, "Output"=w2238:T5[])  [unwired: 7 in]
            n1167 = Bundle By Name(cluster=w2240, "4-2.Chamber 1-3"=w2238) -> (w2239:T13)
            n1168 = property on="Chamber 1-3" class="Arr (strict)"("Value"=w2238) -> ()  [unwired: 2 in, 2 out]
          }
          event Value Change {
            n1169 = event-data() -> ("NewVal"=w2253:T5[])  [unwired: 1 in, 5 out]
            n1170 = property on="Chamber 1-1" class="Arr (strict)"() -> ("Index Values"=w2254:u32[])  [unwired: 2 in, 2 out]
            n1171 = Index Array(array=w2254, index=u32 0) -> (element=w2255:u32)
            n1172 = call "RTS Calculate Door Openings.vi"("Error In"=w2252, "Current Index"=w2255, "Input"=w2253) -> ("Error Out"=w2251:errorcluster, "Output"=w2248:T5[])  [unwired: 7 in]
            n1173 = Bundle By Name(cluster=w2250, "4-3.Chamber 1-1"=w2248) -> (w2249:T13)
            n1174 = property on="Chamber 1-1" class="Arr (strict)"("Value"=w2248) -> ()  [unwired: 2 in, 2 out]
          }
          event Value Change {
            n1175 = event-data() -> ("NewVal"=w2265:T5[])  [unwired: 1 in, 5 out]
            n1176 = property on="Chamber 1-2" class="Arr (strict)"() -> ("Index Values"=w2261:u32[])  [unwired: 2 in, 2 out]
            n1177 = Index Array(array=w2261, index=u32 0) -> (element=w2266:u32)
            n1178 = call "RTS Calculate Door Openings.vi"("Error In"=w2263, "Current Index"=w2266, "Input"=w2265) -> ("Error Out"=w2262:errorcluster, "Output"=w2258:T5[])  [unwired: 7 in]
            n1179 = Bundle By Name(cluster=w2260, "4-3.Chamber 1-2"=w2258) -> (w2259:T13)
            n1180 = property on="Chamber 1-2" class="Arr (strict)"("Value"=w2258) -> ()  [unwired: 2 in, 2 out]
          }
          event Value Change {
            n1181 = event-data() -> ("NewVal"=w2272:T5[])  [unwired: 1 in, 5 out]
            n1182 = property on="Chamber 1-3" class="Arr (strict)"() -> ("Index Values"=w2271:u32[])  [unwired: 2 in, 2 out]
            n1183 = Index Array(array=w2271, index=u32 0) -> (element=w2275:u32)
            n1184 = call "RTS Calculate Door Openings.vi"("Error In"=w2274, "Current Index"=w2275, "Input"=w2272) -> ("Error Out"=w2273:errorcluster, "Output"=w2268:T5[])  [unwired: 7 in]
            n1185 = property on="Chamber 1-3" class="Arr (strict)"("Value"=w2268) -> ()  [unwired: 2 in, 2 out]
            n1186 = Bundle By Name(cluster=w2270, "4-3.Chamber 1-3"=w2268) -> (w2269:T13)
          }
          event Value Change {
            n1187 = event-data() -> ("NewVal"=w2283:T5[])  [unwired: 1 in, 5 out]
            n1188 = property on="Chamber 1-1" class="Arr (strict)"() -> ("Index Values"=w2281:u32[])  [unwired: 2 in, 2 out]
            n1189 = Index Array(array=w2281, index=u32 0) -> (element=w2286:u32)
            n1190 = call "RTS Calculate Door Openings.vi"("Error In"=w2285, "Current Index"=w2286, "Input"=w2283) -> ("Error Out"=w2284:errorcluster, "Output"=w2278:T5[])  [unwired: 7 in]
            n1191 = property on="Chamber 1-1" class="Arr (strict)"("Value"=w2278) -> ()  [unwired: 2 in, 2 out]
            n1192 = Bundle By Name(cluster=w2280, "4-4.Chamber 1-1"=w2278) -> (w2279:T13)
          }
          event Value Change {
            n1193 = event-data() -> ("NewVal"=w2295:T5[])  [unwired: 1 in, 5 out]
            n1194 = property on="Chamber 1-2" class="Arr (strict)"() -> ("Index Values"=w2291:u32[])  [unwired: 2 in, 2 out]
            n1195 = Index Array(array=w2291, index=u32 0) -> (element=w2296:u32)
            n1196 = call "RTS Calculate Door Openings.vi"("Error In"=w2293, "Current Index"=w2296, "Input"=w2295) -> ("Error Out"=w2292:errorcluster, "Output"=w2288:T5[])  [unwired: 7 in]
            n1197 = Bundle By Name(cluster=w2290, "4-4.Chamber 1-2"=w2288) -> (w2289:T13)
            n1198 = property on="Chamber 1-2" class="Arr (strict)"("Value"=w2288) -> ()  [unwired: 2 in, 2 out]
          }
          event Value Change {
            n1199 = event-data() -> ("NewVal"=w2304:T5[])  [unwired: 1 in, 5 out]
            n1200 = property on="Chamber 1-3" class="Arr (strict)"() -> ("Index Values"=w2301:u32[])  [unwired: 2 in, 2 out]
            n1201 = Index Array(array=w2301, index=u32 0) -> (element=w2305:u32)
            n1202 = call "RTS Calculate Door Openings.vi"("Error In"=w2303, "Current Index"=w2305, "Input"=w2304) -> ("Error Out"=w2302:errorcluster, "Output"=w2298:T5[])  [unwired: 7 in]
            n1203 = property on="Chamber 1-3" class="Arr (strict)"("Value"=w2298) -> ()  [unwired: 2 in, 2 out]
            n1204 = Bundle By Name(cluster=w2300, "4-4.Chamber 1-3"=w2298) -> (w2299:T13)
          }
          event Value Change {
            n1205 = event-data() -> ("NewVal"=w2313:T5[])  [unwired: 1 in, 5 out]
            n1206 = property on="Chamber 1-1" class="Arr (strict)"() -> ("Index Values"=w2311:u32[])  [unwired: 2 in, 2 out]
            n1207 = Index Array(array=w2311, index=u32 0) -> (element=w2316:u32)
            n1208 = call "RTS Calculate Door Openings.vi"("Error In"=w2315, "Current Index"=w2316, "Input"=w2313) -> ("Error Out"=w2314:errorcluster, "Output"=w2308:T5[])  [unwired: 7 in]
            n1209 = Bundle By Name(cluster=w2310, "4-5.Chamber 1-1"=w2308) -> (w2309:T13)
            n1210 = property on="Chamber 1-1" class="Arr (strict)"("Value"=w2308) -> ()  [unwired: 2 in, 2 out]
          }
          event Value Change {
            n1211 = event-data() -> ("NewVal"=w2325:T5[])  [unwired: 1 in, 5 out]
            n1212 = property on="Chamber 1-2" class="Arr (strict)"() -> ("Index Values"=w2321:u32[])  [unwired: 2 in, 2 out]
            n1213 = Index Array(array=w2321, index=u32 0) -> (element=w2326:u32)
            n1214 = call "RTS Calculate Door Openings.vi"("Error In"=w2323, "Current Index"=w2326, "Input"=w2325) -> ("Error Out"=w2322:errorcluster, "Output"=w2318:T5[])  [unwired: 7 in]
            n1215 = property on="Chamber 1-2" class="Arr (strict)"("Value"=w2318) -> ()  [unwired: 2 in, 2 out]
            n1216 = Bundle By Name(cluster=w2320, "4-5.Chamber 1-2"=w2318) -> (w2319:T13)
          }
          event Value Change {
            n1217 = event-data() -> ("NewVal"=w2335:T5[])  [unwired: 1 in, 5 out]
            n1218 = property on="Chamber 1-3" class="Arr (strict)"() -> ("Index Values"=w2331:u32[])  [unwired: 2 in, 2 out]
            n1219 = Index Array(array=w2331, index=u32 0) -> (element=w2336:u32)
            n1220 = call "RTS Calculate Door Openings.vi"("Error In"=w2333, "Current Index"=w2336, "Input"=w2335) -> ("Error Out"=w2332:errorcluster, "Output"=w2328:T5[])  [unwired: 7 in]
            n1221 = property on="Chamber 1-3" class="Arr (strict)"("Value"=w2328) -> ()  [unwired: 2 in, 2 out]
            n1222 = Bundle By Name(cluster=w2330, "4-5.Chamber 1-3"=w2328) -> (w2329:T13)
          }
          event Value Change {
            n1223 = event-data() -> ("NewVal"=w2342:T5[])  [unwired: 1 in, 5 out]
            n1224 = property on="Chamber 1-1" class="Arr (strict)"() -> ("Index Values"=w2341:u32[])  [unwired: 2 in, 2 out]
            n1225 = Index Array(array=w2341, index=u32 0) -> (element=w2345:u32)
            n1226 = call "RTS Calculate Door Openings.vi"("Error In"=w2344, "Current Index"=w2345, "Input"=w2342) -> ("Error Out"=w2343:errorcluster, "Output"=w2338:T5[])  [unwired: 7 in]
            n1227 = Bundle By Name(cluster=w2340, "4-6.Chamber 1-1"=w2338) -> (w2339:T13)
            n1228 = property on="Chamber 1-1" class="Arr (strict)"("Value"=w2338) -> ()  [unwired: 2 in, 2 out]
          }
          event Value Change {
            n1229 = event-data() -> ("NewVal"=w2355:T5[])  [unwired: 1 in, 5 out]
            n1230 = property on="Chamber 1-2" class="Arr (strict)"() -> ("Index Values"=w2351:u32[])  [unwired: 2 in, 2 out]
            n1231 = Index Array(array=w2351, index=u32 0) -> (element=w2356:u32)
            n1232 = call "RTS Calculate Door Openings.vi"("Error In"=w2353, "Current Index"=w2356, "Input"=w2355) -> ("Error Out"=w2352:errorcluster, "Output"=w2348:T5[])  [unwired: 7 in]
            n1233 = Bundle By Name(cluster=w2350, "4-6.Chamber 1-2"=w2348) -> (w2349:T13)
            n1234 = property on="Chamber 1-2" class="Arr (strict)"("Value"=w2348) -> ()  [unwired: 2 in, 2 out]
          }
          event Value Change {
            n1235 = event-data() -> ("NewVal"=w2363:T5[])  [unwired: 1 in, 5 out]
            n1236 = property on="Chamber 1-3" class="Arr (strict)"() -> ("Index Values"=w2362:u32[])  [unwired: 2 in, 2 out]
            n1237 = Index Array(array=w2362, index=u32 0) -> (element=w2366:u32)
            n1238 = call "RTS Calculate Door Openings.vi"("Error In"=w2365, "Current Index"=w2366, "Input"=w2363) -> ("Error Out"=w2364:errorcluster, "Output"=w2358:T5[])  [unwired: 7 in]
            n1239 = Bundle By Name(cluster=w2360, "4-6.Chamber 1-3"=w2358) -> (w2359:T13)
            n1240 = property on="Chamber 1-3" class="Arr (strict)"("Value"=w2358) -> ()  [unwired: 2 in, 2 out]
          }
          event Value Change {
            n1241 = event-data() -> ("NewVal"=w2375:T5[])  [unwired: 1 in, 5 out]
            n1242 = property on="Chamber 1-1" class="Arr (strict)"() -> ("Index Values"=w2372:u32[])  [unwired: 2 in, 2 out]
            n1243 = Index Array(array=w2372, index=u32 0) -> (element=w2376:u32)
            n1244 = call "RTS Calculate Door Openings.vi"("Error In"=w2374, "Current Index"=w2376, "Input"=w2375) -> ("Error Out"=w2373:errorcluster, "Output"=w2368:T5[])  [unwired: 7 in]
            n1245 = Bundle By Name(cluster=w2370, "4-7.Chamber 1-1"=w2368) -> (w2369:T13)
            n1246 = property on="Chamber 1-1" class="Arr (strict)"("Value"=w2368) -> ()  [unwired: 2 in, 2 out]
          }
          event Value Change {
            n1247 = event-data() -> ("NewVal"=w2384:T5[])  [unwired: 1 in, 5 out]
            n1248 = property on="Chamber 1-2" class="Arr (strict)"() -> ("Index Values"=w2381:u32[])  [unwired: 2 in, 2 out]
            n1249 = Index Array(array=w2381, index=u32 0) -> (element=w2386:u32)
            n1250 = call "RTS Calculate Door Openings.vi"("Error In"=w2383, "Current Index"=w2386, "Input"=w2384) -> ("Error Out"=w2382:errorcluster, "Output"=w2378:T5[])  [unwired: 7 in]
            n1251 = Bundle By Name(cluster=w2380, "4-7.Chamber 1-2"=w2378) -> (w2379:T13)
            n1252 = property on="Chamber 1-2" class="Arr (strict)"("Value"=w2378) -> ()  [unwired: 2 in, 2 out]
          }
          event Value Change {
            n1253 = event-data() -> ("NewVal"=w2394:T5[])  [unwired: 1 in, 5 out]
            n1254 = property on="Chamber 1-3" class="Arr (strict)"() -> ("Index Values"=w2391:u32[])  [unwired: 2 in, 2 out]
            n1255 = Index Array(array=w2391, index=u32 0) -> (element=w2396:u32)
            n1256 = call "RTS Calculate Door Openings.vi"("Error In"=w2393, "Current Index"=w2396, "Input"=w2394) -> ("Error Out"=w2392:errorcluster, "Output"=w2388:T5[])  [unwired: 7 in]
            n1257 = Bundle By Name(cluster=w2390, "4-7.Chamber 1-3"=w2388) -> (w2389:T13)
            n1258 = property on="Chamber 1-3" class="Arr (strict)"("Value"=w2388) -> ()  [unwired: 2 in, 2 out]
          }
          event Value Change {
            n1259 = event-data() -> ("NewVal"=w2405:T5[])  [unwired: 1 in, 5 out]
            n1260 = property on="Chamber 1-1" class="Arr (strict)"() -> ("Index Values"=w2401:u32[])  [unwired: 2 in, 2 out]
            n1261 = Index Array(array=w2401, index=u32 0) -> (element=w2406:u32)
            n1262 = call "RTS Calculate Door Openings.vi"("Error In"=w2403, "Current Index"=w2406, "Input"=w2405) -> ("Error Out"=w2402:errorcluster, "Output"=w2398:T5[])  [unwired: 7 in]
            n1263 = Bundle By Name(cluster=w2400, "4-8.Chamber 1-1"=w2398) -> (w2399:T13)
            n1264 = property on="Chamber 1-1" class="Arr (strict)"("Value"=w2398) -> ()  [unwired: 2 in, 2 out]
          }
          event Value Change {
            n1265 = event-data() -> ("NewVal"=w2414:T5[])  [unwired: 1 in, 5 out]
            n1266 = property on="Chamber 1-2" class="Arr (strict)"() -> ("Index Values"=w2411:u32[])  [unwired: 2 in, 2 out]
            n1267 = Index Array(array=w2411, index=u32 0) -> (element=w2416:u32)
            n1268 = call "RTS Calculate Door Openings.vi"("Error In"=w2413, "Current Index"=w2416, "Input"=w2414) -> ("Error Out"=w2412:errorcluster, "Output"=w2408:T5[])  [unwired: 7 in]
            n1269 = Bundle By Name(cluster=w2410, "4-8.Chamber 1-2"=w2408) -> (w2409:T13)
            n1270 = property on="Chamber 1-2" class="Arr (strict)"("Value"=w2408) -> ()  [unwired: 2 in, 2 out]
          }
          event Value Change {
            n1271 = event-data() -> ("NewVal"=w2422:T5[])  [unwired: 1 in, 5 out]
            n1272 = property on="Chamber 1-3" class="Arr (strict)"() -> ("Index Values"=w2421:u32[])  [unwired: 2 in, 2 out]
            n1273 = Index Array(array=w2421, index=u32 0) -> (element=w2426:u32)
            n1274 = call "RTS Calculate Door Openings.vi"("Error In"=w2424, "Current Index"=w2426, "Input"=w2422) -> ("Error Out"=w2423:errorcluster, "Output"=w2418:T5[])  [unwired: 7 in]
            n1275 = Bundle By Name(cluster=w2420, "4-8.Chamber 1-3"=w2418) -> (w2419:T13)
            n1276 = property on="Chamber 1-3" class="Arr (strict)"("Value"=w2418) -> ()  [unwired: 2 in, 2 out]
          }
        }
      }
      frame "---------- Core ----------" {
        # "Do not put any code in this frame.\n(it is a separator no-op)"
        n1277 = call <vilib>:"Add State(s) to Queue__jki_lib_state_machine.vi"("State(s) in (\"\")"=w2431) -> ("States Out"=w2430:string)  [unwired: 14 in]
      }
      frame Default {
        w2441 = 42 items=["No error", "Argument error", "Memory is full", "Out of zone", "End of file", "File already open", "Generic file I/O error", "File not found", "File permission error", "Disk is full", "Duplicate path", "Too many files open", "System feature not enabled", "Resource file not found", "Cannot add resource", "Resource not found", "Image not found", "Image memory error", "Pen does not exist", "Config type invalid", "Config token not found", "Config parse error", "Config memory error", "Bad external code format", "Bad external code offset", "External code not present", "Null window", "Destroy window error", "Null menu", "Print aborted", "Bad print record", "Print driver error", "Windows error during printing", "Memory error during printing", "Print dialog error", "Generic print error", "Invalid device refnum", "Device not found", "Device parameter error", "Device unit error", "Cannot open device", "Device call aborted", "Generic error", "Cancelled by user", "Object ID too low", "Object ID too high", "Object not in heap", "Unknown heap", "Unknown object (invalid DefProc)", "Unknown object (DefProc not in table)", "Message out of range", "Invalid (null) method", "Unknown message", "Manager call not supported", "Bad address", "Network operation in progress", "Network operation timed out", "Connection is busy", "Network attribute not supported", "Network error", "Address in use", "System out of memory", "Connection aborted", "Connection refused", "Not connected", "Already connected", "Connection closed", "Initialization error (interapplication manager)", "Bad occurrence", "Wait on unbound occurrence handler", "Occurrence queue overflow", "Datalog type conflict", "Unused", "Unrecognized type (interapplication manager)", "Memory corrupt", "Failed to make temporary DLL", "Old CIN version", "Drag socket not found", "Failed to load drop-object", "Failed to register OLE object", "Failed to release OLE object", "Format specifier type mismatch", "Unknown format specifier", "Too few format specifiers", "Too many format specifiers", "Scan failed", "Newer CIN version", "Error converting to variant", "Runtime menu error", "Password tampered", "Variant attribute not found", "Incompatible variant data type", "Event data is not available", "Event Store is not present", "Occurrence is not found", "Event Queue is not created", "Event info is not available", "Refnum passed is NULL", "Error retrieving Class GUID", "Error retrieving CoClass GUID", "Error retrieving TypeLib GUID.", "Bad built application magic bytes.", "Specific driver is different from the specific driver associated with the Logical Name.", "There is no session opened to the class driver.", "Max Error", "MAX - Error with config objects", "MAX - Error loading configuration", "MAX - Group not supported"]
        # "Current State"
        # "Do not delete, rename, or modify this frame.\n(this is used to capture unhandled states and typos)"
        # "Handle mistyped state name (developer tool)"
        n1278 = Format Into String(format string="Software Exception: Unhandled State \"%s\"." ("message"), error in=w2437, w2432) -> (resulting string=w2440:string, error out=w2439:errorcluster)  [unwired: 1 in]
        n1279 = call <vilib>:"Error Cluster From Error Code.vi"("show call chain? (False)"=TRUE, "error in (no error)"=w2439, "error message (\"\")"=w2440, "error code (0)"=w2441) -> ("error out"=w2438:errorcluster)  [unwired: 5 in]
        n1280 = call <vilib>:"Add State(s) to Queue__jki_lib_state_machine.vi"("State(s) in (\"\")"=w2436) -> ("States Out"=w2435:string)  [unwired: 14 in]
      }
      frame "Initialize Core Data" {
        # "Do not delete, rename, or modify this frame.\n(this is used to determine panel behavior on exit)"
        # "originally closed?"
        # "exe?"
        # "If panel starts closed or is an EXE, then close it when we exit"
        n1281 = property class="VI"() -> ("Front Panel.Open"=w2450:bool)  [unwired: 2 in, 2 out]
        n1282 = property class="App"() -> ("App.Kind"=w2449:T11)  [unwired: 2 in, 2 out]
        n1283 = control-ref of="Current VI Reference"() -> (w2443:refnum<vi>)
        n1284 = Not(x=w2450) -> (.not. x?=w2447:bool)
        n1285 = Equal?(x=w2449, y=T11."Run Time System" ("Application:Kind")) -> (x = y?=w2446:bool)
        n1286 = Or(x=w2447, y=w2446) -> (x .or. y?=w2444:bool)
        n1287 = Bundle By Name(cluster=w2445, "Core.Current VI Reference"=w2443, "Core.Close Panel on Exit?"=w2444) -> (w2452:T13)
        n1288 = call <vilib>:"Add State(s) to Queue__jki_lib_state_machine.vi"("State(s) in (\"\")"=w2454) -> ("States Out"=w2453:string)  [unwired: 14 in]
      }
      frame "Error Handler" {
        # "Unhandled Error -- Display it"
        # "Handle any errors here.\nYou can also output any states to clean-up after errors occur"
        # "Clear error"
        n1289 = call <vilib>:"General Error Handler.vi"("error in (no error)"=w2456) -> ()  [unwired: 10 in, 5 out]
        n1290 = call <vilib>:"Add State(s) to Queue__jki_lib_state_machine.vi"("State(s) in Front (\"\")"="/* Post Error States", "State(s) in (\"\")"=w2460) -> ("States Out"=w2459:string)  [unwired: 13 in]
      }
      frame "Exit" {
        # "Do not put any code in this frame.\n(No errors that occur here will be handled.)"
        n1291 = call <vilib>:"Add State(s) to Queue__jki_lib_state_machine.vi"("State(s) in (\"\")"=w2465) -> ("States Out"=w2464:string)  [unwired: 14 in]
      }
      frame "---------- Data ----------" {
        # "Do not put any code in this frame.\n(It is a separator no-op. You can make a copy of this frame to create a new Data frame)"
        n1292 = call <vilib>:"Add State(s) to Queue__jki_lib_state_machine.vi"("State(s) in (\"\")"=w2469) -> ("States Out"=w2468:string)  [unwired: 14 in]
      }
      frame "Data: Initialize" {
        w2470 = FALSE  # Update Server
        w2504 = ""  # End Time
        w2505 = T14 {"Current VI Reference"=refnum, "Close Panel on Exit?"=FALSE}  # Core
        w2506 = ""  # Start Time
        n1293 = Bundle("Core"=w2505, "Start Time"=w2506, "End Time"=w2504, "Station Settings"="Station Settings", "1-1"="1-1", "1-2"="1-2", "1-3"="1-3", "1-4"="1-4", "1-5"="1-5", "1-6"="1-6", "1-7"="1-7", "1-8"="1-8", "2-1"="2-1", "2-2"="2-2", "2-3"="2-3", "2-4"="2-4", "2-5"="2-5", "2-6"="2-6", "2-7"="2-7", "2-8"="2-8", "3-1"="3-1", "3-2"="3-2", "3-3"="3-3", "3-4"="3-4", "3-5"="3-5", "3-6"="3-6", "3-7"="3-7", "3-8"="3-8", "4-1"="4-1", "4-2"="4-2", "4-3"="4-3", "4-4"="4-4", "4-5"="4-5", "4-6"="4-6", "4-7"="4-7", "4-8"="4-8", "Update Server"=w2470) -> (w2508:T13)  [unwired: 1 in]
        n1294 = call <vilib>:"Add State(s) to Queue__jki_lib_state_machine.vi"("State(s) in (\"\")"=w2510) -> ("States Out"=w2509:string)  [unwired: 14 in]
      }
      frame "Data: Cleanup" {
        # "Cleanup any data and references, here.\n(this is called automatically, by the Macro: Exit)"
        n1295 = Unbundle By Name(w2511) -> ("Core.Current VI Reference"=w2514:refnum<vi>)
        n1296 = Close Reference(reference=w2514, error in (no error)=w2513) -> (error out=w2512:errorcluster)
        n1297 = call <vilib>:"Add State(s) to Queue__jki_lib_state_machine.vi"("State(s) in (\"\")"=w2516) -> ("States Out"=w2515:string)  [unwired: 14 in]
      }
      frame "---------- UI ----------" {
        # "Do not put any code in this frame.\n(It is a separator no-op. You can make a copy of this frame to create a new UI frame)"
        n1298 = call <vilib>:"Add State(s) to Queue__jki_lib_state_machine.vi"("State(s) in (\"\")"=w2520) -> ("States Out"=w2519:string)  [unwired: 14 in]
      }
      frame "UI: Initialize" {
        # "Initialize the User Interface, here.\n(this is called automatically, by the Macro: Init)"
        n1299 = call <vilib>:"Add State(s) to Queue__jki_lib_state_machine.vi"("State(s) in (\"\")"=w2524) -> ("States Out"=w2523:string)  [unwired: 14 in]
      }
      frame "UI: Cursor Set" {
        # "Argument"
        # "Set and Unset Cursor Busy.\n(Usage: \"UI: Cursor Set >> Busy|Idle\")"
        n1300 = case shown="\"Idle\", Default" w2525 {
          tunnel: w2527 -> [w2532 w2534]
          tunnel: [w2531 w2533] -> w2526
          frame "Idle", Default {
            n1301 = call <vilib>:"Unset Busy.vi"("error in (no error)"=w2532) -> ("error out"=w2531:errorcluster)  [unwired: 10 in]
          }
          frame "Busy" {
            n1302 = call <vilib>:"Set Busy.vi"("error in (no error)"=w2534) -> ("error out"=w2533:errorcluster)  [unwired: 9 in, 1 out]
          }
        }
        n1303 = call <vilib>:"Add State(s) to Queue__jki_lib_state_machine.vi"("State(s) in (\"\")"=w2530) -> ("States Out"=w2529:string)  [unwired: 14 in]
      }
      frame "Read Current Files" {
        n1304 = disable-structure shown="Disabled" {
          frame Disabled {
            n1305 = To Time Stamp() -> (0:→"time stamp":timestamp)  [unwired: 1 in]
          }
          frame Enabled {
          }
        }
        n1306 = call <vilib>:"Add State(s) to Queue__jki_lib_state_machine.vi"("State(s) in (\"\")"=w2538) -> ("States Out"=w2537:string)  [unwired: 14 in]
      }
      frame "Write Current File" {
        n1307 = call <vilib>:"Add State(s) to Queue__jki_lib_state_machine.vi"("State(s) in (\"\")"=w2543) -> ("States Out"=w2542:string)  [unwired: 14 in]
      }
      frame "UI: Front Panel State" {
        # "Argument"
        # "Set Front Panel Open or Closed\n(Usage: \"UI: Front Panel State >> Open|Close\")"
        n1308 = Unbundle By Name(w2546) -> ("Core.Current VI Reference"=w2545:refnum<vi>)
        n1309 = case shown="\"Open\", Default" w2544 {
          tunnel: w2548 -> [w2554 w2567]
          tunnel: [w2556 w2568] -> w2547
          tunnel: w2545 -> [w2555 w2565]
          frame "Open", Default {
            n1310 = property class="VI"(reference=w2555, error in=w2554) -> (reference out=w2552:refnum<vi>, error out=w2553:errorcluster, "Front Panel.Open"=w2551:bool)
            n1311 = case shown="False" w2551 {
              tunnel: [w2559 w2562] -> w2556
              tunnel: w2553 -> [w2558 w2562]
              tunnel: w2552 -> [w2557 _]
              frame False {
                n1312 = invoke class="VI" method="FP.Open"(reference=w2557, error in=w2558, "Activate"=TRUE, "State"=T12."Standard") -> (error out=w2559:errorcluster)  [unwired: 1 in, 4 out]
              }
              frame True {
              }
            }
          }
          frame "Close" {
            n1313 = property class="VI"(reference=w2565, error in=w2567) -> (reference out=w2564:refnum<vi>, error out=w2566:errorcluster, "Front Panel.Open"=w2563:bool)
            n1314 = case shown="True" w2563 {
              tunnel: [w2569 w2572] -> w2568
              tunnel: w2566 -> [w2569 w2571]
              tunnel: w2564 -> [_ w2570]
              frame False {
              }
              frame True {
                n1315 = invoke class="VI" method="FP.Close"(reference=w2570, error in=w2571) -> (error out=w2572:errorcluster)  [unwired: 1 in, 2 out]
              }
            }
          }
        }
        n1316 = call <vilib>:"Add State(s) to Queue__jki_lib_state_machine.vi"("State(s) in (\"\")"=w2550) -> ("States Out"=w2549:string)  [unwired: 14 in]
      }
      frame "---------- Macro ----------" {
        # "Do not put any code in this frame.\n(It is a separator no-op. You can make a copy of this frame to create a new Macro frame)"
        n1317 = call <vilib>:"Add State(s) to Queue__jki_lib_state_machine.vi"("State(s) in (\"\")"=w2576) -> ("States Out"=w2575:string)  [unwired: 14 in]
      }
      frame "Macro: Initialize" {
        w2577 = "Data: Initialize\nInitialize Core Data\nUI: Initialize\nUI: Front Panel State >> Open"  # Data: Initialize Initialize Core Data UI: Initialize UI: Front Panel State >> Open
        # "Initialization Macro\n(This is called once, when the VI starts)"
        n1318 = call <vilib>:"Add State(s) to Queue__jki_lib_state_machine.vi"("State(s) in Front (\"\")"=w2577, "State(s) in (\"\")"=w2581) -> ("States Out"=w2580:string)  [unwired: 13 in]
      }
      frame "Macro: Exit" {
        # "Exit Macro\n(This is called once, when the VI exits)"
        n1319 = Unbundle By Name(w2588) -> ("Core.Close Panel on Exit?"=w2587:bool)
        n1320 = Select(t="UI: Front Panel State >> Close", s=w2587, f="") -> (s? t:f=w2584:string)
        n1321 = call <vilib>:"Add State(s) to Queue__jki_lib_state_machine.vi"("State(s) in (\"\")"=w2584, "State(s) at Back (\"\")"="Data: Cleanup\nExit") -> ("States Out"=w2582:string)  [unwired: 13 in]
        n1322 = call <vilib>:"Add State(s) to Queue__jki_lib_state_machine.vi"("State(s) in Front (\"\")"=w2582, "State(s) in (\"\")"=w2591) -> ("States Out"=w2590:string)  [unwired: 13 in]
      }
      frame "---------- New Category ----------" {
        # "Template Separator\n(You can make a copy of, or modify, this frame)"
        n1323 = call <vilib>:"Add State(s) to Queue__jki_lib_state_machine.vi"("State(s) in (\"\")"=w2595) -> ("States Out"=w2594:string)  [unwired: 14 in]
      }
      frame "Get Start Stop Times" {
        n1324 = disable-structure shown="Disabled" {
          disable-tunnel: w2597 -> [w2613 _]
          disable-tunnel: [w2612 _] -> w2596
          frame Disabled {
            n1325 = Get Date/Time String(want seconds? (F)=TRUE) -> (seconds (now)=w2614:timestamp, date string=w2606:string, time string=w2605:string)  [unwired: 1 in]
            n1326 = Get Date/Time String(want seconds? (F)=TRUE) -> (seconds (now)=w2608:timestamp, date string=w2603:string, time string=w2604:string)  [unwired: 1 in]
            n1327 = call <vilib>:"Space Constant.vi"() -> ("String"=w2610:string)
            n1328 = call <vilib>:"Space Constant.vi"() -> ("String"=w2609:string)
            n1329 = Concatenate Strings(w2605, w2610, w2606) -> (w2611:string)
            n1330 = Concatenate Strings(w2604, w2609, w2603) -> (w2607:string)
            n1331 = Bundle By Name(cluster=w2613, "Start Time"=w2611, "End Time"=w2607) -> (w2612:T13)
          }
          frame Enabled {
          }
        }
        n1332 = call <vilib>:"Add State(s) to Queue__jki_lib_state_machine.vi"("State(s) in (\"\")"=w2600) -> ("States Out"=w2599:string)  [unwired: 14 in]
      }
      frame "Get Pattern" {
        # "Use this to write the text file for the server"
        n1333 = Unbundle By Name(w2616) -> ("Start Time"=w2618:string, "End Time"=w2617:string)
        n1334 = Build Array(w2618, w2617) -> ()  [unwired: 1 out]
        n1335 = call <vilib>:"Add State(s) to Queue__jki_lib_state_machine.vi"("State(s) in (\"\")"=w2620) -> ("States Out"=w2619:string)  [unwired: 14 in]
      }
    }
    n1336 = case shown="True" "Debug" {
      tunnel: w13 -> [_ w27]
      tunnel: w12 -> [w24 w26]
      tunnel: [w24 w25] -> w11
      frame False {
      }
      frame True {
        n1337 = Build Array (concatenate)(w26, w27) -> (w25:string[])
        "Debug array" <- w25
      }
    }
  }
  "Error Out" <- w5
  n1338 = Unbundle By Name(w3) -> ("Update Server"=→"Update Server Output":bool)
